vi "DL-SMART-MS-Modify-05-25-7.0.vi"() -> ()   [LabVIEW 2013]
uses:
  <vilib>/Utility/file.llb/Read From Spreadsheet File (DBL).vi
  <userlib>/caLab/Private/CaLabEvent_PV-1D.vi
  <userlib>/caLab/Private/Put_DBL-1D_PV.vi
  <userlib>/caLab/Private/Put_I32_PV.vi
  cal_p.vi
  <userlib>/caLab/Private/Get_PV.vi
  <vilib>/Utility/file.llb/Write To Spreadsheet File (DBL).vi
  <vilib>/vision/driver/NI_Vision_Acquisition_Software.lvlib
  <resource>/objmgr/imaqdx.rc
  <vilib>/Analysis/NI_AALPro.lvlib
panel:
  out "idn status":string
  out "MS":cluster{dbl[], "filtered data":dbl[]}(graph)
  out "std sample":T1(array[cluster])
  in  "Set Laser":bool
  out "Image":T2(plugin-control)
  out "selected id":i32
  out "selected row":i32
  out "currentNO":string
  out "commet":string
  out "sampleID":string
  in  "Shots/Point":i32=100
  in  "chamber in":bool caption="TakeMS"
  in  "chamber out":bool caption="TakeMS"
  in  "Laser parameter":T4
  in  "ADC parameter":T5
  in  "ShutDownSystem":bool
  in  "ADC reference":refnum<vi>
  in  "SetLaserEnergy":dbl(slide) min=0.0 max=50.0 scale=0.0..10.0
  in  "LaserHV":u8=50 min=1 max=100
  in  "频率/Hz":u8=30
  out "Pul.HV-Real":dbl
  out "Identify Spcetrum":cluster{"ID1:X":dbl[], "ID1:Y":dbl[]}[](graph)
  in  "测试记录":i32(listbox)=6
  in  "Identification Results (单靶鉴定结果)":i32(listbox)=2
  in  "HVEnable":bool
  out "GateClose":bool
  out "LaserOK":bool
  out "HV-OK":bool
  out "Vacuum-OK":bool
  in  "Tab Control":T6(tab)
  in  "helix-Zeta-Step":dbl=100.0
  in  "helix-b":dbl=0.2
  in  "AcquireMS-Methods":u8(ring) items=["SinglePoint", "Multipoints", "MultiTar"]
  in  "Thresh":dbl=-0.005 format="%#_13g"
  in  "right rank":i32=2
  in  "left rank":i32=2
  in  "deBaseline":bool
  in  "MCPHV-Set":dbl=1400.0 min=0.0 max=1600.0
  in  "LensHV-Set":dbl=8000.0 min=0.0 max=10000.0
  in  "Tar.HV-Set":dbl=18010.0 min=0.0 max=20000.0
  in  "Pul.HV-Set":dbl=1400.0 min=0.0 max=2000.0
  in  "PulseDelay":dbl
  in  "ADCFreq":dbl
  in  "CH1_Coupling":u64(ring)=2 items=["Volt DC"=1, "Volt AC"=2, "Ampere DC"=4, "Ampere AC"=8, "Ohm"=16]
  in  "Channel 1_Range":dbl(ring)=4.0 items=["80 V"=80.0, "40 V"=40.0, "20 V"=20.0, "8 V"=8.0, "4 V"=4.0, "2 V"=2.0, "800 mV"=0.8, "400 mV"=0.4, "200 mV"=0.2]
  in  "Anal. Setting File":string="High Mass"
  in  "SettingFileSave":bool caption="TakeMS"
  in  "SettingFileAppl":bool caption="TakeMS"
  in  "SettingDel":bool caption="TakeMS"
  in  "RunADC":bool caption="TakeMS"
  out "ADCstatus":bool
  in  "Vac_Prot.":bool
  in  "Turbo_Fore":bool
  in  "Main_Samp":bool
  in  "Samp_Atmos":bool
  in  "Fore_Samp":bool
  in  "StartPump":bool
  in  "SopPump":bool
  out "TurboSpeed":dbl(knob) scale=0.0..100.0
  out "PumpKW":dbl
  out "PumpAmps":dbl
  out "PumpTemp":u16
  out "PumpVolts":dbl
  in  "laser OFF":bool
  in  "laser ON":bool
  out "cluster":T7
  in  "laser Deactive":bool
  out "A1-position-Y":dbl=45.0 caption="Y" min=0.0 max=55.0
  out "A1-position-X":dbl=53.4 caption="X" min=0.0 max=55.0
  in  "GO":bool
  in  "Y":dbl min=0.0 max=55.0
  in  "X":dbl min=0.0 max=55.0
  in  "A1-Position":bool caption="X-"
  in  "Plat_To_Zero":bool caption="TakeMS"
  in  "Plat_Cal":bool caption="TakeMS"
  out "Y当前":dbl
  out "X当前":dbl
  out "移动":bool
  out "Y满":bool
  out "Y标":bool
  out "X满":bool
  out "Y0":bool
  out "X0":bool
  out "靶位In/Out":bool
  out "仓门":bool
  out "Y过热":bool
  out "X过热":bool
  out "通讯":bool
  in  "Operation Record":i32(listbox)
  in  "OptionRecordLoad 2":bool caption="TakeMS"
  in  "OptionRecordClear":bool caption="TakeMS"
  out "c:":dbl
  out "b:":dbl
  out "a:":dbl
  in  "cancel cal":bool
  in  "cal save":bool
  in  "peak cal":bool
  in  "peak detect":bool
  in  "标准样品":u16(ring) items=["肺炎克雷伯菌", "铜绿假单胞菌"]
  in  "定标参数":i32(listbox)
  out "Tar.HV-Real":dbl
  out "LensHV-Real":dbl
  out "MCPHV-Real":dbl
  out "Lvaccum":dbl=0.83 format="%#_2e"
  out "Hvaccum":dbl=3.4e-05 format="%#_2e"
  in  "H12":bool
  in  "G12":bool
  in  "F12":bool
  in  "E12":bool
  in  "D12":bool
  in  "C12":bool
  in  "B12":bool
  in  "A12":bool
  in  "H11":bool
  in  "G11":bool
  in  "F11":bool
  in  "E11":bool
  in  "D11":bool
  in  "C11":bool
  in  "B11":bool
  in  "A11":bool
  in  "H10":bool
  in  "G10":bool
  in  "F10":bool
  in  "E10":bool
  in  "D10":bool
  in  "C10":bool
  in  "B10":bool
  in  "A10":bool
  in  "H9":bool
  in  "G9":bool
  in  "F9":bool
  in  "E9":bool
  in  "D9":bool
  in  "C9":bool
  in  "B9":bool
  in  "A9":bool
  in  "H8":bool
  in  "G8":bool
  in  "F8":bool
  in  "E8":bool
  in  "D8":bool
  in  "C8":bool
  in  "B8":bool
  in  "A8":bool
  in  "H7":bool
  in  "G7":bool
  in  "F7":bool
  in  "E7":bool
  in  "D7":bool
  in  "C7":bool
  in  "B7":bool
  in  "A7":bool
  in  "H6":bool
  in  "G6":bool
  in  "F6":bool
  in  "E6":bool
  in  "D6":bool
  in  "C6":bool
  in  "B6":bool
  in  "A6":bool
  in  "H5":bool
  in  "G5":bool
  in  "F5":bool
  in  "E5":bool
  in  "D5":bool
  in  "C5":bool
  in  "B5":bool
  in  "A5":bool
  in  "H4":bool
  in  "G4":bool
  in  "F4":bool
  in  "E4":bool
  in  "D4":bool
  in  "C4":bool
  in  "B4":bool
  in  "A4":bool
  in  "H3":bool
  in  "G3":bool
  in  "F3":bool
  in  "E3":bool
  in  "D3":bool
  in  "C3":bool
  in  "B3":bool
  in  "A3":bool
  in  "H2":bool
  in  "G2":bool
  in  "F2":bool
  in  "E2":bool
  in  "D2":bool
  in  "C2":bool
  in  "B2":bool
  in  "A2":bool
  in  "H1":bool
  in  "G1":bool
  in  "F1":bool
  in  "E1":bool
  in  "D1":bool
  in  "C1":bool
  in  "B1":bool
  in  "A1":bool
  in  "Clear":bool caption="TakeMS"
  in  "Add":bool caption="TakeMS"
  in  "TakeMS-Stop":bool caption="TakeMS"
  in  "TakeMS-Run":bool caption="TakeMS"
  # "Laser (激光)"
  # "Acq.(采谱)"
  # "Vacuum(真空)"
  # "Pa"
  # "High"
  # "1"
  # "2"
  # "3"
  # "4"
  # "5"
  # "6"
  # "7"
  # "8"
  # "9"
  # "10"
  # "11"
  # "12"
  # "A"
  # "Low"
  # "Pa"
  # "B"
  # "H.V.(高压)"
  # "C"
  # "D"
  # "MCP"
  # "V"
  # "E"
  # "Tar."
  # "V"
  # "F"
  # "Pul."
  # "V"
  # "G"
  # "Lens"
  # "V"
  # "H"
  # "Vauum (真空)"
  # "H.V. (高压)"
  # "Laser (激光)"
  # "Gate (仓门)"
  # "mm"
  # "Radian"
  # "H.V. (高压参数)"
  # "ADC(采集卡设置)"
  # "ADCFreq(采样)"
  # "MCP (探测器)"
  # "V"
  # "Hz"
  # "Tar. (靶)"
  # "V"
  # "Setting File(设置文件)"
  # "Coupling"
  # "Pulse (脉冲)"
  # "V"
  # "IntRange"
  # "V"
  # "Lens (透镜)"
  # "Delay (延时)"
  # "ns"
  # "Sole. Valves"
  # "Turbo Pump"
  # "自锁保护"
  # "机械/分子"
  # "主仓/样仓"
  # "样仓/大气"
  # "机械/样仓"
  # "激光器状态"
  # "mm"
  # "mm"
  # "mm"
  # "mm"
  # "mm"
  # "mm"
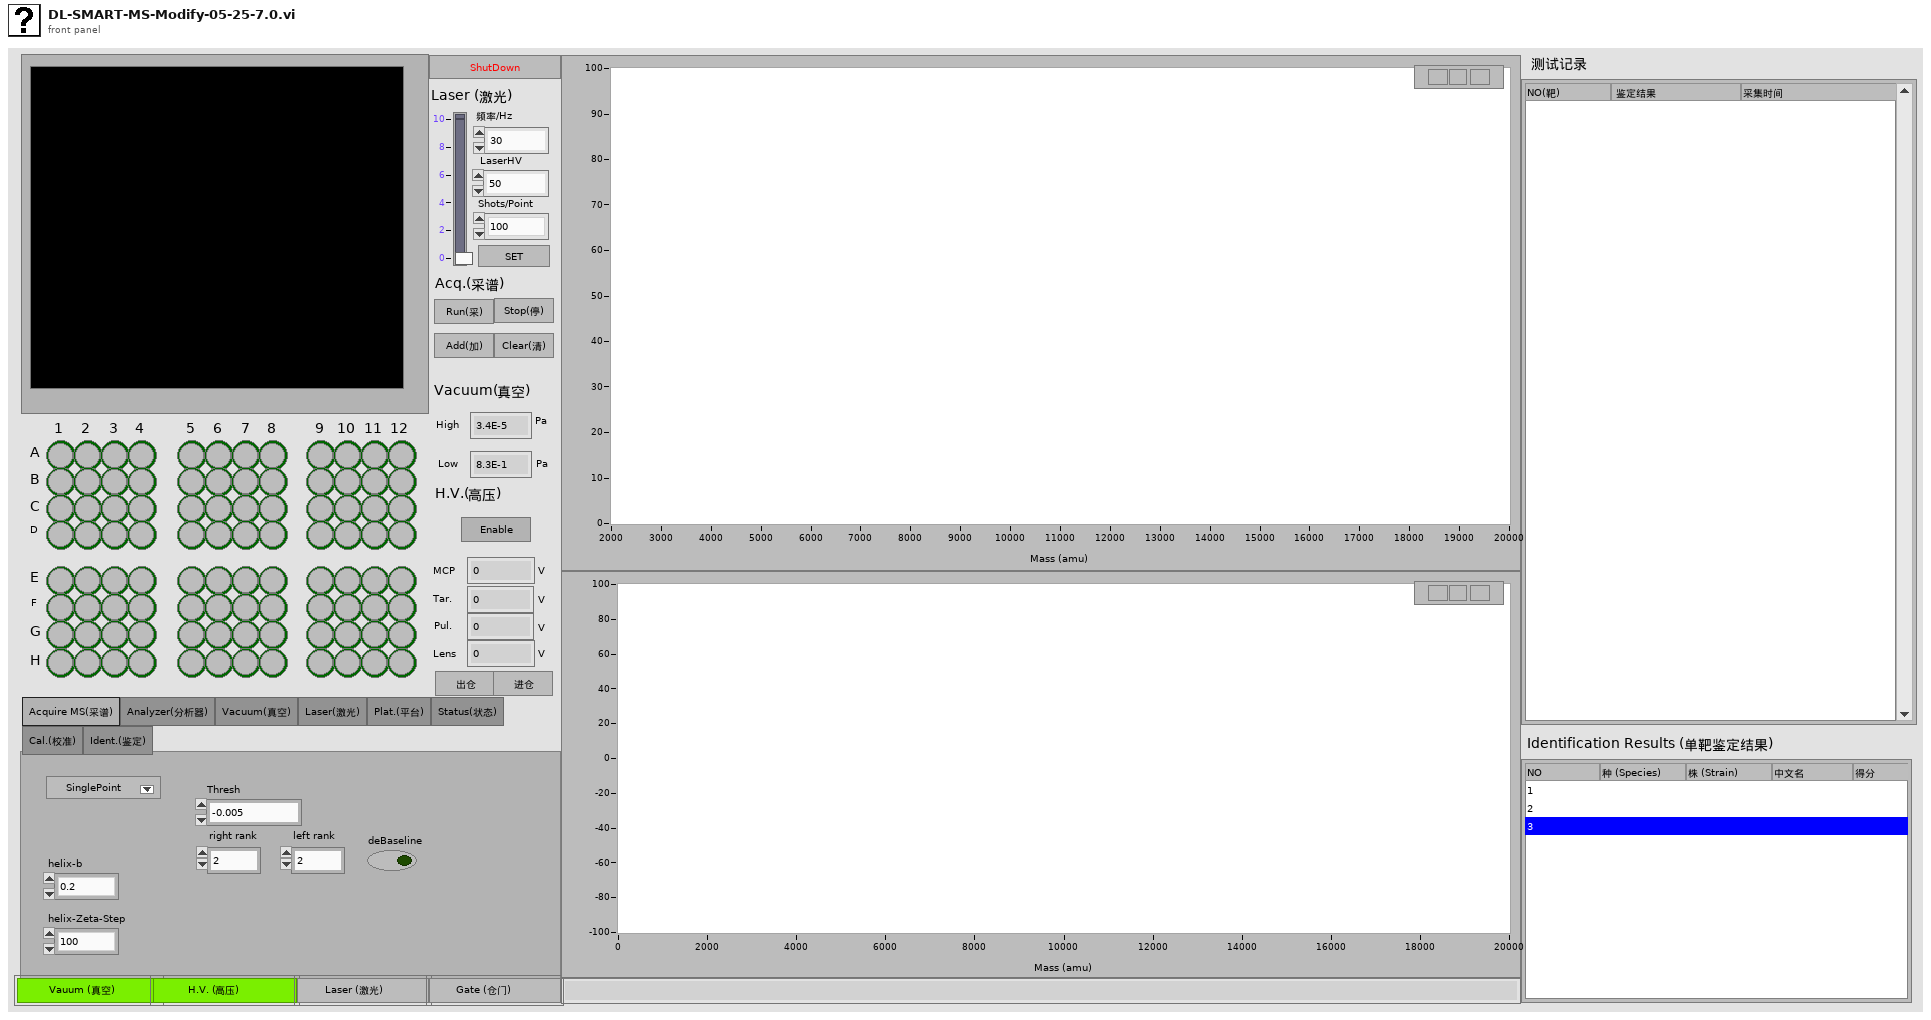
[diagram p1: front panel]
types:
  T1 = cluster{"name":string, "mz":dbl[], "time":dbl[]}[]
  T2 = typedef "IMAQ Image.ctl" = refnum<image>
  T3 = typedef "Semaphore RefNum" = refnum<k1>
  T4 = cluster{"VISA resource name":refnum<visa-resource-name>, "standby":bool, "semaphore in":T3, "SetLaserEnergy":dbl}
  T5 = cluster{"TpDeviceHandle_t":u32, "Record Length/Samples":u64, "ShotsPerPoint":u16}
  T6 = enum32{"Acquire MS(采谱)", "Analyzer(分析器)", "Vacuum(真空)", "Laser(激光)", "Plat.(平台)", "Status(状态)", "Cal.(校准)", "Ident.(鉴定)"}
  T7 = cluster{"链接":bool, "待机":bool, "发射":bool, "[3]":bool, "内存":bool, "测能":bool, "温警":bool, "静态":bool, "操作":bool}
  T8 = cluster{"tag1":string, "tag2":string, "x":dbl[], "y":dbl[], "ID1:X":dbl[], "ID1:Y":dbl[], "ID1:REF:X":dbl[], "ID1:REF:Y":dbl[], "ID2:X":dbl[], "ID2:Y":dbl[], "ID2:REF:X":dbl[], "ID2:REF:Y":dbl[], "ID3:X":dbl[], "ID3:Y":dbl[], "ID3:REF:X":dbl[], "ID3:REF:Y":dbl[], "ID1:TAG1":string, "ID1:TAG2":string, "ID2:TAG1":string, "ID2:TAG2":string, "ID3:TAG1":string, "ID3:TAG2":string, "ID1:NAME":string, "ID2:NAME":string, "ID3:NAME":string, "ID1:SCORE":string, "ID2:SCORE":string, "ID3:SCORE":string, "NO":string}[]
  T9 = cluster{"laser semaphore":T3, "pump semaphore":T3}
  T10 = enum8{"Enabled", "Disabled", "Disabled and Grayed Out"}
  T11 = cluster{"tag1":string, "tag2":string, "x":dbl[], "y":dbl[], "ID1:X":dbl[], "ID1:Y":dbl[], "ID1:REF:X":dbl[], "ID1:REF:Y":dbl[], "ID2:X":dbl[], "ID2:Y":dbl[], "ID2:REF:X":dbl[], "ID2:REF:Y":dbl[], "ID3:X":dbl[], "ID3:Y":dbl[], "ID3:REF:X":dbl[], "ID3:REF:Y":dbl[], "ID1:TAG1":string, "ID1:TAG2":string, "ID2:TAG1":string, "ID2:TAG2":string, "ID3:TAG1":string, "ID3:TAG2":string, "ID1:NAME":string, "ID2:NAME":string, "ID3:NAME":string, "ID1:SCORE":string, "ID2:SCORE":string, "ID3:SCORE":string, "NO":string}
  T12 = cluster{"monitor":refnum<user-event>, "motor status":refnum<user-event>, "motor":refnum<user-event>, "notifier out":refnum<notifier>, "queue out":refnum<queue>, "AI":T3, "DI":T3, "CX":T3, "CY":T3}
  T13 = cluster{"AI Task":refnum<k21>, "AO Task":refnum<k21>, "DO Task":refnum<k21>, "DI Task":refnum<k21>, "PWM x":refnum<k21>, "PWM y":refnum<k21>, "counter x":refnum<k21>, "counter y":refnum<k21>}
  T14 = cluster{"tasks":cluster{"AI Task":refnum<k21>, "AO Task":refnum<k21>, "DO Task":refnum<k21>, "DI Task":refnum<k21>, "PWM x":refnum<k21>, "PWM y":refnum<k21>, "counter x":refnum<k21>, "counter y":refnum<k21>}, "interface":cluster{"monitor":refnum<user-event>, "motor status":refnum<user-event>, "motor":refnum<user-event>, "notifier out":refnum<notifier>, "queue out":refnum<queue>, "AI":T3, "DI":T3, "CX":T3, "CY":T3}, "error out":errorcluster}
  T15 = cluster{"ConfiguredPumpCom":refnum<visa-resource-name>, "ConfiguredLaserCom":refnum<visa-resource-name>}
  T16 = typedef "LVPoint32TypeDef.ctl" = cluster{"Horizontal":i32, "Vertical":i32}
  T17 = typedef "LVRowAndColumnTypeDef.ctl" = cluster{"Row":i32, "Column":i32}
  T18 = cluster{"Type":u32, "Version":u32, "Flags":u32, "SerialNumberHigh":u32, "SerialNumberLow":u32, "BusType":u32, "InterfaceName":string, "VendorName":string, "ModelName":string, "CameraFileName":string, "CameraAttributeURL":string}[]
  T19 = cluster{"Type":u32, "Version":u32, "Flags":u32, "SerialNumberHigh":u32, "SerialNumberLow":u32, "BusType":u32, "InterfaceName":string, "VendorName":string, "ModelName":string, "CameraFileName":string, "CameraAttributeURL":string}
  T20 = typedef "IMAQdx.ctl" = refnum<k21>
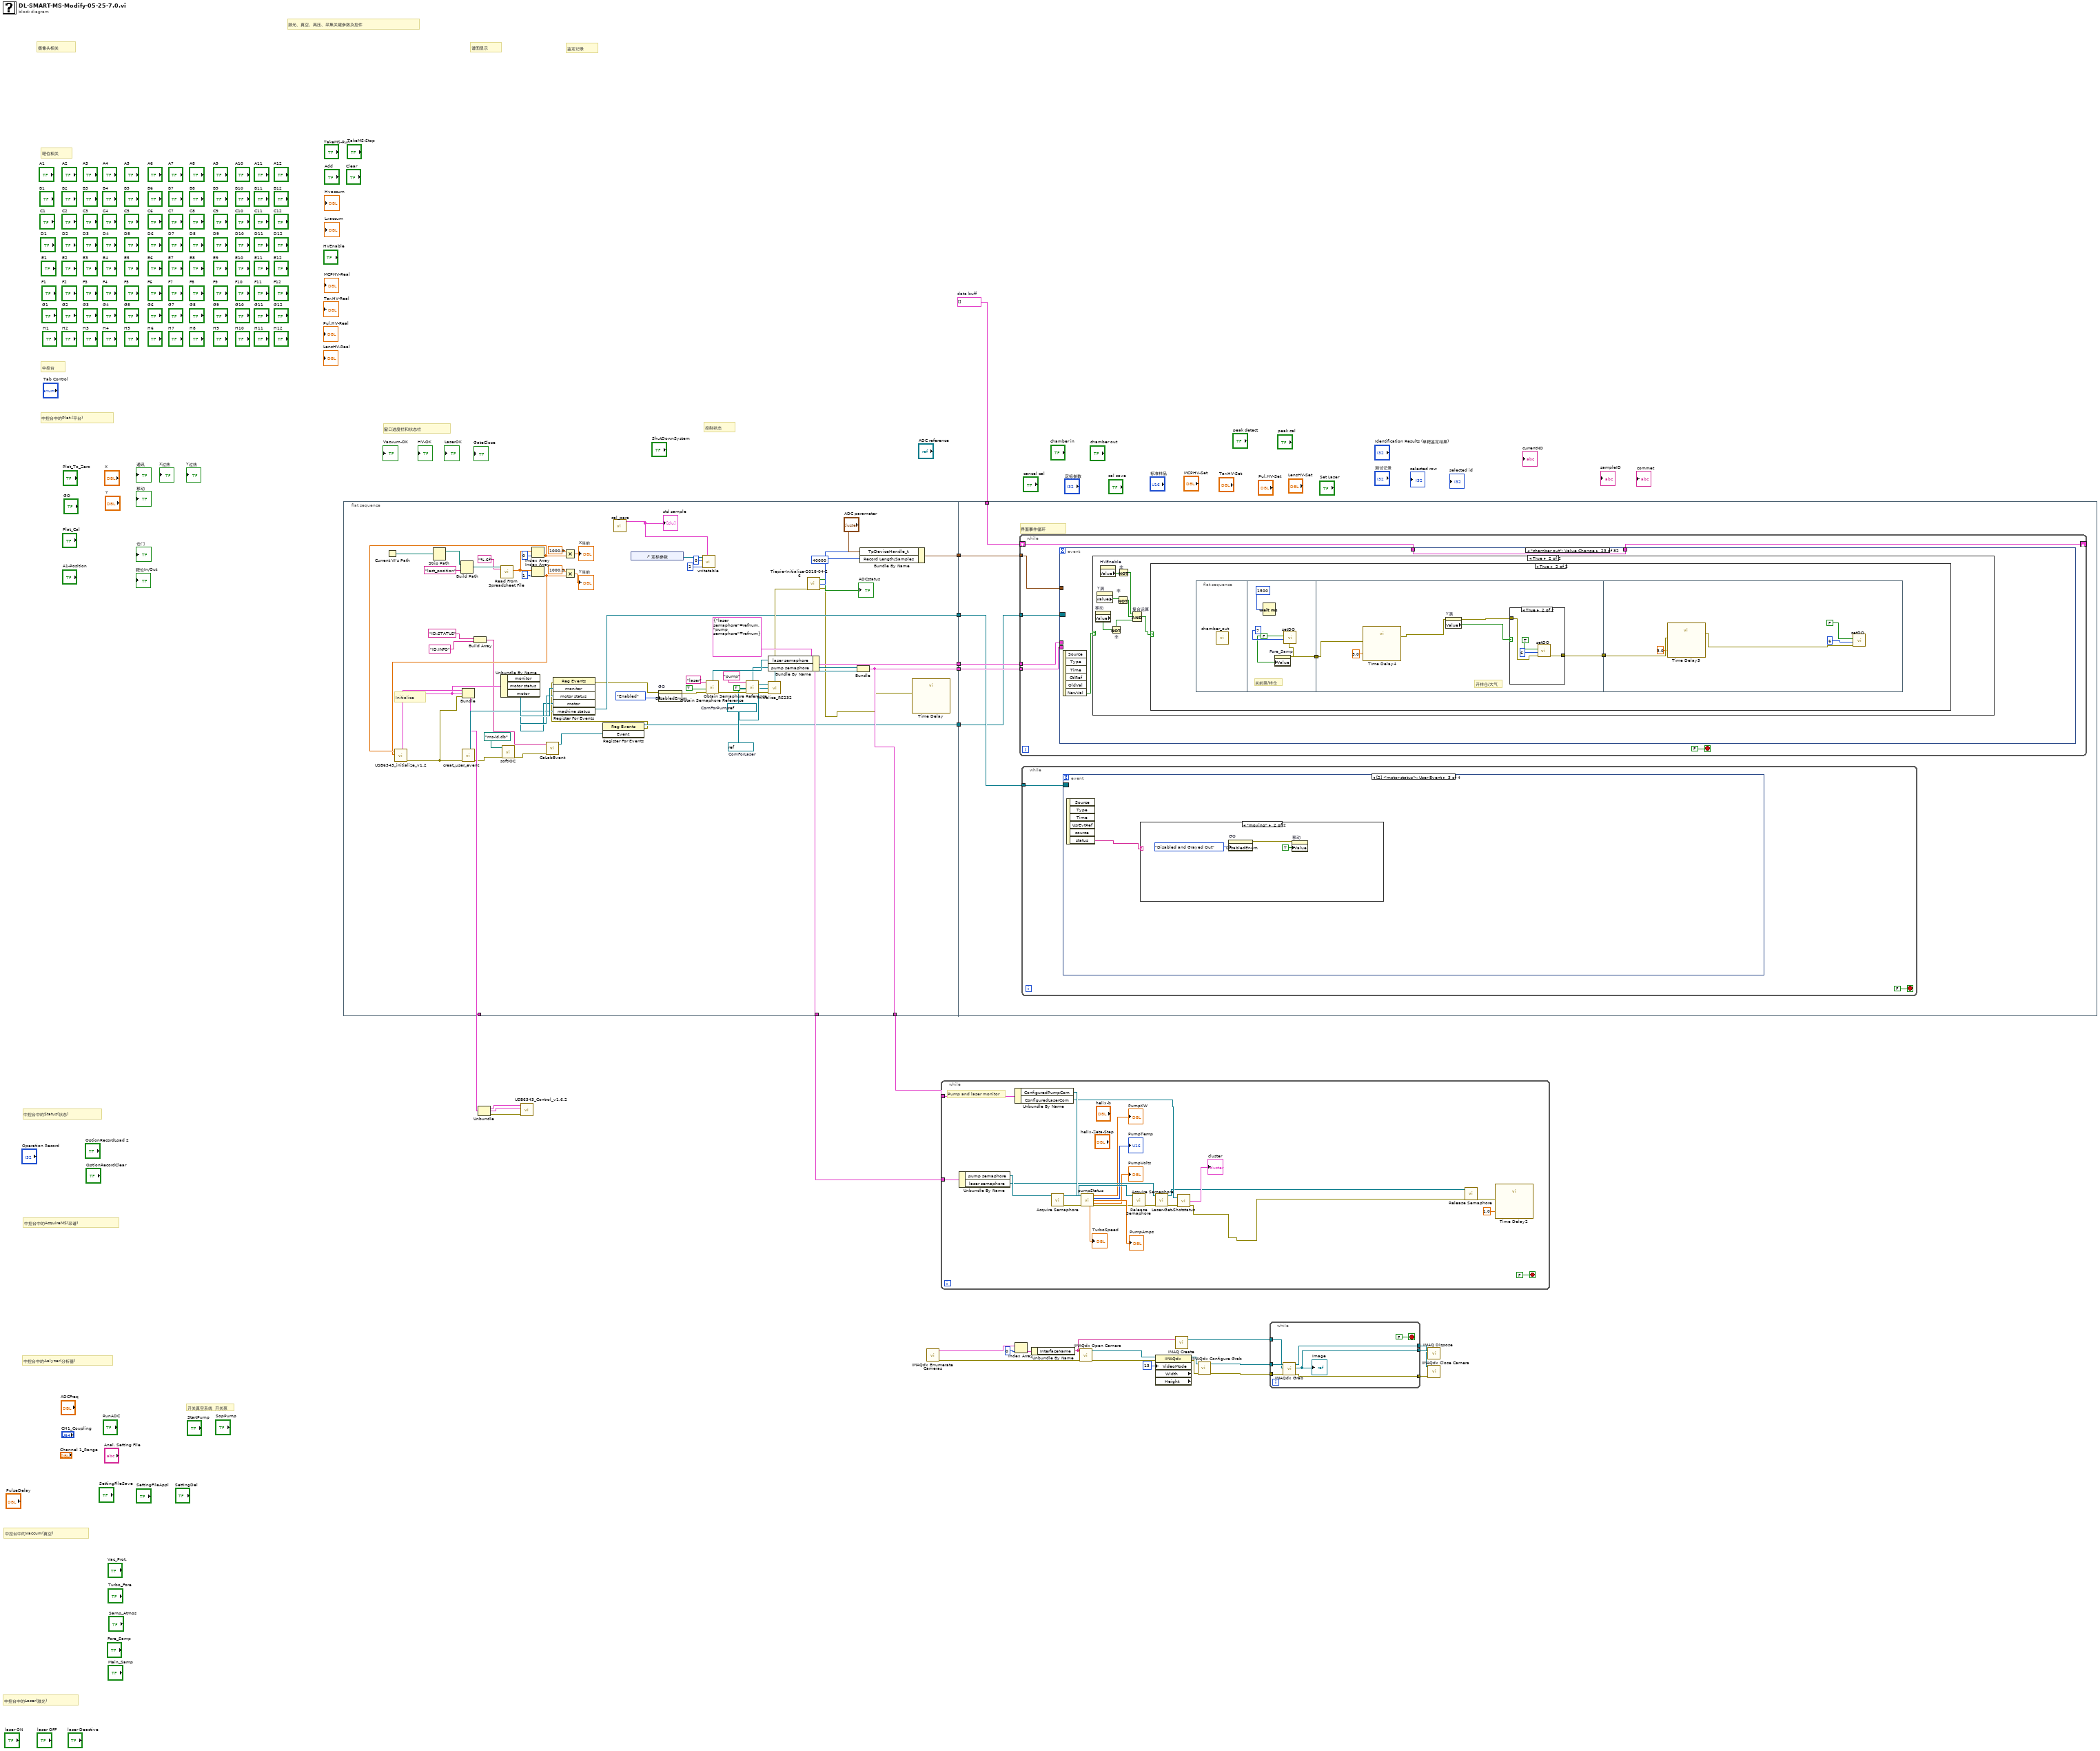
[diagram p0: block diagram]
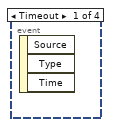
[diagram p2: hidden frame]
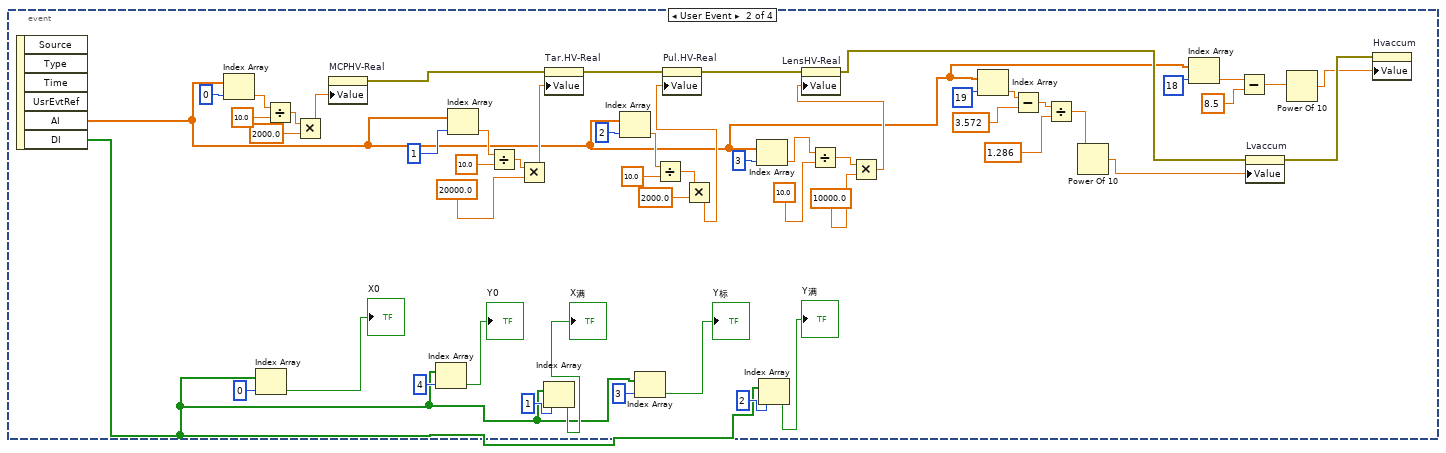
[diagram p3: hidden frame]
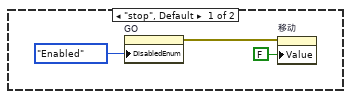
[diagram p4: hidden frame]
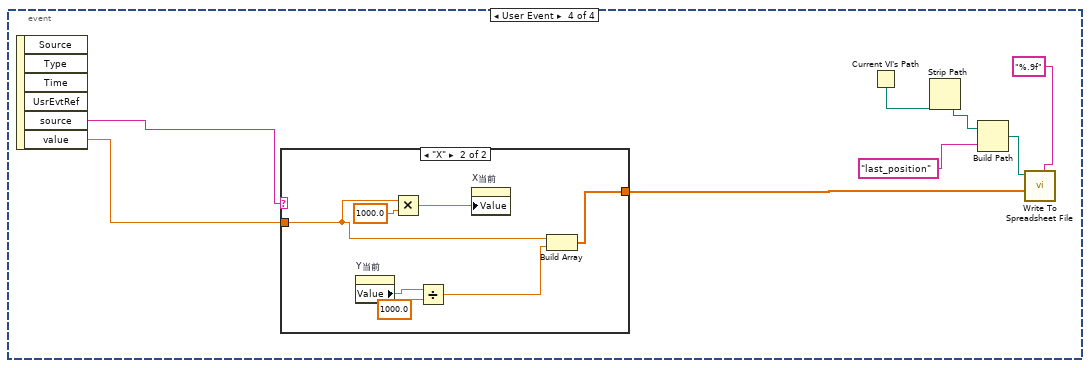
[diagram p5: hidden frame]
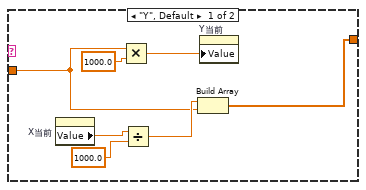
[diagram p6: hidden frame]
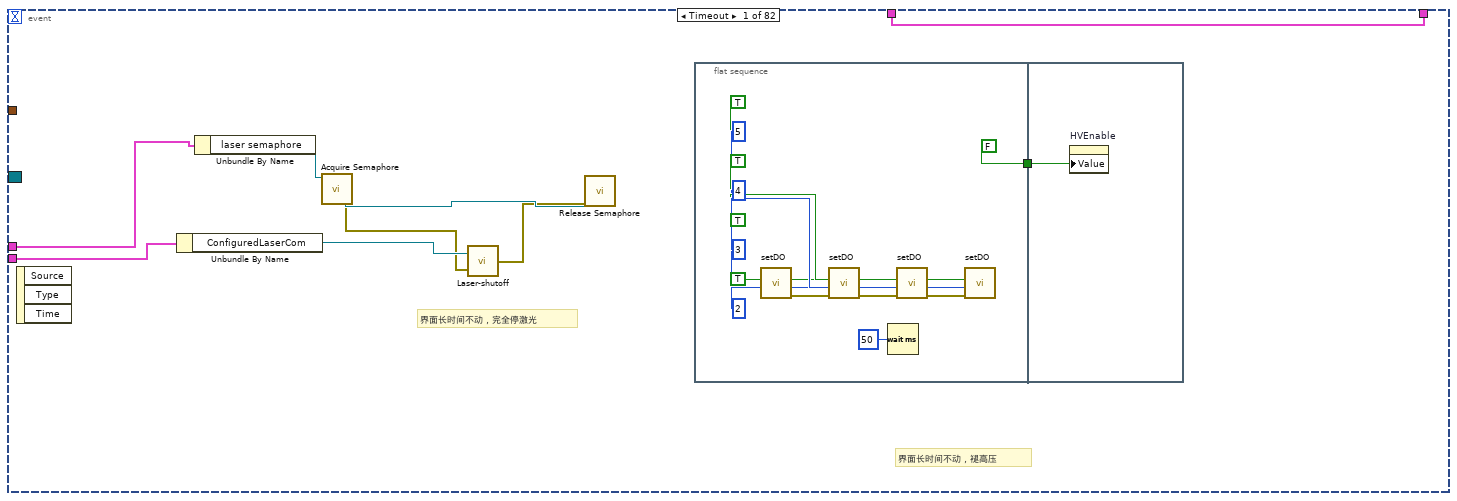
[diagram p7: hidden frame]
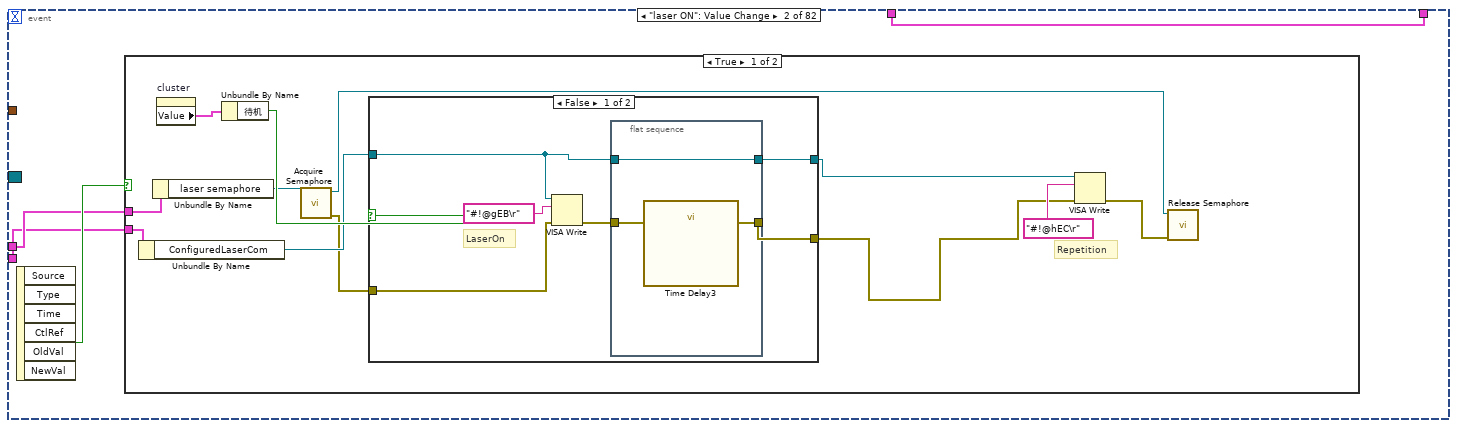
[diagram p8: hidden frame]
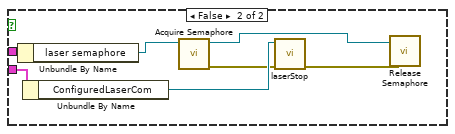
[diagram p10: hidden frame]
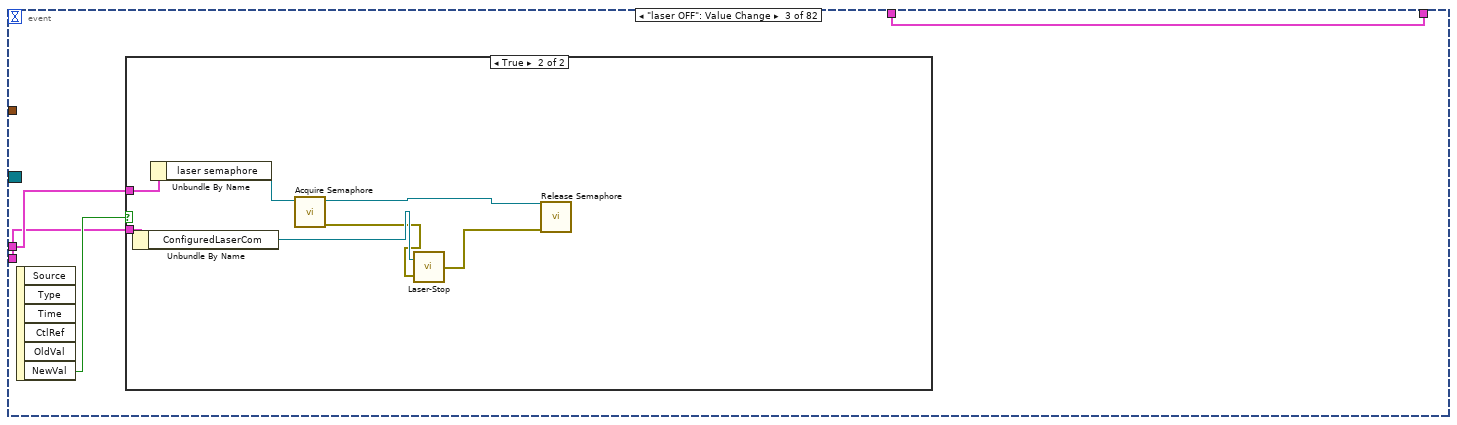
[diagram p11: hidden frame]
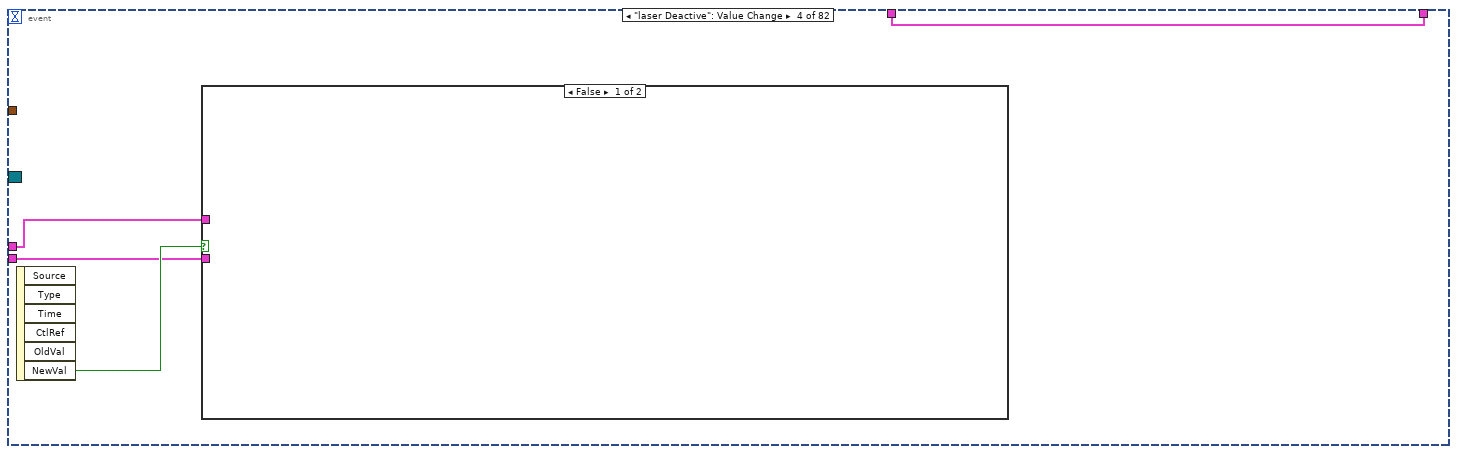
[diagram p13: hidden frame]
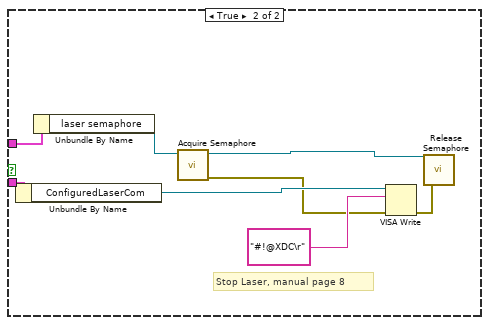
[diagram p14: hidden frame]
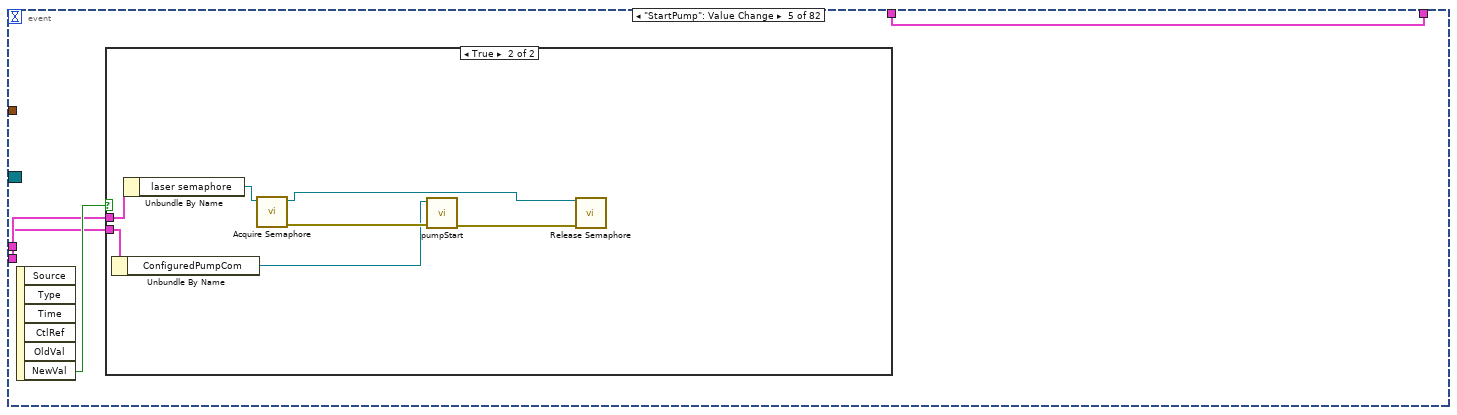
[diagram p15: hidden frame]
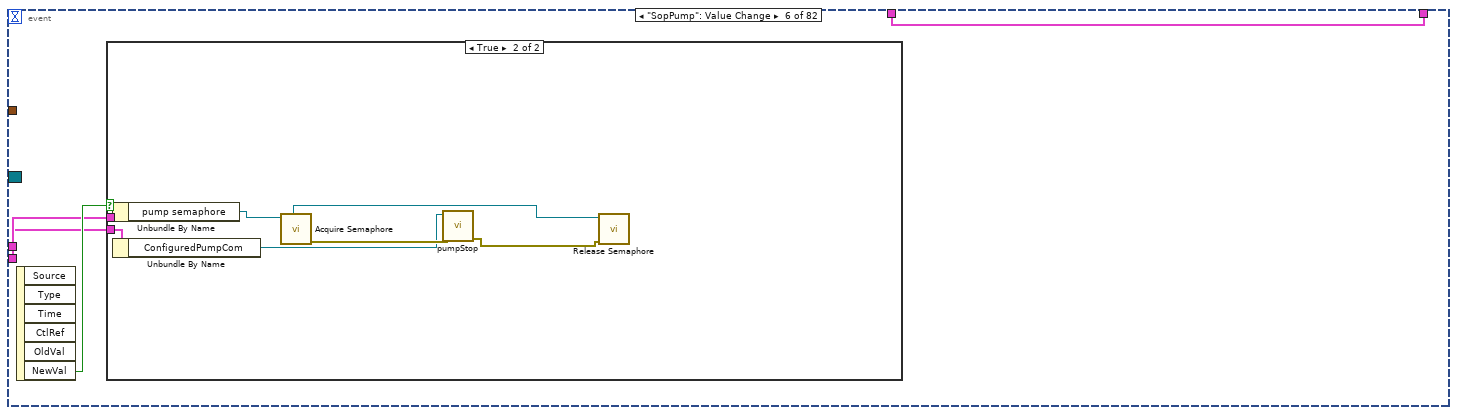
[diagram p17: hidden frame]
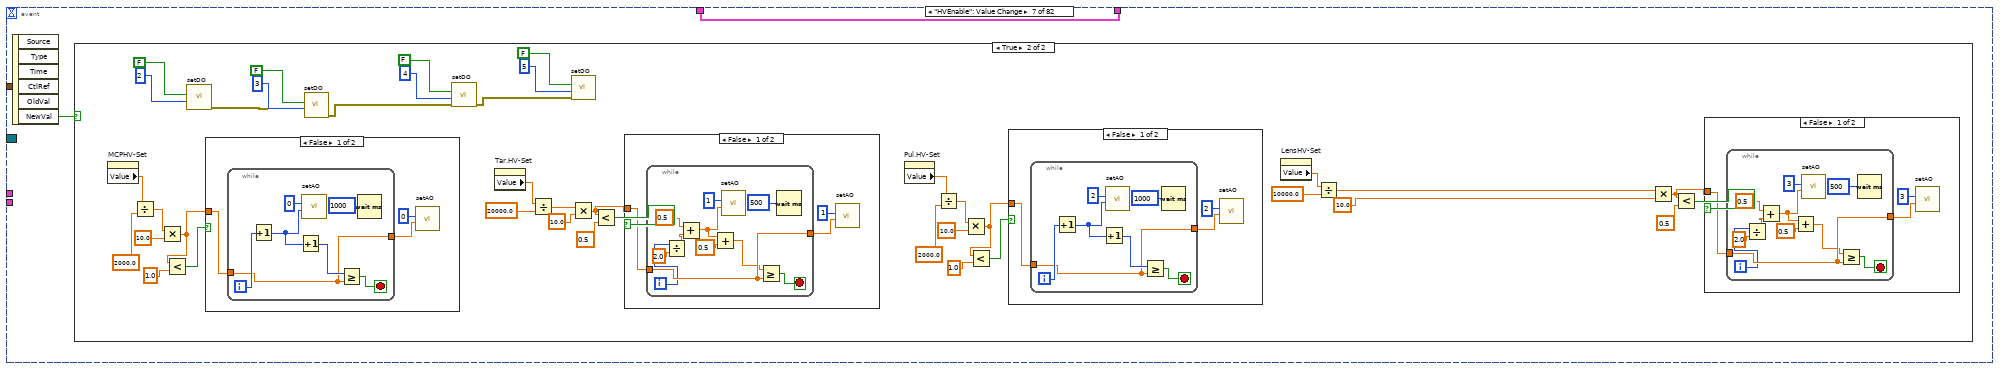
[diagram p19: hidden frame]
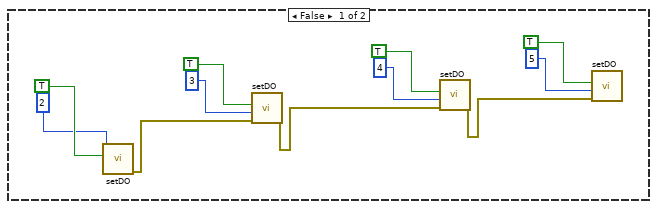
[diagram p20: hidden frame]
diagram:
  w21 = T8 []  # data buff
  # "Pump and laser monitor"
  # "开关真空系统  开关泵"
  # "控制状态"
  # "鉴定记录"
  # "谱图显示"
  # "激光、真空、高压、采集关键参数及控件"
  # "窗口进度栏和状态栏"
  # "中控台中的Laser(激光)"
  # "中控台中的Vaccum(真空)"
  # "中控台中的Aalyzer(分析器)"
  # "中控台中的AcquireMS(采谱)"
  # "中控台中的Status(状态)"
  # "中控台中的Plat.(平台)"
  # "中控台"
  # "靶位相关"
  # "摄像头相关"
  n1 = flat-sequence {
    tunnel: [w43] -> w28
    tunnel: [w68] -> w27
    tunnel: [w68] -> w25
    tunnel: [w67] -> w26
    tunnel: [w67] -> w24
    tunnel: [w71] -> w23
    tunnel: [w60] -> w22
    tunnel: [w30] -> w1
    tunnel: w28 -> [w91]
    tunnel: w27 -> [w95]
    tunnel: w26 -> [w94]
    tunnel: w22 -> [w93]
    tunnel: w21 -> [w92]
    tunnel: w1 -> [w90]
    frame #0 {
      w65 = refnum<visa-resource-name> "COM9"  # ComForLaser
      w66 = refnum<visa-resource-name> "COM10"  # ComForPump
      # "Initialize"
      n2 = Current VI's Path() -> (path=w58:path)
      n3 = Strip Path(path=w58) -> (stripped path=w57:path)  [unwired: 1 out]
      n4 = Build Path(base path=w57, name or relative path="last_position") -> (appended path=w55:path)
      n5 = Build Array("ID:STATUS", "ID:INFO") -> (w32:string[])
      n6 = call-poly <vilib>:"Read From Spreadsheet File.vi"("format (%.3f)"="%.6f", "file path (dialog if empty)"=w55) -> ("first row"=w53:dbl[])  [unwired: 5 in, 4 out]
      n7 = Index Array(array=w53, index=0) -> (element=w50:dbl)
      n8 = Index Array(array=w53, index=1) -> (element=w47:dbl)
      n9 = call "USB6343_initialize_v1.2.vi"("Y initial position"=w47, "X initial position"=w50) -> ("error out"=w72:errorcluster, "interface"=w73:T12, "tasks"=w74:T13)  [unwired: 7 in]
      n10 = Bundle("tasks"=w74, "interface"=w73, "error out"=w72) -> (w71:T14)  [unwired: 1 in]
      n11 = call "creat_user_event.vi"("error in (no error)"=w72) -> ("error out"=w40:errorcluster, "machine status"=w82:refnum<user-event>)  [unwired: 9 in]
      n12 = Unbundle By Name(w73) -> ("monitor"=w89:refnum<user-event>, "motor status"=w88:refnum<user-event>, "motor"=w87:refnum<user-event>)
      n13 = call "softIOC.vi"("error in (no error)"=w40, "路径"=path "ms-id.db") -> ("error out"=w41:errorcluster)  [unwired: 8 in, 1 out]
      n14 = call-poly <userlib>:"CaLabEvent.vi"("error in (no error)"=w41, "PV Names"=w32) -> ("Event"=w31:refnum<user-event>)  [unwired: 7 in, 2 out]
      n15 = Multiply(x=1000.0, y=w50) -> (x*y=→"X当前":dbl)
      n16 = Multiply(x=1000.0, y=w47) -> (x*y=→"Y当前":dbl)
      n17 = register-events(w31) -> (reference out=w30:refnum<event-registration>, error out=w29:errorcluster)  [unwired: 2 in]
      n18 = register-events(error in=w29, w89, w88, w87, w82) -> (reference out=w43:refnum<event-registration>, error out=w39:errorcluster)  [unwired: 1 in]
      n19 = call "cal_para.vi"() -> ("std sample"=w36:T1)  [unwired: 11 in]
      "std sample" <- w36
      n20 = control-ref of="定标参数"() -> (w38:refnum<vi>)
      n21 = property on="GO" class="Bool (strict)"(error in=w39, "DisabledEnum"=T10."Enabled" ("Disabled")) -> (error out=w83:errorcluster)  [unwired: 1 in, 1 out]
      n22 = call "writetable.vi"("std sample"=w36, "col"=2, "type"=0, "reference"=w38) -> ()  [unwired: 8 in]
      n23 = call <vilib>:"Obtain Semaphore Reference.vi"("error in (no error)"=w83, "create if not found (T)"=TRUE, "name (unnamed)"="laser") -> ("error out"=w78:errorcluster, "semaphore"=w75:T3)  [unwired: 2 in, 1 out]
      n24 = call <vilib>:"Obtain Semaphore Reference.vi"("error in (no error)"=w78, "create if not found (T)"=TRUE, "name (unnamed)"="pump") -> ("error out"=w77:errorcluster, "semaphore"=w69:T3)  [unwired: 2 in, 1 out]
      n25 = Bundle By Name(cluster=T9 {"laser semaphore"=refnum, "pump semaphore"=refnum}, "laser semaphore"=w75, "pump semaphore"=w69) -> (w68:T9)
      n26 = call "Initialize_RS232.vi"("error in (no error)"=w77, "ComForLaser"=w65, "ComForPump"=w66) -> ("error out"=w64:errorcluster, "ConfiguredLaserCom"=w80:refnum<visa-resource-name>, "ConfiguredPumpCom"=w81:refnum<visa-resource-name>)
      n27 = call "Tiepie-Initialize-2018-04-26.vi"("error in (no error)"=w64) -> ("error out"=w42:errorcluster, "TpDeviceHandle_t"=w62:u32, "Card-OK"=→"ADCstatus":bool)  [unwired: 3 in]
      n28 = Bundle("ConfiguredPumpCom"=w81, "ConfiguredLaserCom"=w80) -> (w67:T15)  [unwired: 1 in]
      n29 = Bundle By Name(cluster="ADC parameter", "TpDeviceHandle_t"=w62, "Record Length/Samples"=u64 40000) -> (w60:T5)
      n30 = call "Time Delay"("error in (no error)"=w42) -> ()  [unwired: 10 in, 1 out]
    }
    frame #1 {
      # "界面事件循环"
      n31 = while {
        tunnel: w90 -> [w186]
        tunnel: w94 -> [w185]
        tunnel: w95 -> [w184]
        tunnel: w93 -> [w182]
        shift-right: [w180] -> _
        shift-left: w92 -> [w181]
        stop <- FALSE stop-if-true
        n32 = event shown="[22] \"chamber out\": Value Change" {
          selector: w186 -> [_ _ _ _ _ _ _ _ _ _ _ _ _ _ _ _ _ _ _ _ _ _ _ _ _ _ _ _ _ _ _ _ _ _ _ _ _ _ _ _ _ _ _ _ _ _ _ _ _ _ _ _ _ _ _ _ _ _ _ _ _ _ _ _ _ _ _ _ _ _ _ _ _ _ _ _ _ _ _ _ _ _]
          dyn-events: _ -> [_ _ _ _ _ _ _ _ _ _ _ _ _ _ _ _ _ _ _ _ _ _ _ _ _ _ _ _ _ _ _ _ _ _ _ _ _ _ _ _ _ _ _ _ _ _ _ _ _ _ _ _ _ _ _ _ _ _ _ _ _ _ _ _ _ _ _ _ _ _ _ _ _ _ _ _ _ _ _ _ _ _]
          timeout: _ -> [_ _ _ _ _ _ _ _ _ _ _ _ _ _ _ _ _ _ _ _ _ _ _ _ _ _ _ _ _ _ _ _ _ _ _ _ _ _ _ _ _ _ _ _ _ _ _ _ _ _ _ _ _ _ _ _ _ _ _ _ _ _ _ _ _ _ _ _ _ _ _ _ _ _ _ _ _ _ _ _ _ _]
          tunnel: w185 -> [w189 w211 w244 w255 w267 w278 _ _ _ _ _ _ _ _ w473 w524 _ _ _ _ _ _ _ _ _ _ _ _ _ _ _ _ _ _ _ _ _ _ _ _ _ _ _ _ _ _ _ _ _ _ _ _ _ _ _ _ _ _ _ _ _ _ _ _ _ _ _ _ _ _ _ _ _ _ _ _ _ _ _ _ _ w1761]
          tunnel: w184 -> [w190 w212 w245 w254 w268 w279 _ _ _ _ _ _ _ _ w474 w525 _ _ _ _ _ _ _ _ _ _ _ _ _ _ _ _ _ _ _ _ _ _ _ _ _ _ _ _ _ _ _ _ _ _ _ _ _ _ _ _ _ _ _ _ _ _ _ _ _ _ _ _ _ _ _ _ _ _ _ _ _ _ _ _ _ _]
          tunnel: w182 -> [_ _ _ _ _ _ _ _ _ _ _ _ _ _ w475 _ _ _ _ _ _ _ _ _ _ _ _ _ _ _ _ _ _ _ _ _ _ _ _ _ _ _ _ _ _ _ _ _ _ _ _ _ _ _ _ _ _ _ _ _ _ _ _ _ _ _ _ _ _ _ _ _ _ _ _ _ _ _ _ _ _ _]
          tunnel: w181 -> [w187 w210 w243 w257 w266 w277 w288 w396 w411 w426 w433 w440 w447 w456 w472 w527 w539 w569 w604 w643 w645 w652 w687 w722 w724 w763 w768 w784 w802 w819 w836 w853 w870 w889 w914 w931 w948 w965 w982 w999 w1018 w1037 w1056 w1075 w1094 w1112 w1130 w1148 w1166 w1184 w1202 w1220 w1238 w1256 w1274 w1292 w1310 w1328 w1346 w1364 w1382 w1400 w1418 w1436 w1454 w1472 w1490 w1508 w1526 w1544 w1566 w1584 w1602 w1620 w1638 w1656 w1674 w1692 w1710 w1728 w1746 w1760]
          tunnel: [w187 w210 w243 w257 w266 w277 w288 w396 w411 w426 w433 w440 w447 w456 w471 w527 w538 w569 w604 w643 w645 w652 w687 w722 w724 w763 w768 w784 w802 w819 w836 w853 w870 w888 w914 w931 w948 w965 w982 w999 w1018 w1037 w1056 w1075 w1094 w1112 w1130 w1148 w1166 w1184 w1202 w1220 w1238 w1256 w1274 w1292 w1310 w1328 w1346 w1364 w1382 w1400 w1418 w1436 w1454 w1472 w1490 w1508 w1526 w1544 w1566 w1584 w1602 w1620 w1638 w1656 w1674 w1692 w1710 w1728 w1746 w1760] -> w180
          event Timeout {
            # "界面长时间不动，褪高压"
            # "界面长时间不动，完全停激光"
            n33 = event-data() -> ()  [unwired: 1 in, 3 out]
            n34 = Unbundle By Name(w189) -> ("ConfiguredLaserCom"=w193:refnum<visa-resource-name>)
            n35 = Unbundle By Name(w190) -> ("laser semaphore"=w195:T3)
            n36 = call <vilib>:"Acquire Semaphore.vi"("semaphore"=w195) -> ("error out"=w192:errorcluster, "semaphore out"=w194:T3)  [unwired: 4 in, 1 out]
            n37 = call "Laser-shutoff.vi"("error in (no error)"=w192, "VISA resource name"=w193) -> ("error out"=w191:errorcluster)
            n38 = call <vilib>:"Release Semaphore.vi"("error in (no error)"=w191, "semaphore"=w194) -> ()  [unwired: 4 in, 2 out]
            n39 = flat-sequence {
              tunnel: [FALSE ("HVEnable")] -> w188
              tunnel: w188 -> [w209]
              frame #0 {
                n40 = call "setDO.vi"("channel"=2, "on/off"=TRUE) -> ("错误输出"=w206:errorcluster)  [unwired: 9 in]
                n41 = call "setDO.vi"("错误输入（无错误）"=w206, "channel"=3, "on/off"=TRUE) -> ("错误输出"=w207:errorcluster)  [unwired: 8 in]
                n42 = Wait (ms)(milliseconds to wait=u32 50) -> ()  [unwired: 1 out]
                n43 = call "setDO.vi"("错误输入（无错误）"=w207, "channel"=4, "on/off"=TRUE) -> ("错误输出"=w208:errorcluster)  [unwired: 8 in]
                n44 = call "setDO.vi"("错误输入（无错误）"=w208, "channel"=5, "on/off"=TRUE) -> ()  [unwired: 8 in, 1 out]
              }
              frame #1 {
                n45 = property on="HVEnable" class="Bool (strict)"("Value"=w209) -> ()  [unwired: 2 in, 2 out]
              }
            }
          }
          event "laser ON": Value Change {
            n46 = event-data() -> ("NewVal"=w213:bool)  [unwired: 1 in, 5 out]
            n47 = case shown="True" w213 {
              tunnel: w212 -> [w225 w242]
              tunnel: w211 -> [w224 w240]
              frame True {
                # "Repetition"
                n48 = Unbundle By Name(w224) -> ("ConfiguredLaserCom"=w221:refnum<visa-resource-name>)
                n49 = Unbundle By Name(w225) -> ("laser semaphore"=w216:T3)
                n50 = property on="cluster" class="Clust (strict)"() -> ("Value"=w223:T7)  [unwired: 2 in, 2 out]
                n51 = Unbundle By Name(w223) -> ("待机"=w222:bool)
                n52 = call <vilib>:"Acquire Semaphore.vi"("semaphore"=w216) -> ("error out"=w214:errorcluster, "semaphore out"=w215:T3)  [unwired: 4 in, 1 out]
                n53 = case shown="False" w222 {
                  tunnel: w221 -> [w230 w235]
                  tunnel: [w229 w235] -> w218
                  tunnel: [w227 w234] -> w217
                  tunnel: w214 -> [w226 w234]
                  frame False {
                    # "LaserOn"
                    n54 = VISA Write(VISA resource name=w230, write buffer="#!@gEB\r", error in (no error)=w226) -> (error out=w228:errorcluster)  [unwired: 2 out]
                    n55 = flat-sequence {
                      tunnel: w228 -> [w233]
                      tunnel: [w233] -> w227
                      tunnel: w230 -> [w232]
                      tunnel: [w232] -> w229
                      frame #0 {
                        n56 = call "Time Delay3"() -> ()  [unwired: 11 in, 1 out]
                      }
                    }
                  }
                  frame True {
                  }
                }
                n57 = VISA Write(VISA resource name=w218, write buffer="#!@hEC\r", error in (no error)=w217) -> (error out=w219:errorcluster)  [unwired: 2 out]
                n58 = call <vilib>:"Release Semaphore.vi"("error in (no error)"=w219, "semaphore"=w215) -> ()  [unwired: 4 in, 2 out]
              }
              frame False {
                n59 = Unbundle By Name(w242) -> ("laser semaphore"=w241:T3)
                n60 = Unbundle By Name(w240) -> ("ConfiguredLaserCom"=w239:refnum<visa-resource-name>)
                n61 = call <vilib>:"Acquire Semaphore.vi"("semaphore"=w241) -> ("error out"=w238:errorcluster, "semaphore out"=w236:T3)  [unwired: 4 in, 1 out]
                n62 = call "laserStop.vi"("error in (no error)"=w238, "VISA resource name"=w239) -> ("error out"=w237:errorcluster)  [unwired: 9 in]
                n63 = call <vilib>:"Release Semaphore.vi"("error in (no error)"=w237, "semaphore"=w236) -> ()  [unwired: 4 in, 2 out]
              }
            }
          }
          event "laser OFF": Value Change {
            n64 = event-data() -> ("NewVal"=w246:bool)  [unwired: 1 in, 5 out]
            n65 = case shown="True" w246 {
              tunnel: w245 -> [_ w253]
              tunnel: w244 -> [_ w251]
              frame False {
              }
              frame True {
                n66 = Unbundle By Name(w251) -> ("ConfiguredLaserCom"=w249:refnum<visa-resource-name>)
                n67 = Unbundle By Name(w253) -> ("laser semaphore"=w252:T3)
                n68 = call <vilib>:"Acquire Semaphore.vi"("semaphore"=w252) -> ("error out"=w248:errorcluster, "semaphore out"=w250:T3)  [unwired: 4 in, 1 out]
                n69 = call "Laser-Stop.vi"("error in (no error)"=w248, "VISA resource name"=w249) -> ("error out"=w247:errorcluster)
                n70 = call <vilib>:"Release Semaphore.vi"("error in (no error)"=w247, "semaphore"=w250) -> ()  [unwired: 4 in, 2 out]
              }
            }
          }
          event "laser Deactive": Value Change {
            n71 = event-data() -> ("NewVal"=w256:bool)  [unwired: 1 in, 5 out]
            n72 = case shown="False" w256 {
              tunnel: w254 -> [_ w265]
              tunnel: w255 -> [_ w263]
              frame False {
              }
              frame True {
                # "Stop Laser, manual page 8"
                n73 = Unbundle By Name(w263) -> ("ConfiguredLaserCom"=w260:refnum<visa-resource-name>)
                n74 = Unbundle By Name(w265) -> ("laser semaphore"=w264:T3)
                n75 = call <vilib>:"Acquire Semaphore.vi"("semaphore"=w264) -> ("error out"=w259:errorcluster, "semaphore out"=w262:T3)  [unwired: 4 in, 1 out]
                n76 = VISA Write(VISA resource name=w260, write buffer="#!@XDC\r", error in (no error)=w259) -> (error out=w258:errorcluster)  [unwired: 2 out]
                n77 = call <vilib>:"Release Semaphore.vi"("error in (no error)"=w258, "semaphore"=w262) -> ()  [unwired: 4 in, 2 out]
              }
            }
          }
          event "StartPump": Value Change {
            n78 = event-data() -> ("NewVal"=w269:bool)  [unwired: 1 in, 5 out]
            n79 = case shown="True" w269 {
              tunnel: w268 -> [_ w274]
              tunnel: w267 -> [_ w273]
              frame False {
              }
              frame True {
                n80 = Unbundle By Name(w273) -> ("ConfiguredPumpCom"=w272:refnum<visa-resource-name>)
                n81 = Unbundle By Name(w274) -> ("laser semaphore"=w271:T3)
                n82 = call <vilib>:"Acquire Semaphore.vi"("semaphore"=w271) -> ("error out"=w276:errorcluster, "semaphore out"=w270:T3)  [unwired: 4 in, 1 out]
                n83 = call "pumpStart.vi"("error in (no error)"=w276, "VISA resource name"=w272) -> ("error out"=w275:errorcluster)  [unwired: 9 in]
                n84 = call <vilib>:"Release Semaphore.vi"("error in (no error)"=w275, "semaphore"=w270) -> ()  [unwired: 4 in, 2 out]
              }
            }
          }
          event "SopPump": Value Change {
            n85 = event-data() -> ("NewVal"=w280:bool)  [unwired: 1 in, 5 out]
            n86 = case shown="True" w280 {
              tunnel: w279 -> [_ w284]
              tunnel: w278 -> [_ w282]
              frame False {
              }
              frame True {
                n87 = Unbundle By Name(w284) -> ("pump semaphore"=w283:T3)
                n88 = Unbundle By Name(w282) -> ("ConfiguredPumpCom"=w281:refnum<visa-resource-name>)
                n89 = call <vilib>:"Acquire Semaphore.vi"("semaphore"=w283) -> ("error out"=w287:errorcluster, "semaphore out"=w285:T3)  [unwired: 4 in, 1 out]
                n90 = call "pumpStop.vi"("error in (no error)"=w287, "VISA resource name"=w281) -> ("error out"=w286:errorcluster)  [unwired: 9 in]
                n91 = call <vilib>:"Release Semaphore.vi"("error in (no error)"=w286, "semaphore"=w285) -> ()  [unwired: 4 in, 2 out]
              }
            }
          }
          event "HVEnable": Value Change {
            n92 = event-data() -> ("NewVal"=w289:bool)  [unwired: 1 in, 5 out]
            n93 = case shown="True" w289 {
              frame False {
                n94 = call "setDO.vi"("channel"=2, "on/off"=TRUE) -> ("错误输出"=w292:errorcluster)  [unwired: 9 in]
                n95 = call "setDO.vi"("错误输入（无错误）"=w292, "channel"=3, "on/off"=TRUE) -> ("错误输出"=w291:errorcluster)  [unwired: 8 in]
                n96 = call "setDO.vi"("错误输入（无错误）"=w291, "channel"=4, "on/off"=TRUE) -> ("错误输出"=w290:errorcluster)  [unwired: 8 in]
                n97 = call "setDO.vi"("错误输入（无错误）"=w290, "channel"=5, "on/off"=TRUE) -> ()  [unwired: 8 in, 1 out]
              }
              frame True {
                n98 = property on="MCPHV-Set" class="DigNum (strict)"() -> ("Value"=w325:dbl)  [unwired: 2 in, 2 out]
                n99 = Divide(x=w325, y=2000.0) -> (x/y=w327:dbl)
                n100 = Multiply(x=w327, y=10.0) -> (x*y=w318:dbl)
                n101 = Less?(x=w318, y=1.0) -> (x < y?=w319:bool)
                n102 = call "setDO.vi"("channel"=2, "on/off"=FALSE) -> ("错误输出"=w331:errorcluster)  [unwired: 9 in]
                n103 = case shown="False" w319 {
                  tunnel: w318 -> [w386 w394]
                  frame False {
                    n104 = while {
                      tunnel: w386 -> [w388]
                      tunnel: [w388] -> w384
                      i -> [w392]
                      stop <- w389 stop-if-true
                      n105 = Increment(x=w392) -> (x+1=w391:i32)
                      n106 = Increment(x=w391) -> (x+1=w390:i32)
                      n107 = call "setAO.vi"("value"=w391, "channel"=0) -> ()  [unwired: 9 in, 1 out]
                      n108 = Greater Or Equal?(x=w390, y=w388) -> (x >= y?=w389:bool)
                      n109 = Wait (ms)(milliseconds to wait=1000) -> ()  [unwired: 1 out]
                    }
                    n110 = call "setAO.vi"("value"=w384, "channel"=0) -> ()  [unwired: 9 in, 1 out]
                  }
                  frame True {
                    n111 = call "setAO.vi"("value"=w394, "channel"=0) -> ()  [unwired: 9 in, 1 out]
                  }
                }
                n112 = call "setDO.vi"("错误输入（无错误）"=w331, "channel"=3, "on/off"=FALSE) -> ("错误输出"=w330:errorcluster)  [unwired: 8 in]
                n113 = call "setDO.vi"("错误输入（无错误）"=w330, "channel"=4, "on/off"=FALSE) -> ("错误输出"=w329:errorcluster)  [unwired: 8 in]
                n114 = property on="Tar.HV-Set" class="DigNum (strict)"() -> ("Value"=w321:dbl)  [unwired: 2 in, 2 out]
                n115 = Divide(x=w321, y=20000.0) -> (x/y=w323:dbl)
                n116 = call "setDO.vi"("错误输入（无错误）"=w329, "channel"=5, "on/off"=FALSE) -> ()  [unwired: 8 in, 1 out]
                n117 = Multiply(x=w323, y=10.0) -> (x*y=w315:dbl)
                n118 = Less?(x=w315, y=0.5) -> (x < y?=w316:bool)
                n119 = case shown="False" w316 {
                  tunnel: w315 -> [w370 w382]
                  frame False {
                    n120 = while {
                      tunnel: w370 -> [w379]
                      tunnel: [w379] -> w368
                      i -> [w375]
                      stop <- w380 stop-if-true
                      n121 = Divide(x=w375, y=2.0) -> (x/y=w376:dbl)
                      n122 = Add(x=0.5, y=w376) -> (x+y=w373:dbl)
                      n123 = Add(x=w373, y=0.5) -> (x+y=w371:dbl)
                      n124 = call "setAO.vi"("value"=w373, "channel"=1) -> ()  [unwired: 9 in, 1 out]
                      n125 = Greater Or Equal?(x=w371, y=w379) -> (x >= y?=w380:bool)
                      n126 = Wait (ms)(milliseconds to wait=500) -> ()  [unwired: 1 out]
                    }
                    n127 = call "setAO.vi"("value"=w368, "channel"=1) -> ()  [unwired: 9 in, 1 out]
                  }
                  frame True {
                    n128 = call "setAO.vi"("value"=w382, "channel"=1) -> ()  [unwired: 9 in, 1 out]
                  }
                }
                n129 = property on="Pul.HV-Set" class="DigNum (strict)"() -> ("Value"=w314:dbl)  [unwired: 2 in, 2 out]
                n130 = Divide(x=w314, y=2000.0) -> (x/y=w309:dbl)
                n131 = Multiply(x=w309, y=10.0) -> (x*y=w313:dbl)
                n132 = Less?(x=w313, y=1.0) -> (x < y?=w312:bool)
                n133 = case shown="False" w312 {
                  tunnel: w313 -> [w358 w366]
                  frame False {
                    n134 = while {
                      tunnel: w358 -> [w360]
                      tunnel: [w360] -> w356
                      i -> [w364]
                      stop <- w361 stop-if-true
                      n135 = Increment(x=w364) -> (x+1=w363:i32)
                      n136 = Increment(x=w363) -> (x+1=w362:i32)
                      n137 = call "setAO.vi"("value"=w363, "channel"=2) -> ()  [unwired: 9 in, 1 out]
                      n138 = Greater Or Equal?(x=w362, y=w360) -> (x >= y?=w361:bool)
                      n139 = Wait (ms)(milliseconds to wait=1000) -> ()  [unwired: 1 out]
                    }
                    n140 = call "setAO.vi"("value"=w356, "channel"=2) -> ()  [unwired: 9 in, 1 out]
                  }
                  frame True {
                    n141 = call "setAO.vi"("value"=w366, "channel"=2) -> ()  [unwired: 9 in, 1 out]
                  }
                }
                n142 = property on="LensHV-Set" class="DigNum (strict)"() -> ("Value"=w307:dbl)  [unwired: 2 in, 2 out]
                n143 = Divide(x=w307, y=10000.0) -> (x/y=w302:dbl)
                n144 = Multiply(x=w302, y=10.0) -> (x*y=w306:dbl)
                n145 = Less?(x=w306, y=0.5) -> (x < y?=w305:bool)
                n146 = case shown="False" w305 {
                  tunnel: w306 -> [w342 w354]
                  frame False {
                    n147 = while {
                      tunnel: w342 -> [w351]
                      tunnel: [w351] -> w340
                      i -> [w347]
                      stop <- w352 stop-if-true
                      n148 = Divide(x=w347, y=2.0) -> (x/y=w348:dbl)
                      n149 = Add(x=0.5, y=w348) -> (x+y=w345:dbl)
                      n150 = Add(x=w345, y=0.5) -> (x+y=w343:dbl)
                      n151 = call "setAO.vi"("value"=w345, "channel"=3) -> ()  [unwired: 9 in, 1 out]
                      n152 = Greater Or Equal?(x=w343, y=w351) -> (x >= y?=w352:bool)
                      n153 = Wait (ms)(milliseconds to wait=500) -> ()  [unwired: 1 out]
                    }
                    n154 = call "setAO.vi"("value"=w340, "channel"=3) -> ()  [unwired: 9 in, 1 out]
                  }
                  frame True {
                    n155 = call "setAO.vi"("value"=w354, "channel"=3) -> ()  [unwired: 9 in, 1 out]
                  }
                }
              }
            }
          }
          event "Samp_Atmos": Value Change {
            n156 = event-data() -> ("OldVal"=w397:bool, "NewVal"=w401:bool)  [unwired: 1 in, 4 out]
            n157 = property on="Fore_Samp" class="Bool (strict)"() -> ("Value"=w400:bool)  [unwired: 2 in, 2 out]
            n158 = And(x=w401, y=w400) -> (x .and. y?=w399:bool)
            n159 = Not(x=w399) -> (.not. x?=w398:bool)
            n160 = case shown="True" w398 {
              tunnel: w401 -> [_ w404]
              tunnel: w397 -> [w403 _]
              frame False {
                n161 = property on="Samp_Atmos" class="Bool (strict)"("Value"=w403) -> (error out=w402:errorcluster)  [unwired: 2 in, 1 out]
                n162 = call "Display Message to User7"("error in (no error)"=w402) -> ()  [unwired: 9 in, 2 out]
              }
              frame True {
                n163 = case shown="False" w404 {
                  frame False {
                    n164 = call "setDO.vi"("channel"=6, "on/off"=FALSE) -> ()  [unwired: 9 in, 1 out]
                  }
                  frame True {
                    n165 = property on="Y满" class="Bool (strict)"() -> ("Value"=w408:bool)  [unwired: 2 in, 2 out]
                    n166 = Not(x=w408) -> (.not. x?=w407:bool)
                    n167 = case shown="False" w407 {
                      frame False {
                        n168 = call "setDO.vi"("channel"=6, "on/off"=TRUE) -> ()  [unwired: 9 in, 1 out]
                      }
                      frame True {
                        n169 = call "Display Message to User6"() -> ()  [unwired: 10 in, 2 out]
                      }
                    }
                  }
                }
              }
            }
          }
          event "Fore_Samp": Value Change {
            n170 = event-data() -> ("OldVal"=w412:bool, "NewVal"=w416:bool)  [unwired: 1 in, 4 out]
            n171 = property on="Samp_Atmos" class="Bool (strict)"() -> ("Value"=w415:bool)  [unwired: 2 in, 2 out]
            n172 = And(x=w416, y=w415) -> (x .and. y?=w414:bool)
            n173 = Not(x=w414) -> (.not. x?=w413:bool)
            n174 = case shown="True" w413 {
              tunnel: w416 -> [_ w419]
              tunnel: w412 -> [w418 _]
              frame False {
                n175 = property on="Fore_Samp" class="Bool (strict)"("Value"=w418) -> (error out=w417:errorcluster)  [unwired: 2 in, 1 out]
                n176 = call "Display Message to User8"("error in (no error)"=w417) -> ()  [unwired: 9 in, 2 out]
              }
              frame True {
                n177 = case shown="True" w419 {
                  frame False {
                    n178 = call "setDO.vi"("channel"=7, "on/off"=FALSE) -> ()  [unwired: 9 in, 1 out]
                  }
                  frame True {
                    n179 = property on="Y满" class="Bool (strict)"() -> ("Value"=w423:bool)  [unwired: 2 in, 2 out]
                    n180 = Not(x=w423) -> (.not. x?=w422:bool)
                    n181 = case shown="True" w422 {
                      frame False {
                        n182 = call "setDO.vi"("channel"=7, "on/off"=TRUE) -> ()  [unwired: 9 in, 1 out]
                      }
                      frame True {
                        n183 = call "Display Message to User"() -> ()  [unwired: 10 in, 2 out]
                      }
                    }
                  }
                }
              }
            }
          }
          event "MCPHV-Set": Value Change {
            n184 = event-data() -> ("NewVal"=w427:dbl)  [unwired: 1 in, 5 out]
            n185 = Divide(x=w427, y=2000.0) -> (x/y=w430:dbl)
            n186 = Multiply(x=w430, y=10.0) -> (x*y=w428:dbl)
            n187 = call "setAO.vi"("value"=w428, "channel"=0) -> ()  [unwired: 9 in, 1 out]
          }
          event "Tar.HV-Set": Value Change {
            n188 = event-data() -> ("NewVal"=w439:dbl)  [unwired: 1 in, 5 out]
            n189 = Divide(x=w439, y=20000.0) -> (x/y=w436:dbl)
            n190 = Multiply(x=w436, y=10.0) -> (x*y=w434:dbl)
            n191 = call "setAO.vi"("value"=w434, "channel"=1) -> ()  [unwired: 9 in, 1 out]
          }
          event "Pul.HV-Set": Value Change {
            n192 = event-data() -> ("NewVal"=w446:dbl)  [unwired: 1 in, 5 out]
            n193 = Divide(x=w446, y=2000.0) -> (x/y=w443:dbl)
            n194 = Multiply(x=w443, y=10.0) -> (x*y=w441:dbl)
            n195 = call "setAO.vi"("value"=w441, "channel"=2) -> ()  [unwired: 9 in, 1 out]
          }
          event "LensHV-Set": Value Change {
            n196 = event-data() -> ("NewVal"=w453:dbl)  [unwired: 1 in, 5 out]
            n197 = Divide(x=w453, y=10000.0) -> (x/y=w450:dbl)
            n198 = Multiply(x=w450, y=10.0) -> (x*y=w449:dbl)
            n199 = call "setAO.vi"("value"=w449, "channel"=3) -> ()  [unwired: 9 in, 1 out]
          }
          event "Image": Mouse Down {
            n200 = event-data() -> ("Coords"=w454:T16)  [unwired: 1 in, 7 out]
            n201 = property on="移动" class="Bool (strict)"() -> ("Value"=w455:bool)  [unwired: 2 in, 2 out]
            n202 = case shown="False" w455 {
              tunnel: w454 -> [w466 _]
              frame False {
                w463 = -0.005 ("x")
                n203 = Unbundle(w466) -> ("Horizontal"=w465:i32, "Vertical"=w464:i32)
                n204 = property on="X当前" class="DigNum (strict)"() -> ("Value"=w462:dbl)  [unwired: 2 in, 2 out]
                n205 = property on="Y当前" class="DigNum (strict)"() -> ("Value"=w458:dbl)  [unwired: 2 in, 2 out]
                n206 = Subtract(x=w465, y=252.0) -> (x-y=w468:dbl)
                n207 = Subtract(x=w464, y=191.0) -> (x-y=w467:dbl)
                n208 = Multiply(x=w463, y=w468) -> (x*y=w461:dbl)
                n209 = Multiply(x=w463, y=w467) -> (x*y=w459:dbl)
                n210 = Add(x=w462, y=w461) -> (x+y=w460:dbl)
                n211 = Add(x=w459, y=w458) -> (x+y=w457:dbl)
                n212 = call "goto.vi"("Y(mm)"=w457, "X(mm)"=w460) -> ()  [unwired: 9 in, 1 out]
              }
              frame True {
              }
            }
          }
          event "TakeMS-Run": Value Change {
            n213 = event-data() -> ("NewVal"=w476:bool)  [unwired: 1 in, 5 out]
            n214 = case shown="True" w476 {
              tunnel: w475 -> [_ w492]
              tunnel: w474 -> [_ w489]
              tunnel: w473 -> [_ w488]
              tunnel: w472 -> [w477 w479]
              tunnel: [w477 w478] -> w471
              frame False {
              }
              frame True {
                n215 = Unbundle By Name(w488) -> ("ConfiguredLaserCom"=w485:refnum<visa-resource-name>)
                n216 = Unbundle By Name(w489) -> ("laser semaphore"=w483:T3)
                n217 = property on="cluster" class="Clust (strict)"() -> ("Value"=w487:T7)  [unwired: 2 in, 2 out]
                n218 = Bundle By Name(cluster=w492, "ShotsPerPoint"="Shots/Point") -> (w490:T5)
                n219 = Unbundle By Name(w487) -> ("待机"=w484:bool)
                n220 = property on="SetLaserEnergy" class="Slide (strict)"() -> ("Value"=w482:dbl)  [unwired: 2 in, 2 out]
                n221 = Bundle By Name(cluster="Laser parameter", "VISA resource name"=w485, "standby"=w484, "semaphore in"=w483, "SetLaserEnergy"=w482) -> (w481:T4)
                n222 = case shown="0, Default" "AcquireMS-Methods" {
                  tunnel: w490 -> [w512 _ _]
                  tunnel: w481 -> [w513 _ _]
                  tunnel: w479 -> [w511 w522 w523]
                  tunnel: [w502 w522 w523] -> w478
                  frame 0, Default {
                    n223 = Get Date/Time String() -> (date string=w509:string, time string=w508:string)  [unwired: 3 in]
                    n224 = Concatenate Strings(w509, " " ("字符串"), w508) -> (w503:string)
                    n225 = call "Tiepie-takeData-2018-06-01.vi"("left rank"="left rank", "right rank"="right rank", "deBaseline"="deBaseline", "Thresh"="Thresh", "Laser parameter"=w513, "ADC parameter"=w512) -> ("output cluster"=w494:cluster{dbl[], "filtered data":dbl[]})  [unwired: 1 in, 1 out]
                    "MS" <- w494
                    n226 = Unbundle(w494) -> (w495:dbl[], "filtered data"=w510:dbl[])
                    n227 = property on="currentNO" class="Str"() -> ("Value"=w505:string)  [unwired: 2 in, 2 out]
                    n228 = Bundle By Name(cluster=T11 {"tag1"="", "tag2"="", "x"=[], "y"=[], "ID1:X"=[], "ID1:Y"=[], "ID1:REF:X"=[], "ID1:REF:Y"=[], "ID2:X"=[], "ID2:Y"=[], "ID2:REF:X"=[], "ID2:REF:Y"=[], "ID3:X"=[], "ID3:Y"=[], "ID3:REF:X"=[], "ID3:REF:Y"=[], "ID1:TAG1"="", "ID1:TAG2"="", "ID2:TAG1"="", "ID2:TAG2"="", "ID3:TAG1"="", "ID3:TAG2"="", "ID1:NAME"="", "ID2:NAME"="", "ID3:NAME"="", "ID1:SCORE"="", "ID2:SCORE"="", "ID3:SCORE"="", "NO"=""}, "y"=w510, "x"=w495, "tag1"="未鉴定", "tag2"=w503, "NO"=w505) -> (w504:T11)
                    n229 = Build Array (concatenate)(w511, w504) -> (w502:T8)
                    n230 = for {
                      tunnel: w502 -> [w521] mode=indexing
                      shift-right: [w514] -> w500
                      shift-left: string[][] [] ("Item Names") -> [w516]
                      i -> [w517]
                      n231 = Unbundle By Name(w521) -> ("NO"=w520:string, "tag1"=w519:string, "tag2"=w518:string)
                      n232 = Build Array(w520, w519, w518) -> (w515:string[])
                      n233 = Insert Into Array "Insert Into Array"(array=w516, index (row)=w517, new element=w515) -> (w514:string[][])  [unwired: 1 in]
                    }
                    n234 = property on="测试记录" class="MCListbox (strict)"("ItemNames"=w500) -> ()  [unwired: 2 in, 2 out]
                  }
                  frame 1 {
                  }
                  frame 2 {
                  }
                }
              }
            }
          }
          event "Set Laser": Value Change {
            n235 = event-data() -> ("NewVal"=w526:bool)  [unwired: 1 in, 5 out]
            n236 = case shown="True" w526 {
              tunnel: w525 -> [_ w534]
              tunnel: w524 -> [_ w529]
              frame False {
              }
              frame True {
                n237 = Unbundle By Name(w529) -> ("ConfiguredLaserCom"=w528:refnum<visa-resource-name>)
                n238 = Unbundle By Name(w534) -> ("laser semaphore"=w533:T3)
                n239 = call <vilib>:"Acquire Semaphore.vi"("semaphore"=w533) -> ("error out"=w532:errorcluster, "semaphore out"=w530:T3)  [unwired: 4 in, 1 out]
                n240 = call "Laser-Set-Parmeter.vi"("error in (no error)"=w532, "LaserHV"="LaserHV", "LaserFreq"="频率/Hz", "SetLaserEnergy"="SetLaserEnergy", "VISA resource name"=w528) -> ("error out"=w531:errorcluster)  [unwired: 1 in, 1 out]
                n241 = call <vilib>:"Release Semaphore.vi"("error in (no error)"=w531, "semaphore"=w530) -> ()  [unwired: 4 in, 2 out]
              }
            }
          }
          event "测试记录": Shortcut Menu Selection (User) {
            n242 = event-data() -> ("ItemTag"=w540:string)  [unwired: 1 in, 7 out]
            n243 = case shown="\"鉴定\"" w540 {
              tunnel: w539 -> [w541 w548 w555 w560]
              tunnel: [w541 w548 w555 w556] -> w538
              frame "假", Default {
              }
              frame "鉴定" {
                n244 = property on="selected row" class="DigNum (strict)"() -> ("Value"=w544:i32)  [unwired: 2 in, 2 out]
                n245 = Index Array(array=w548, index=w544) -> (element=w554:T11)
                n246 = Unbundle By Name(w554) -> ("x"=w553:dbl[], "y"=w549:dbl[])
                n247 = call-poly <userlib>:"CaLabPut.vi"("Values"=w553, "PV Names"="MS:X") -> ("Error out"=w551:errorcluster)  [unwired: 6 in, 3 out]
                n248 = call-poly <userlib>:"CaLabPut.vi"("Error in (no error)"=w551, "Values"=w549, "PV Names"="MS:Y") -> ("Error out"=w547:errorcluster)  [unwired: 5 in, 3 out]
                n249 = call-poly <userlib>:"CaLabPut.vi"("Error in (no error)"=w547, "Value"=w544, "PV Name"="MS:NUM") -> ("Error out"=w546:errorcluster)  [unwired: 5 in, 3 out]
                n250 = call-poly <userlib>:"CaLabPut.vi"("Error in (no error)"=w546, "Value"=1, "PV Name"="MS:START") -> ()  [unwired: 5 in, 4 out]
              }
              frame "参数" {
              }
              frame "删除" {
                n251 = property on="selected row" class="DigNum (strict)"() -> ("Value"=w559:i32)  [unwired: 2 in, 2 out]
                n252 = Delete From Array "Delete From Array"(array=w560, index=w559) -> (array with subset deleted=w556:T8)  [unwired: 1 in, 1 out]
                n253 = for {
                  tunnel: w556 -> [w568] mode=indexing
                  shift-right: [w561] -> w557
                  shift-left: string[][] [] ("Item Names") -> [w563]
                  i -> [w564]
                  n254 = Unbundle By Name(w568) -> ("NO"=w567:string, "tag1"=w566:string, "tag2"=w565:string)
                  n255 = Build Array(w567, w566, w565) -> (w562:string[])
                  n256 = Insert Into Array "Insert Into Array"(array=w563, index (row)=w564, new element=w562) -> (w561:string[][])  [unwired: 1 in]
                }
                n257 = property on="测试记录" class="MCListbox (strict)"("ItemNames"=w557) -> ()  [unwired: 2 in, 2 out]
              }
            }
          }
          event "测试记录": Mouse Down {
            n258 = event-data() -> ("Coords"=w574:T16)  [unwired: 1 in, 7 out]
            n259 = invoke on="测试记录" class="MCListbox (严格)" method="Point To Row Column"("Point"=w574) -> ("CellPosition"=w573:T17)  [unwired: 6 in, 6 out]
            n260 = Unbundle By Name(w573) -> ("Row"=w570:i32)
            n261 = Array Size(array=w569) -> (size(s)=w572:i32)
            n262 = Greater Or Equal?(x=w572, y=w570) -> (x >= y?=w571:bool)
            n263 = case shown="True" w571 {
              tunnel: w570 -> [_ w601]
              tunnel: w569 -> [_ w602]
              frame False {
              }
              frame True {
                n264 = property on="selected row" class="DigNum (strict)"("Value"=w601) -> ()  [unwired: 2 in, 2 out]
                n265 = Index Array(array=w602, index=w601) -> (element=w600:T11)
                n266 = Unbundle By Name(w600) -> ("ID1:TAG1"=w583:string, "ID1:TAG2"=w597:string, "ID1:NAME"=w596:string, "ID1:SCORE"=w587:string, "ID2:TAG1"=w581:string, "ID2:TAG2"=w594:string, "ID2:NAME"=w593:string, "ID2:SCORE"=w586:string, "ID3:TAG1"=w579:string, "ID3:TAG2"=w578:string, "ID3:NAME"=w577:string, "ID3:SCORE"=w576:string)
                n267 = Build Array("1" ("element"), w583, w597, w596, w587) -> (w595:string[])
                n268 = Build Array("2" ("element"), w581, w594, w593, w586) -> (w590:string[])
                n269 = Build Array("3" ("element"), w579, w578, w577, w576) -> (w585:string[])
                n270 = Insert Into Array(array=string[][] [] ("项名"), index (row)=0 ("索引 (行)"), new element=w595) -> (w592:string[][])  [unwired: 1 in]
                n271 = Insert Into Array(array=w592, index (row)=1 ("索引 (行)"), new element=w590) -> (w589:string[][])  [unwired: 1 in]
                n272 = Insert Into Array(array=w589, index (row)=2 ("索引 (行)"), new element=w585) -> (w584:string[][])  [unwired: 1 in]
                n273 = property on="Identification Results (单靶鉴定结果)" class="MCListbox (strict)"("ItemNames"=w584) -> ()  [unwired: 2 in, 2 out]
              }
            }
          }
          event "Identification Results (单靶鉴定结果)": Mouse Down {
            n274 = event-data() -> ("Coords"=w608:T16)  [unwired: 1 in, 7 out]
            n275 = invoke on="Identification Results (单靶鉴定结果)" class="MCListbox (严格)" method="Point To Row Column"("Point"=w608) -> ("CellPosition"=w607:T17)  [unwired: 6 in, 6 out]
            n276 = Unbundle By Name(w607) -> ("Row"=w603:i32)
            n277 = Less Or Equal?(x=w603, y=2) -> (x <= y?=w605:bool)
            n278 = case shown="True" w605 {
              tunnel: w604 -> [_ w615]
              tunnel: w603 -> [_ w609]
              frame False {
              }
              frame True {
                n279 = property on="selected row" class="DigNum (strict)"() -> ("Value"=w614:i32)  [unwired: 2 in, 2 out]
                n280 = Index Array(array=w615, index=w614) -> (element=w613:T11)
                n281 = case shown="2" w609 {
                  tunnel: w613 -> [w621 w633 w642]
                  tunnel: [w620 w629 w638] -> w612
                  tunnel: [w619 w628 w637] -> w610
                  frame 0, Default {
                    n282 = Unbundle By Name(w621) -> ("x"=w623:dbl[], "y"=w622:dbl[], "ID1:REF:X"=w624:dbl[], "ID1:REF:Y"=w618:dbl[])
                    n283 = Multiply(x=w618, y=-1.0) -> (x*y=w616:dbl[])
                    n284 = Bundle("x"=w623, "y"=w622) -> (w620:cluster{"x":dbl[], "y":dbl[]})  [unwired: 1 in]
                    n285 = Bundle("ID1:REF:X"=w624, w616) -> (w619:cluster{"ID1:REF:X":dbl[], dbl[]})  [unwired: 1 in]
                  }
                  frame 1 {
                    n286 = Unbundle By Name(w633) -> ("x"=w631:dbl[], "y"=w630:dbl[], "ID2:REF:X"=w632:dbl[], "ID2:REF:Y"=w627:dbl[])
                    n287 = Multiply(x=w627, y=-1.0) -> (x*y=w625:dbl[])
                    n288 = Bundle("x"=w631, "y"=w630) -> (w629:cluster{"x":dbl[], "y":dbl[]})  [unwired: 1 in]
                    n289 = Bundle("ID2:REF:X"=w632, w625) -> (w628:cluster{"ID2:REF:X":dbl[], dbl[]})  [unwired: 1 in]
                  }
                  frame 2 {
                    n290 = Unbundle By Name(w642) -> ("x"=w640:dbl[], "y"=w639:dbl[], "ID3:REF:X"=w641:dbl[], "ID3:REF:Y"=w636:dbl[])
                    n291 = Multiply(x=w636, y=-1.0) -> (x*y=w634:dbl[])
                    n292 = Bundle("x"=w640, "y"=w639) -> (w638:cluster{"x":dbl[], "y":dbl[]})  [unwired: 1 in]
                    n293 = Bundle("ID3:REF:X"=w641, w634) -> (w637:cluster{"ID3:REF:X":dbl[], dbl[]})  [unwired: 1 in]
                  }
                }
                n294 = Build Array(w612, w610) -> (→"Identify Spcetrum":cluster{"ID3:REF:X":dbl[], "y":dbl[]}[])
              }
            }
          }
          event "Plat_To_Zero": Value Change {
            n295 = event-data() -> ("NewVal"=w644:bool)  [unwired: 1 in, 5 out]
            n296 = case shown="False" w644 {
              frame False {
              }
              frame True {
                (unwired) TRUE ("plat zeroed")
                n297 = call "plate_cal.vi"() -> ()  [unwired: 11 in, 1 out]
              }
            }
          }
          event "GO": Value Change {
            n298 = event-data() -> ("NewVal"=w647:bool)  [unwired: 1 in, 5 out]
            n299 = property on="移动" class="Bool (strict)"() -> ("Value"=w649:bool)  [unwired: 2 in, 2 out]
            n300 = Not(x=w649) -> (.not. x?=w648:bool)
            n301 = And(x=w648, y=w647) -> (x .and. y?=w646:bool)
            n302 = case shown="True" w646 {
              frame False {
              }
              frame True {
                n303 = property on="X" class="DigNum (strict)"() -> ("Value"=w651:dbl)  [unwired: 2 in, 2 out]
                n304 = property on="Y" class="DigNum (strict)"() -> ("Value"=w650:dbl)  [unwired: 2 in, 2 out]
                n305 = call "goto.vi"("Y(mm)"=w650, "X(mm)"=w651) -> ()  [unwired: 9 in, 1 out]
              }
            }
          }
          event "chamber in": Value Change {
            n306 = event-data() -> ("NewVal"=w654:bool)  [unwired: 1 in, 5 out]
            n307 = property on="HVEnable" class="Bool (strict)"() -> ("Value"=w659:bool)  [unwired: 2 in, 2 out]
            n308 = property on="Y满" class="Bool (strict)"() -> ("Value"=w655:bool)  [unwired: 2 in, 2 out]
            n309 = property on="移动" class="Bool (strict)"() -> ("Value"=w658:bool)  [unwired: 2 in, 2 out]
            n310 = Not(x=w659) -> (.not. x?=w656:bool)
            n311 = Not(x=w658) -> (.not. x?=w657:bool)
            n312 = Compound Arithmetic op=AND(w656, w655, w657, w654) -> (w653:bool)
            n313 = case shown="True" w653 {
              frame False {
              }
              frame True {
                n314 = flat-sequence {
                  tunnel: [w664] -> w660
                  tunnel: w660 -> [w674]
                  frame #0 {
                    n315 = call "样品标识与备注"() -> ("备注"=w661:string, "样品名称"=w662:string)  [unwired: 16 in, 2 out]
                    n316 = property on="sampleID" class="Str"("Value"=w662) -> ()  [unwired: 2 in, 2 out]
                    n317 = property on="commet" class="Str"("Value"=w661) -> ()  [unwired: 2 in, 2 out]
                  }
                  frame #1 {
                    w665 = FALSE ("on/off")
                    # "关样仓/大气"
                    n318 = Wait (ms)(milliseconds to wait=1500) -> ()  [unwired: 1 out]
                    n319 = call "setDO.vi"("channel"=6, "on/off"=w665) -> ("错误输出"=w663:errorcluster)  [unwired: 9 in]
                    n320 = property on="Samp_Atmos" class="Bool (strict)"(error in=w663, "Value"=w665) -> (error out=w664:errorcluster)  [unwired: 1 in, 1 out]
                  }
                  frame #2 {
                    # "开前泵/样仓"
                    n321 = call "setDO.vi"("错误输入（无错误）"=w674, "channel"=7, "on/off"=TRUE) -> ("错误输出"=w673:errorcluster)  [unwired: 8 in]
                    n322 = flat-sequence {
                      tunnel: w673 -> [w684]
                      tunnel: [w684] -> w669
                      frame #0 {
                        n323 = Wait (ms)(milliseconds to wait=10000) -> ()  [unwired: 1 out]
                      }
                    }
                    n324 = property on="Lvaccum" class="DigNum (strict)"(error in=w669) -> (error out=w668:errorcluster, "Value"=w672:dbl)  [unwired: 1 in, 1 out]
                    n325 = Less?(x=w672, y=10) -> (x < y?=w670:bool)
                    n326 = case shown="False" w670 {
                      tunnel: w668 -> [w678 w680]
                      frame False {
                        (unwired) 7
                        n327 = call "setDO.vi"("错误输入（无错误）"=w678, "on/off"=FALSE) -> ("错误输出"=w677:errorcluster)  [unwired: 9 in]
                        n328 = call "Display Message to User4"("error in (no error)"=w677) -> ()  [unwired: 9 in, 2 out]
                      }
                      frame True {
                        n329 = flat-sequence {
                          tunnel: w680 -> [w681]
                          frame #0 {
                            n330 = call "setDO.vi"("错误输入（无错误）"=w681, "channel"=7, "on/off"=FALSE) -> ()  [unwired: 8 in, 1 out]
                          }
                          frame #1 {
                            n331 = call "chamber_in.vi"() -> ()  [unwired: 12 in]
                          }
                        }
                      }
                    }
                  }
                }
              }
            }
          }
          event "chamber out": Value Change {
            n332 = event-data() -> ("NewVal"=w686:bool)  [unwired: 1 in, 5 out]
            n333 = case shown="True" w686 {
              frame False {
              }
              frame True {
                n334 = property on="移动" class="Bool (strict)"() -> ("Value"=w692:bool)  [unwired: 2 in, 2 out]
                n335 = property on="Y满" class="Bool (strict)"() -> ("Value"=w693:bool)  [unwired: 2 in, 2 out]
                n336 = property on="HVEnable" class="Bool (strict)"() -> ("Value"=w694:bool)  [unwired: 2 in, 2 out]
                n337 = Not "非"(x=w692) -> (.not. x?=w690:bool)
                n338 = Not "非"(x=w693) -> (.not. x?=w691:bool)
                n339 = Not "非"(x=w694) -> (.not. x?=w688:bool)
                n340 = Compound Arithmetic op=AND "复合运算"(w688, w691, w690) -> (w689:bool)
                n341 = case shown="True" w689 {
                  frame False {
                    n342 = call "Display Message to User3"() -> ()  [unwired: 10 in, 2 out]
                  }
                  frame True {
                    n343 = flat-sequence {
                      tunnel: [w698] -> w696
                      tunnel: w696 -> [w704]
                      tunnel: [w705] -> w695
                      tunnel: w695 -> [w716]
                      frame #0 {
                        n344 = call "chamber_out.vi"() -> ()  [unwired: 12 in]
                      }
                      frame #1 {
                        w699 = FALSE ("on/off")
                        # "关前泵/样仓"
                        n345 = Wait (ms)(milliseconds to wait=1500) -> ()  [unwired: 1 out]
                        n346 = call "setDO.vi"("channel"=7, "on/off"=w699) -> ("错误输出"=w697:errorcluster)  [unwired: 9 in]
                        n347 = property on="Fore_Samp" class="Bool (strict)"(error in=w697, "Value"=w699) -> (error out=w698:errorcluster)  [unwired: 1 in, 1 out]
                      }
                      frame #2 {
                        # "开样仓/大气"
                        n348 = call "Time Delay4"("error in (no error)"=w704, "Delay Time (s)"=3.0) -> ("error out"=w703:errorcluster)  [unwired: 9 in]
                        n349 = property on="Y满" class="Bool (strict)"(error in=w703) -> (error out=w706:errorcluster, "Value"=w707:bool)  [unwired: 1 in, 1 out]
                        n350 = case shown="True" w707 {
                          tunnel: w706 -> [w709 w711]
                          tunnel: [w708 w710] -> w705
                          frame False {
                            n351 = call "Display Message to User2"("error in (no error)"=w709) -> ("error out"=w708:errorcluster)  [unwired: 9 in, 1 out]
                          }
                          frame True {
                            n352 = call "setDO.vi"("错误输入（无错误）"=w711, "channel"=6, "on/off"=TRUE) -> ("错误输出"=w710:errorcluster)  [unwired: 8 in]
                          }
                        }
                      }
                      frame #3 {
                        n353 = call "Time Delay5"("error in (no error)"=w716, "Delay Time (s)"=3.0) -> ("error out"=w715:errorcluster)  [unwired: 9 in]
                        n354 = call "setDO.vi"("错误输入（无错误）"=w715, "channel"=6, "on/off"=FALSE) -> ()  [unwired: 8 in, 1 out]
                      }
                    }
                  }
                }
              }
            }
          }
          event "标准样品": Value Change {
            n355 = event-data() -> ("NewVal"=w720:u16)  [unwired: 1 in, 5 out]
            n356 = control-ref of="定标参数"() -> (w721:refnum<vi>)
            n357 = local read "std sample"() -> (w719:T1)
            n358 = call "writetable.vi"("std sample"=w719, "type"=w720, "reference"=w721) -> ()  [unwired: 9 in]
          }
          event "peak cal": Value Change {
            n359 = event-data() -> ("NewVal"=w723:bool)  [unwired: 1 in, 5 out]
            n360 = case shown="True" w723 {
              frame False {
              }
              frame True {
                n361 = property on="定标参数" class="MCListbox (strict)"() -> ("ItemNames"=w743:string[][])  [unwired: 2 in, 2 out]
                n362 = Index Array(array=w743, index (col)=1 ("disabled index (col)")) -> (element=w744:string[])  [unwired: 1 in]
                n363 = Index Array(array=w743, index (col)=3 ("disabled index (col)")) -> (element=w741:string[])  [unwired: 1 in]
                n364 = Fract/Exp String To Number(string=w744) -> (number=w733:dbl[])  [unwired: 3 in, 1 out]
                n365 = Fract/Exp String To Number(string=w741) -> (number=w735:dbl[])  [unwired: 3 in, 1 out]
                n366 = call <vilib>:"General Polynomial Fit.vi"("Y"=w733, "polynomial order"=2, "X"=w735) -> ("Polynomial Coefficients"=w737:dbl[])  [unwired: 9 in, 3 out]
                n367 = Index Array(array=w737, index=2) -> (element=w725:dbl)
                "a:" <- w725
                n368 = Index Array(array=w737, index=1) -> (element=w726:dbl)
                "b:" <- w726
                n369 = Index Array(array=w737, index=0) -> (element=w727:dbl)
                "c:" <- w727
                n370 = global write "cal_p.vi" "a"(w725) -> ()
                n371 = global write "cal_p.vi" "b"(w726) -> ()
                n372 = for {
                  tunnel: w735 -> [w758] mode=indexing
                  tunnel: [w762] -> w734 mode=indexing
                  tunnel: w727 -> [w759]
                  tunnel: w726 -> [w760]
                  tunnel: w725 -> [w761]
                  n373 = formula code="m=a*x*x+b*x+c;"("a"=w761, "b"=w760, "c"=w759, "x"=w758) -> ("m"=w762:dbl)
                }
                n374 = global write "cal_p.vi" "c"(w727) -> ()
                n375 = for {
                  tunnel: w734 -> [w756] mode=indexing
                  tunnel: w733 -> [w757] mode=indexing
                  tunnel: [w755] -> w728 mode=indexing
                  n376 = formula code="delta=100*(m-m0)/m0;"("m0"=w757, "m"=w756) -> ("delta"=w755:dbl)
                }
                n377 = control-ref of="定标参数"() -> (w732:refnum<vi>)
                n378 = property on="Property Node" class="MCListbox (strict)"(reference=w732) -> (reference out=w731:refnum<vi>, "ItemNames"=w730:string[][])  [unwired: 1 in, 1 out]
                n379 = for {
                  shift-right: [w751] -> w729
                  shift-left: w730 -> [w754]
                  tunnel: w728 -> [w752] mode=indexing
                  i -> [w753]
                  n380 = Number To Fractional String(number=w752, precision (6)=i16 2) -> (F-format string=w749:string)  [unwired: 2 in]
                  n381 = Concatenate Strings(w749, "%" ("string")) -> (w747:string)
                  n382 = Replace Array Subset(array=w754, new element=w747, index (row)=w753, index (col)=4 ("disabled index (col)")) -> (w751:string[][])
                }
                n383 = property on="Property Node" class="MCListbox (strict)"(reference=w731, "ItemNames"=w729) -> ()  [unwired: 1 in, 2 out]
              }
            }
          }
          event "A1-Position": Value Change {
            n384 = event-data() -> ("NewVal"=w764:bool)  [unwired: 1 in, 5 out]
            n385 = case shown="True" w764 {
              frame False {
              }
              frame True {
                n386 = property on="X当前" class="DigNum (strict)"() -> ("Value"=→"A1-position-X":dbl)  [unwired: 2 in, 2 out]
                n387 = property on="Y当前" class="DigNum (strict)"() -> ("Value"=→"A1-position-Y":dbl)  [unwired: 2 in, 2 out]
              }
            }
          }
          event "A1": Value Change {
            n388 = event-data() -> ("NewVal"=w770:bool)  [unwired: 1 in, 5 out]
            n389 = property on="移动" class="Bool (strict)"() -> ("Value"=w772:bool)  [unwired: 2 in, 2 out]
            n390 = Not(x=w772) -> (.not. x?=w771:bool)
            n391 = And(x=w771, y=w770) -> (x .and. y?=w769:bool)
            n392 = case shown="True" w769 {
              frame False {
              }
              frame True {
                n393 = property on="A1-position-X" class="DigNum (strict)"() -> (error out=w777:errorcluster, "Value"=w775:dbl)  [unwired: 2 in, 1 out]
                n394 = property on="A1-position-Y" class="DigNum (strict)"(error in=w777) -> (error out=w776:errorcluster, "Value"=w774:dbl)  [unwired: 1 in, 1 out]
                n395 = vi-ref "goto.vi"() -> (w781:refnum<vi>)
                n396 = property class="VI"(reference=w781, error in=w776) -> ("Name"=w780:string)  [unwired: 2 out]
                n397 = Open VI Reference(type specifier VI Refnum (for type only)=refnum<vi> refnum, vi path=w780, options=128) -> (vi reference=w778:refnum<vi>)  [unwired: 3 in, 1 out]
                n398 = call-by-ref "Start Asynchronous Call"(reference=w778, "Y(mm)"=w774, "X(mm)"=w775) -> ()  [unwired: 10 in, 3 out]
              }
            }
            n399 = property on="currentNO" class="Str"("Value"="A1") -> ()  [unwired: 2 in, 2 out]
          }
          event "A2": Value Change {
            n400 = event-data() -> ("NewVal"=w785:bool)  [unwired: 1 in, 5 out]
            n401 = property on="移动" class="Bool (strict)"() -> ("Value"=w788:bool)  [unwired: 2 in, 2 out]
            n402 = Not(x=w788) -> (.not. x?=w787:bool)
            n403 = And(x=w787, y=w785) -> (x .and. y?=w786:bool)
            n404 = case shown="True" w786 {
              frame False {
              }
              frame True {
                n405 = property on="A1-position-X" class="DigNum (strict)"() -> (error out=w792:errorcluster, "Value"=w799:dbl)  [unwired: 2 in, 1 out]
                n406 = property on="A1-position-Y" class="DigNum (strict)"(error in=w792) -> (error out=w791:errorcluster, "Value"=w789:dbl)  [unwired: 1 in, 1 out]
                n407 = Subtract(x=w799, y=4.5) -> (x-y=w790:dbl)
                n408 = vi-ref "goto.vi"() -> (w797:refnum<vi>)
                n409 = property class="VI"(reference=w797, error in=w791) -> ("Name"=w796:string)  [unwired: 2 out]
                n410 = Open VI Reference(type specifier VI Refnum (for type only)=refnum<vi> refnum, vi path=w796, options=128) -> (vi reference=w794:refnum<vi>)  [unwired: 3 in, 1 out]
                n411 = call-by-ref "Start Asynchronous Call"(reference=w794, "Y(mm)"=w789, "X(mm)"=w790) -> ()  [unwired: 10 in, 3 out]
              }
            }
            n412 = control-ref of="currentNO"() -> (w782:refnum<vi>)
            n413 = property on="属性节点" class="Str"(reference=w782, "Value"="A2") -> ()  [unwired: 1 in, 2 out]
          }
          event "A3": Value Change {
            n414 = event-data() -> ("NewVal"=w803:bool)  [unwired: 1 in, 5 out]
            n415 = property on="移动" class="Bool (strict)"() -> ("Value"=w806:bool)  [unwired: 2 in, 2 out]
            n416 = Not(x=w806) -> (.not. x?=w805:bool)
            n417 = And(x=w805, y=w803) -> (x .and. y?=w804:bool)
            n418 = case shown="True" w804 {
              frame False {
              }
              frame True {
                n419 = property on="A1-position-X" class="DigNum (strict)"() -> (error out=w810:errorcluster, "Value"=w817:dbl)  [unwired: 2 in, 1 out]
                n420 = property on="A1-position-Y" class="DigNum (strict)"(error in=w810) -> (error out=w809:errorcluster, "Value"=w807:dbl)  [unwired: 1 in, 1 out]
                n421 = Subtract(x=w817, y=9.0) -> (x-y=w808:dbl)
                n422 = vi-ref "goto.vi"() -> (w815:refnum<vi>)
                n423 = property class="VI"(reference=w815, error in=w809) -> ("Name"=w814:string)  [unwired: 2 out]
                n424 = Open VI Reference(type specifier VI Refnum (for type only)=refnum<vi> refnum, vi path=w814, options=128) -> (vi reference=w812:refnum<vi>)  [unwired: 3 in, 1 out]
                n425 = call-by-ref "Start Asynchronous Call"(reference=w812, "Y(mm)"=w807, "X(mm)"=w808) -> ()  [unwired: 10 in, 3 out]
              }
            }
            n426 = control-ref of="currentNO"() -> (w800:refnum<vi>)
            n427 = property on="属性节点" class="Str"(reference=w800, "Value"="A3") -> ()  [unwired: 1 in, 2 out]
          }
          event "A4": Value Change {
            n428 = event-data() -> ("NewVal"=w820:bool)  [unwired: 1 in, 5 out]
            n429 = property on="移动" class="Bool (strict)"() -> ("Value"=w823:bool)  [unwired: 2 in, 2 out]
            n430 = Not(x=w823) -> (.not. x?=w822:bool)
            n431 = And(x=w822, y=w820) -> (x .and. y?=w821:bool)
            n432 = case shown="True" w821 {
              frame False {
              }
              frame True {
                n433 = property on="A1-position-X" class="DigNum (strict)"() -> (error out=w827:errorcluster, "Value"=w834:dbl)  [unwired: 2 in, 1 out]
                n434 = property on="A1-position-Y" class="DigNum (strict)"(error in=w827) -> (error out=w826:errorcluster, "Value"=w824:dbl)  [unwired: 1 in, 1 out]
                n435 = Subtract(x=w834, y=13.5) -> (x-y=w825:dbl)
                n436 = vi-ref "goto.vi"() -> (w832:refnum<vi>)
                n437 = property class="VI"(reference=w832, error in=w826) -> ("Name"=w831:string)  [unwired: 2 out]
                n438 = Open VI Reference(type specifier VI Refnum (for type only)=refnum<vi> refnum, vi path=w831, options=128) -> (vi reference=w829:refnum<vi>)  [unwired: 3 in, 1 out]
                n439 = call-by-ref "Start Asynchronous Call"(reference=w829, "Y(mm)"=w824, "X(mm)"=w825) -> ()  [unwired: 10 in, 3 out]
              }
            }
            n440 = property on="currentNO" class="Str"("Value"="A4") -> ()  [unwired: 2 in, 2 out]
          }
          event "A5": Value Change {
            n441 = event-data() -> ("NewVal"=w837:bool)  [unwired: 1 in, 5 out]
            n442 = property on="移动" class="Bool (strict)"() -> ("Value"=w840:bool)  [unwired: 2 in, 2 out]
            n443 = Not(x=w840) -> (.not. x?=w839:bool)
            n444 = And(x=w839, y=w837) -> (x .and. y?=w838:bool)
            n445 = case shown="True" w838 {
              frame False {
              }
              frame True {
                n446 = property on="A1-position-X" class="DigNum (strict)"() -> (error out=w844:errorcluster, "Value"=w851:dbl)  [unwired: 2 in, 1 out]
                n447 = property on="A1-position-Y" class="DigNum (strict)"(error in=w844) -> (error out=w843:errorcluster, "Value"=w841:dbl)  [unwired: 1 in, 1 out]
                n448 = Subtract(x=w851, y=18) -> (x-y=w842:dbl)
                n449 = vi-ref "goto.vi"() -> (w849:refnum<vi>)
                n450 = property class="VI"(reference=w849, error in=w843) -> ("Name"=w848:string)  [unwired: 2 out]
                n451 = Open VI Reference(type specifier VI Refnum (for type only)=refnum<vi> refnum, vi path=w848, options=128) -> (vi reference=w846:refnum<vi>)  [unwired: 3 in, 1 out]
                n452 = call-by-ref "Start Asynchronous Call"(reference=w846, "Y(mm)"=w841, "X(mm)"=w842) -> ()  [unwired: 10 in, 3 out]
              }
            }
            n453 = property on="currentNO" class="Str"("Value"="A5") -> ()  [unwired: 2 in, 2 out]
          }
          event "A6": Value Change {
            n454 = event-data() -> ("NewVal"=w854:bool)  [unwired: 1 in, 5 out]
            n455 = property on="移动" class="Bool (strict)"() -> ("Value"=w857:bool)  [unwired: 2 in, 2 out]
            n456 = Not(x=w857) -> (.not. x?=w856:bool)
            n457 = And(x=w856, y=w854) -> (x .and. y?=w855:bool)
            n458 = case shown="True" w855 {
              frame False {
              }
              frame True {
                n459 = property on="A1-position-X" class="DigNum (strict)"() -> (error out=w861:errorcluster, "Value"=w868:dbl)  [unwired: 2 in, 1 out]
                n460 = property on="A1-position-Y" class="DigNum (strict)"(error in=w861) -> (error out=w860:errorcluster, "Value"=w858:dbl)  [unwired: 1 in, 1 out]
                n461 = Subtract(x=w868, y=22.5) -> (x-y=w859:dbl)
                n462 = vi-ref "goto.vi"() -> (w866:refnum<vi>)
                n463 = property class="VI"(reference=w866, error in=w860) -> ("Name"=w865:string)  [unwired: 2 out]
                n464 = Open VI Reference(type specifier VI Refnum (for type only)=refnum<vi> refnum, vi path=w865, options=128) -> (vi reference=w863:refnum<vi>)  [unwired: 3 in, 1 out]
                n465 = call-by-ref "Start Asynchronous Call"(reference=w863, "Y(mm)"=w858, "X(mm)"=w859) -> ()  [unwired: 10 in, 3 out]
              }
            }
            n466 = property on="currentNO" class="Str"("Value"="A6") -> ()  [unwired: 2 in, 2 out]
          }
          event "A7": Value Change {
            n467 = event-data() -> ("NewVal"=w871:bool)  [unwired: 1 in, 5 out]
            n468 = property on="移动" class="Bool (strict)"() -> ("Value"=w874:bool)  [unwired: 2 in, 2 out]
            n469 = Not(x=w874) -> (.not. x?=w873:bool)
            n470 = And(x=w873, y=w871) -> (x .and. y?=w872:bool)
            n471 = case shown="True" w872 {
              frame False {
              }
              frame True {
                n472 = property on="A1-position-X" class="DigNum (strict)"() -> (error out=w878:errorcluster, "Value"=w885:dbl)  [unwired: 2 in, 1 out]
                n473 = property on="A1-position-Y" class="DigNum (strict)"(error in=w878) -> (error out=w877:errorcluster, "Value"=w875:dbl)  [unwired: 1 in, 1 out]
                n474 = Subtract(x=w885, y=27) -> (x-y=w876:dbl)
                n475 = vi-ref "goto.vi"() -> (w883:refnum<vi>)
                n476 = property class="VI"(reference=w883, error in=w877) -> ("Name"=w882:string)  [unwired: 2 out]
                n477 = Open VI Reference(type specifier VI Refnum (for type only)=refnum<vi> refnum, vi path=w882, options=128) -> (vi reference=w880:refnum<vi>)  [unwired: 3 in, 1 out]
                n478 = call-by-ref "Start Asynchronous Call"(reference=w880, "Y(mm)"=w875, "X(mm)"=w876) -> ()  [unwired: 10 in, 3 out]
              }
            }
            n479 = property on="currentNO" class="Str"("Value"="A7") -> ()  [unwired: 2 in, 2 out]
          }
          event User Event {
            n480 = event-data() -> ("PV name"=w887:string, "value array (string)"=w886:string[])  [unwired: 1 in, 9 out]
            n481 = case shown="\"ID:STATUS\"" w887 {
              tunnel: w889 -> [w893 w899]
              tunnel: [w893 w902] -> w888
              tunnel: w886 -> [w892 _]
              frame "ID:INFO", Default {
                n482 = Index Array(array=w892, index=0) -> (element=→"idn status":string)
              }
              frame "ID:STATUS" {
                n483 = call "getIOCdata.vi"() -> ("输出簇"=w900:T11)  [unwired: 11 in]
                n484 = call-poly <userlib>:"CaLabGet.vi"("PV Name"="MS:NUM") -> ("1rst Value (number)"=w898:dbl)  [unwired: 8 in, 6 out]
                n485 = Index Array(array=w899, index=w898) -> (element=w897:T11)
                n486 = Unbundle By Name(w897) -> ("NO"=w896:string, "tag2"=w895:string)
                n487 = Bundle By Name(cluster=w900, "NO"=w896, "tag2"=w895) -> (w894:T11)
                n488 = Replace Array Subset "Replace Array Subset"(array=w899, new element=w894, index=w898) -> (w902:T8)
                n489 = for {
                  tunnel: w902 -> [w912] mode=indexing
                  shift-right: [w905] -> w901
                  shift-left: string[][] [] ("Item Names") -> [w907]
                  i -> [w908]
                  n490 = Unbundle By Name(w912) -> ("NO"=w911:string, "tag1"=w910:string, "tag2"=w909:string)
                  n491 = Build Array(w911, w910, w909) -> (w906:string[])
                  n492 = Insert Into Array "Insert Into Array"(array=w907, index (row)=w908, new element=w906) -> (w905:string[][])  [unwired: 1 in]
                }
                n493 = property on="测试记录" class="MCListbox (strict)"("ItemNames"=w901) -> ()  [unwired: 2 in, 2 out]
              }
            }
          }
          event "A8": Value Change {
            n494 = event-data() -> ("NewVal"=w915:bool)  [unwired: 1 in, 5 out]
            n495 = property on="移动" class="Bool (strict)"() -> ("Value"=w918:bool)  [unwired: 2 in, 2 out]
            n496 = Not(x=w918) -> (.not. x?=w917:bool)
            n497 = And(x=w917, y=w915) -> (x .and. y?=w916:bool)
            n498 = case shown="True" w916 {
              frame False {
              }
              frame True {
                n499 = property on="A1-position-X" class="DigNum (strict)"() -> (error out=w922:errorcluster, "Value"=w929:dbl)  [unwired: 2 in, 1 out]
                n500 = property on="A1-position-Y" class="DigNum (strict)"(error in=w922) -> (error out=w921:errorcluster, "Value"=w919:dbl)  [unwired: 1 in, 1 out]
                n501 = Subtract(x=w929, y=31.5) -> (x-y=w920:dbl)
                n502 = vi-ref "goto.vi"() -> (w927:refnum<vi>)
                n503 = property class="VI"(reference=w927, error in=w921) -> ("Name"=w926:string)  [unwired: 2 out]
                n504 = Open VI Reference(type specifier VI Refnum (for type only)=refnum<vi> refnum, vi path=w926, options=128) -> (vi reference=w924:refnum<vi>)  [unwired: 3 in, 1 out]
                n505 = call-by-ref "Start Asynchronous Call"(reference=w924, "Y(mm)"=w919, "X(mm)"=w920) -> ()  [unwired: 10 in, 3 out]
              }
            }
            n506 = property on="currentNO" class="Str"("Value"="A8") -> ()  [unwired: 2 in, 2 out]
          }
          event "A9": Value Change {
            n507 = event-data() -> ("NewVal"=w932:bool)  [unwired: 1 in, 5 out]
            n508 = property on="移动" class="Bool (strict)"() -> ("Value"=w935:bool)  [unwired: 2 in, 2 out]
            n509 = Not(x=w935) -> (.not. x?=w934:bool)
            n510 = And(x=w934, y=w932) -> (x .and. y?=w933:bool)
            n511 = case shown="True" w933 {
              frame False {
              }
              frame True {
                n512 = property on="A1-position-X" class="DigNum (strict)"() -> (error out=w939:errorcluster, "Value"=w946:dbl)  [unwired: 2 in, 1 out]
                n513 = property on="A1-position-Y" class="DigNum (strict)"(error in=w939) -> (error out=w938:errorcluster, "Value"=w936:dbl)  [unwired: 1 in, 1 out]
                n514 = Subtract(x=w946, y=36) -> (x-y=w937:dbl)
                n515 = vi-ref "goto.vi"() -> (w944:refnum<vi>)
                n516 = property class="VI"(reference=w944, error in=w938) -> ("Name"=w943:string)  [unwired: 2 out]
                n517 = Open VI Reference(type specifier VI Refnum (for type only)=refnum<vi> refnum, vi path=w943, options=128) -> (vi reference=w941:refnum<vi>)  [unwired: 3 in, 1 out]
                n518 = call-by-ref "Start Asynchronous Call"(reference=w941, "Y(mm)"=w936, "X(mm)"=w937) -> ()  [unwired: 10 in, 3 out]
              }
            }
            n519 = property on="currentNO" class="Str"("Value"="A9") -> ()  [unwired: 2 in, 2 out]
          }
          event "A10": Value Change {
            n520 = event-data() -> ("NewVal"=w949:bool)  [unwired: 1 in, 5 out]
            n521 = property on="移动" class="Bool (strict)"() -> ("Value"=w952:bool)  [unwired: 2 in, 2 out]
            n522 = Not(x=w952) -> (.not. x?=w951:bool)
            n523 = And(x=w951, y=w949) -> (x .and. y?=w950:bool)
            n524 = case shown="True" w950 {
              frame False {
              }
              frame True {
                n525 = property on="A1-position-X" class="DigNum (strict)"() -> (error out=w956:errorcluster, "Value"=w963:dbl)  [unwired: 2 in, 1 out]
                n526 = property on="A1-position-Y" class="DigNum (strict)"(error in=w956) -> (error out=w955:errorcluster, "Value"=w953:dbl)  [unwired: 1 in, 1 out]
                n527 = Subtract(x=w963, y=40.5) -> (x-y=w954:dbl)
                n528 = vi-ref "goto.vi"() -> (w961:refnum<vi>)
                n529 = property class="VI"(reference=w961, error in=w955) -> ("Name"=w960:string)  [unwired: 2 out]
                n530 = Open VI Reference(type specifier VI Refnum (for type only)=refnum<vi> refnum, vi path=w960, options=128) -> (vi reference=w958:refnum<vi>)  [unwired: 3 in, 1 out]
                n531 = call-by-ref "Start Asynchronous Call"(reference=w958, "Y(mm)"=w953, "X(mm)"=w954) -> ()  [unwired: 10 in, 3 out]
              }
            }
            n532 = property on="currentNO" class="Str"("Value"="A10") -> ()  [unwired: 2 in, 2 out]
          }
          event "A11": Value Change {
            n533 = event-data() -> ("NewVal"=w966:bool)  [unwired: 1 in, 5 out]
            n534 = property on="移动" class="Bool (strict)"() -> ("Value"=w969:bool)  [unwired: 2 in, 2 out]
            n535 = Not(x=w969) -> (.not. x?=w968:bool)
            n536 = And(x=w968, y=w966) -> (x .and. y?=w967:bool)
            n537 = case shown="True" w967 {
              frame False {
              }
              frame True {
                n538 = property on="A1-position-X" class="DigNum (strict)"() -> (error out=w973:errorcluster, "Value"=w980:dbl)  [unwired: 2 in, 1 out]
                n539 = property on="A1-position-Y" class="DigNum (strict)"(error in=w973) -> (error out=w972:errorcluster, "Value"=w970:dbl)  [unwired: 1 in, 1 out]
                n540 = Subtract(x=w980, y=45) -> (x-y=w971:dbl)
                n541 = vi-ref "goto.vi"() -> (w978:refnum<vi>)
                n542 = property class="VI"(reference=w978, error in=w972) -> ("Name"=w977:string)  [unwired: 2 out]
                n543 = Open VI Reference(type specifier VI Refnum (for type only)=refnum<vi> refnum, vi path=w977, options=128) -> (vi reference=w975:refnum<vi>)  [unwired: 3 in, 1 out]
                n544 = call-by-ref "Start Asynchronous Call"(reference=w975, "Y(mm)"=w970, "X(mm)"=w971) -> ()  [unwired: 10 in, 3 out]
              }
            }
            n545 = property on="currentNO" class="Str"("Value"="A11") -> ()  [unwired: 2 in, 2 out]
          }
          event "A12": Value Change {
            n546 = event-data() -> ("NewVal"=w983:bool)  [unwired: 1 in, 5 out]
            n547 = property on="移动" class="Bool (strict)"() -> ("Value"=w986:bool)  [unwired: 2 in, 2 out]
            n548 = Not(x=w986) -> (.not. x?=w985:bool)
            n549 = And(x=w985, y=w983) -> (x .and. y?=w984:bool)
            n550 = case shown="True" w984 {
              frame False {
              }
              frame True {
                n551 = property on="A1-position-X" class="DigNum (strict)"() -> (error out=w990:errorcluster, "Value"=w997:dbl)  [unwired: 2 in, 1 out]
                n552 = property on="A1-position-Y" class="DigNum (strict)"(error in=w990) -> (error out=w989:errorcluster, "Value"=w987:dbl)  [unwired: 1 in, 1 out]
                n553 = Subtract(x=w997, y=49.5) -> (x-y=w988:dbl)
                n554 = vi-ref "goto.vi"() -> (w995:refnum<vi>)
                n555 = property class="VI"(reference=w995, error in=w989) -> ("Name"=w994:string)  [unwired: 2 out]
                n556 = Open VI Reference(type specifier VI Refnum (for type only)=refnum<vi> refnum, vi path=w994, options=128) -> (vi reference=w992:refnum<vi>)  [unwired: 3 in, 1 out]
                n557 = call-by-ref "Start Asynchronous Call"(reference=w992, "Y(mm)"=w987, "X(mm)"=w988) -> ()  [unwired: 10 in, 3 out]
              }
            }
            n558 = property on="currentNO" class="Str"("Value"="A12") -> ()  [unwired: 2 in, 2 out]
          }
          event "B1": Value Change {
            n559 = event-data() -> ("NewVal"=w1000:bool)  [unwired: 1 in, 5 out]
            n560 = property on="移动" class="Bool (strict)"() -> ("Value"=w1003:bool)  [unwired: 2 in, 2 out]
            n561 = Not(x=w1003) -> (.not. x?=w1002:bool)
            n562 = And(x=w1002, y=w1000) -> (x .and. y?=w1001:bool)
            n563 = case shown="True" w1001 {
              frame False {
              }
              frame True {
                n564 = property on="A1-position-X" class="DigNum (strict)"() -> (error out=w1009:errorcluster, "Value"=w1016:dbl)  [unwired: 2 in, 1 out]
                n565 = property on="A1-position-Y" class="DigNum (strict)"(error in=w1009) -> (error out=w1008:errorcluster, "Value"=w1005:dbl)  [unwired: 1 in, 1 out]
                n566 = Subtract(x=w1005, y=4.5) -> (x-y=w1004:dbl)
                n567 = Subtract(x=w1016, y=0) -> (x-y=w1007:dbl)
                n568 = vi-ref "goto.vi"() -> (w1014:refnum<vi>)
                n569 = property class="VI"(reference=w1014, error in=w1008) -> ("Name"=w1013:string)  [unwired: 2 out]
                n570 = Open VI Reference(type specifier VI Refnum (for type only)=refnum<vi> refnum, vi path=w1013, options=128) -> (vi reference=w1011:refnum<vi>)  [unwired: 3 in, 1 out]
                n571 = call-by-ref "Start Asynchronous Call"(reference=w1011, "Y(mm)"=w1004, "X(mm)"=w1007) -> ()  [unwired: 10 in, 3 out]
              }
            }
            n572 = property on="currentNO" class="Str"("Value"="B1") -> ()  [unwired: 2 in, 2 out]
          }
          event "B2": Value Change {
            n573 = event-data() -> ("NewVal"=w1019:bool)  [unwired: 1 in, 5 out]
            n574 = property on="移动" class="Bool (strict)"() -> ("Value"=w1022:bool)  [unwired: 2 in, 2 out]
            n575 = Not(x=w1022) -> (.not. x?=w1021:bool)
            n576 = And(x=w1021, y=w1019) -> (x .and. y?=w1020:bool)
            n577 = case shown="True" w1020 {
              frame False {
              }
              frame True {
                n578 = property on="A1-position-X" class="DigNum (strict)"() -> (error out=w1028:errorcluster, "Value"=w1035:dbl)  [unwired: 2 in, 1 out]
                n579 = property on="A1-position-Y" class="DigNum (strict)"(error in=w1028) -> (error out=w1027:errorcluster, "Value"=w1024:dbl)  [unwired: 1 in, 1 out]
                n580 = Subtract(x=w1024, y=4.5) -> (x-y=w1023:dbl)
                n581 = Subtract(x=w1035, y=4.5) -> (x-y=w1026:dbl)
                n582 = vi-ref "goto.vi"() -> (w1033:refnum<vi>)
                n583 = property class="VI"(reference=w1033, error in=w1027) -> ("Name"=w1032:string)  [unwired: 2 out]
                n584 = Open VI Reference(type specifier VI Refnum (for type only)=refnum<vi> refnum, vi path=w1032, options=128) -> (vi reference=w1030:refnum<vi>)  [unwired: 3 in, 1 out]
                n585 = call-by-ref "Start Asynchronous Call"(reference=w1030, "Y(mm)"=w1023, "X(mm)"=w1026) -> ()  [unwired: 10 in, 3 out]
              }
            }
            n586 = property on="currentNO" class="Str"("Value"="B2") -> ()  [unwired: 2 in, 2 out]
          }
          event "B3": Value Change {
            n587 = event-data() -> ("NewVal"=w1038:bool)  [unwired: 1 in, 5 out]
            n588 = property on="移动" class="Bool (strict)"() -> ("Value"=w1041:bool)  [unwired: 2 in, 2 out]
            n589 = Not(x=w1041) -> (.not. x?=w1040:bool)
            n590 = And(x=w1040, y=w1038) -> (x .and. y?=w1039:bool)
            n591 = case shown="True" w1039 {
              frame False {
              }
              frame True {
                n592 = property on="A1-position-X" class="DigNum (strict)"() -> (error out=w1047:errorcluster, "Value"=w1054:dbl)  [unwired: 2 in, 1 out]
                n593 = property on="A1-position-Y" class="DigNum (strict)"(error in=w1047) -> (error out=w1046:errorcluster, "Value"=w1043:dbl)  [unwired: 1 in, 1 out]
                n594 = Subtract(x=w1043, y=4.5) -> (x-y=w1042:dbl)
                n595 = Subtract(x=w1054, y=9) -> (x-y=w1045:dbl)
                n596 = vi-ref "goto.vi"() -> (w1052:refnum<vi>)
                n597 = property class="VI"(reference=w1052, error in=w1046) -> ("Name"=w1051:string)  [unwired: 2 out]
                n598 = Open VI Reference(type specifier VI Refnum (for type only)=refnum<vi> refnum, vi path=w1051, options=128) -> (vi reference=w1049:refnum<vi>)  [unwired: 3 in, 1 out]
                n599 = call-by-ref "Start Asynchronous Call"(reference=w1049, "Y(mm)"=w1042, "X(mm)"=w1045) -> ()  [unwired: 10 in, 3 out]
              }
            }
            n600 = property on="currentNO" class="Str"("Value"="B3") -> ()  [unwired: 2 in, 2 out]
          }
          event "B4": Value Change {
            n601 = event-data() -> ("NewVal"=w1057:bool)  [unwired: 1 in, 5 out]
            n602 = property on="移动" class="Bool (strict)"() -> ("Value"=w1060:bool)  [unwired: 2 in, 2 out]
            n603 = Not(x=w1060) -> (.not. x?=w1059:bool)
            n604 = And(x=w1059, y=w1057) -> (x .and. y?=w1058:bool)
            n605 = case shown="True" w1058 {
              frame False {
              }
              frame True {
                n606 = property on="A1-position-X" class="DigNum (strict)"() -> (error out=w1066:errorcluster, "Value"=w1073:dbl)  [unwired: 2 in, 1 out]
                n607 = property on="A1-position-Y" class="DigNum (strict)"(error in=w1066) -> (error out=w1065:errorcluster, "Value"=w1062:dbl)  [unwired: 1 in, 1 out]
                n608 = Subtract(x=w1062, y=4.5) -> (x-y=w1061:dbl)
                n609 = Subtract(x=w1073, y=13.5) -> (x-y=w1064:dbl)
                n610 = vi-ref "goto.vi"() -> (w1071:refnum<vi>)
                n611 = property class="VI"(reference=w1071, error in=w1065) -> ("Name"=w1070:string)  [unwired: 2 out]
                n612 = Open VI Reference(type specifier VI Refnum (for type only)=refnum<vi> refnum, vi path=w1070, options=128) -> (vi reference=w1068:refnum<vi>)  [unwired: 3 in, 1 out]
                n613 = call-by-ref "Start Asynchronous Call"(reference=w1068, "Y(mm)"=w1061, "X(mm)"=w1064) -> ()  [unwired: 10 in, 3 out]
              }
            }
            n614 = property on="currentNO" class="Str"("Value"="B4") -> ()  [unwired: 2 in, 2 out]
          }
          event "B5": Value Change {
            n615 = event-data() -> ("NewVal"=w1076:bool)  [unwired: 1 in, 5 out]
            n616 = property on="移动" class="Bool (strict)"() -> ("Value"=w1079:bool)  [unwired: 2 in, 2 out]
            n617 = Not(x=w1079) -> (.not. x?=w1078:bool)
            n618 = And(x=w1078, y=w1076) -> (x .and. y?=w1077:bool)
            n619 = case shown="True" w1077 {
              frame False {
              }
              frame True {
                n620 = property on="A1-position-X" class="DigNum (strict)"() -> (error out=w1085:errorcluster, "Value"=w1092:dbl)  [unwired: 2 in, 1 out]
                n621 = property on="A1-position-Y" class="DigNum (strict)"(error in=w1085) -> (error out=w1084:errorcluster, "Value"=w1081:dbl)  [unwired: 1 in, 1 out]
                n622 = Subtract(x=w1081, y=4.5) -> (x-y=w1080:dbl)
                n623 = Subtract(x=w1092, y=18) -> (x-y=w1083:dbl)
                n624 = vi-ref "goto.vi"() -> (w1090:refnum<vi>)
                n625 = property class="VI"(reference=w1090, error in=w1084) -> ("Name"=w1089:string)  [unwired: 2 out]
                n626 = Open VI Reference(type specifier VI Refnum (for type only)=refnum<vi> refnum, vi path=w1089, options=128) -> (vi reference=w1087:refnum<vi>)  [unwired: 3 in, 1 out]
                n627 = call-by-ref "Start Asynchronous Call"(reference=w1087, "Y(mm)"=w1080, "X(mm)"=w1083) -> ()  [unwired: 10 in, 3 out]
              }
            }
            n628 = property on="currentNO" class="Str"("Value"="B5") -> ()  [unwired: 2 in, 2 out]
          }
          event "B6": Value Change {
            n629 = event-data() -> ("NewVal"=w1095:bool)  [unwired: 1 in, 5 out]
            n630 = property on="移动" class="Bool (strict)"() -> ("Value"=w1098:bool)  [unwired: 2 in, 2 out]
            n631 = Not(x=w1098) -> (.not. x?=w1097:bool)
            n632 = And(x=w1097, y=w1095) -> (x .and. y?=w1096:bool)
            n633 = case shown="True" w1096 {
              frame False {
              }
              frame True {
                n634 = property on="A1-position-X" class="DigNum (strict)"() -> (error out=w1104:errorcluster, "Value"=w1111:dbl)  [unwired: 2 in, 1 out]
                n635 = property on="A1-position-Y" class="DigNum (strict)"(error in=w1104) -> (error out=w1103:errorcluster, "Value"=w1100:dbl)  [unwired: 1 in, 1 out]
                n636 = Subtract(x=w1100, y=4.5) -> (x-y=w1099:dbl)
                n637 = Subtract(x=w1111, y=22.5) -> (x-y=w1102:dbl)
                n638 = vi-ref "goto.vi"() -> (w1109:refnum<vi>)
                n639 = property class="VI"(reference=w1109, error in=w1103) -> ("Name"=w1108:string)  [unwired: 2 out]
                n640 = Open VI Reference(type specifier VI Refnum (for type only)=refnum<vi> refnum, vi path=w1108, options=128) -> (vi reference=w1106:refnum<vi>)  [unwired: 3 in, 1 out]
                n641 = call-by-ref "Start Asynchronous Call"(reference=w1106, "Y(mm)"=w1099, "X(mm)"=w1102) -> ()  [unwired: 10 in, 3 out]
              }
            }
            n642 = property on="currentNO" class="Str"("Value"="B6") -> ()  [unwired: 2 in, 2 out]
          }
          event "B7": Value Change {
            n643 = event-data() -> ("NewVal"=w1113:bool)  [unwired: 1 in, 5 out]
            n644 = property on="移动" class="Bool (strict)"() -> ("Value"=w1116:bool)  [unwired: 2 in, 2 out]
            n645 = Not(x=w1116) -> (.not. x?=w1115:bool)
            n646 = And(x=w1115, y=w1113) -> (x .and. y?=w1114:bool)
            n647 = case shown="True" w1114 {
              frame False {
              }
              frame True {
                n648 = property on="A1-position-X" class="DigNum (strict)"() -> (error out=w1122:errorcluster, "Value"=w1129:dbl)  [unwired: 2 in, 1 out]
                n649 = property on="A1-position-Y" class="DigNum (strict)"(error in=w1122) -> (error out=w1121:errorcluster, "Value"=w1118:dbl)  [unwired: 1 in, 1 out]
                n650 = Subtract(x=w1118, y=4.5) -> (x-y=w1117:dbl)
                n651 = Subtract(x=w1129, y=27) -> (x-y=w1120:dbl)
                n652 = vi-ref "goto.vi"() -> (w1127:refnum<vi>)
                n653 = property class="VI"(reference=w1127, error in=w1121) -> ("Name"=w1126:string)  [unwired: 2 out]
                n654 = Open VI Reference(type specifier VI Refnum (for type only)=refnum<vi> refnum, vi path=w1126, options=128) -> (vi reference=w1124:refnum<vi>)  [unwired: 3 in, 1 out]
                n655 = call-by-ref "Start Asynchronous Call"(reference=w1124, "Y(mm)"=w1117, "X(mm)"=w1120) -> ()  [unwired: 10 in, 3 out]
              }
            }
          }
          event "B8": Value Change {
            n656 = event-data() -> ("NewVal"=w1131:bool)  [unwired: 1 in, 5 out]
            n657 = property on="移动" class="Bool (strict)"() -> ("Value"=w1134:bool)  [unwired: 2 in, 2 out]
            n658 = Not(x=w1134) -> (.not. x?=w1133:bool)
            n659 = And(x=w1133, y=w1131) -> (x .and. y?=w1132:bool)
            n660 = case shown="True" w1132 {
              frame False {
              }
              frame True {
                n661 = property on="A1-position-X" class="DigNum (strict)"() -> (error out=w1140:errorcluster, "Value"=w1147:dbl)  [unwired: 2 in, 1 out]
                n662 = property on="A1-position-Y" class="DigNum (strict)"(error in=w1140) -> (error out=w1139:errorcluster, "Value"=w1136:dbl)  [unwired: 1 in, 1 out]
                n663 = Subtract(x=w1136, y=4.5) -> (x-y=w1135:dbl)
                n664 = Subtract(x=w1147, y=31.5) -> (x-y=w1138:dbl)
                n665 = vi-ref "goto.vi"() -> (w1145:refnum<vi>)
                n666 = property class="VI"(reference=w1145, error in=w1139) -> ("Name"=w1144:string)  [unwired: 2 out]
                n667 = Open VI Reference(type specifier VI Refnum (for type only)=refnum<vi> refnum, vi path=w1144, options=128) -> (vi reference=w1142:refnum<vi>)  [unwired: 3 in, 1 out]
                n668 = call-by-ref "Start Asynchronous Call"(reference=w1142, "Y(mm)"=w1135, "X(mm)"=w1138) -> ()  [unwired: 10 in, 3 out]
              }
            }
          }
          event "B9": Value Change {
            n669 = event-data() -> ("NewVal"=w1149:bool)  [unwired: 1 in, 5 out]
            n670 = property on="移动" class="Bool (strict)"() -> ("Value"=w1152:bool)  [unwired: 2 in, 2 out]
            n671 = Not(x=w1152) -> (.not. x?=w1151:bool)
            n672 = And(x=w1151, y=w1149) -> (x .and. y?=w1150:bool)
            n673 = case shown="True" w1150 {
              frame False {
              }
              frame True {
                n674 = property on="A1-position-X" class="DigNum (strict)"() -> (error out=w1158:errorcluster, "Value"=w1165:dbl)  [unwired: 2 in, 1 out]
                n675 = property on="A1-position-Y" class="DigNum (strict)"(error in=w1158) -> (error out=w1157:errorcluster, "Value"=w1154:dbl)  [unwired: 1 in, 1 out]
                n676 = Subtract(x=w1154, y=4.5) -> (x-y=w1153:dbl)
                n677 = Subtract(x=w1165, y=36) -> (x-y=w1156:dbl)
                n678 = vi-ref "goto.vi"() -> (w1163:refnum<vi>)
                n679 = property class="VI"(reference=w1163, error in=w1157) -> ("Name"=w1162:string)  [unwired: 2 out]
                n680 = Open VI Reference(type specifier VI Refnum (for type only)=refnum<vi> refnum, vi path=w1162, options=128) -> (vi reference=w1160:refnum<vi>)  [unwired: 3 in, 1 out]
                n681 = call-by-ref "Start Asynchronous Call"(reference=w1160, "Y(mm)"=w1153, "X(mm)"=w1156) -> ()  [unwired: 10 in, 3 out]
              }
            }
          }
          event "B10": Value Change {
            n682 = event-data() -> ("NewVal"=w1167:bool)  [unwired: 1 in, 5 out]
            n683 = property on="移动" class="Bool (strict)"() -> ("Value"=w1170:bool)  [unwired: 2 in, 2 out]
            n684 = Not(x=w1170) -> (.not. x?=w1169:bool)
            n685 = And(x=w1169, y=w1167) -> (x .and. y?=w1168:bool)
            n686 = case shown="True" w1168 {
              frame False {
              }
              frame True {
                n687 = property on="A1-position-X" class="DigNum (strict)"() -> (error out=w1176:errorcluster, "Value"=w1183:dbl)  [unwired: 2 in, 1 out]
                n688 = property on="A1-position-Y" class="DigNum (strict)"(error in=w1176) -> (error out=w1175:errorcluster, "Value"=w1172:dbl)  [unwired: 1 in, 1 out]
                n689 = Subtract(x=w1172, y=4.5) -> (x-y=w1171:dbl)
                n690 = Subtract(x=w1183, y=40.5) -> (x-y=w1174:dbl)
                n691 = vi-ref "goto.vi"() -> (w1181:refnum<vi>)
                n692 = property class="VI"(reference=w1181, error in=w1175) -> ("Name"=w1180:string)  [unwired: 2 out]
                n693 = Open VI Reference(type specifier VI Refnum (for type only)=refnum<vi> refnum, vi path=w1180, options=128) -> (vi reference=w1178:refnum<vi>)  [unwired: 3 in, 1 out]
                n694 = call-by-ref "Start Asynchronous Call"(reference=w1178, "Y(mm)"=w1171, "X(mm)"=w1174) -> ()  [unwired: 10 in, 3 out]
              }
            }
          }
          event "B11": Value Change {
            n695 = event-data() -> ("NewVal"=w1185:bool)  [unwired: 1 in, 5 out]
            n696 = property on="移动" class="Bool (strict)"() -> ("Value"=w1188:bool)  [unwired: 2 in, 2 out]
            n697 = Not(x=w1188) -> (.not. x?=w1187:bool)
            n698 = And(x=w1187, y=w1185) -> (x .and. y?=w1186:bool)
            n699 = case shown="True" w1186 {
              frame False {
              }
              frame True {
                n700 = property on="A1-position-X" class="DigNum (strict)"() -> (error out=w1194:errorcluster, "Value"=w1201:dbl)  [unwired: 2 in, 1 out]
                n701 = property on="A1-position-Y" class="DigNum (strict)"(error in=w1194) -> (error out=w1193:errorcluster, "Value"=w1190:dbl)  [unwired: 1 in, 1 out]
                n702 = Subtract(x=w1190, y=4.5) -> (x-y=w1189:dbl)
                n703 = Subtract(x=w1201, y=45) -> (x-y=w1192:dbl)
                n704 = vi-ref "goto.vi"() -> (w1199:refnum<vi>)
                n705 = property class="VI"(reference=w1199, error in=w1193) -> ("Name"=w1198:string)  [unwired: 2 out]
                n706 = Open VI Reference(type specifier VI Refnum (for type only)=refnum<vi> refnum, vi path=w1198, options=128) -> (vi reference=w1196:refnum<vi>)  [unwired: 3 in, 1 out]
                n707 = call-by-ref "Start Asynchronous Call"(reference=w1196, "Y(mm)"=w1189, "X(mm)"=w1192) -> ()  [unwired: 10 in, 3 out]
              }
            }
          }
          event "B12": Value Change {
            n708 = event-data() -> ("NewVal"=w1203:bool)  [unwired: 1 in, 5 out]
            n709 = property on="移动" class="Bool (strict)"() -> ("Value"=w1206:bool)  [unwired: 2 in, 2 out]
            n710 = Not(x=w1206) -> (.not. x?=w1205:bool)
            n711 = And(x=w1205, y=w1203) -> (x .and. y?=w1204:bool)
            n712 = case shown="True" w1204 {
              frame False {
              }
              frame True {
                n713 = property on="A1-position-X" class="DigNum (strict)"() -> (error out=w1212:errorcluster, "Value"=w1219:dbl)  [unwired: 2 in, 1 out]
                n714 = property on="A1-position-Y" class="DigNum (strict)"(error in=w1212) -> (error out=w1211:errorcluster, "Value"=w1208:dbl)  [unwired: 1 in, 1 out]
                n715 = Subtract(x=w1208, y=4.5) -> (x-y=w1207:dbl)
                n716 = Subtract(x=w1219, y=49.5) -> (x-y=w1210:dbl)
                n717 = vi-ref "goto.vi"() -> (w1217:refnum<vi>)
                n718 = property class="VI"(reference=w1217, error in=w1211) -> ("Name"=w1216:string)  [unwired: 2 out]
                n719 = Open VI Reference(type specifier VI Refnum (for type only)=refnum<vi> refnum, vi path=w1216, options=128) -> (vi reference=w1214:refnum<vi>)  [unwired: 3 in, 1 out]
                n720 = call-by-ref "Start Asynchronous Call"(reference=w1214, "Y(mm)"=w1207, "X(mm)"=w1210) -> ()  [unwired: 10 in, 3 out]
              }
            }
          }
          event "C1": Value Change {
            n721 = event-data() -> ("NewVal"=w1221:bool)  [unwired: 1 in, 5 out]
            n722 = property on="移动" class="Bool (strict)"() -> ("Value"=w1224:bool)  [unwired: 2 in, 2 out]
            n723 = Not(x=w1224) -> (.not. x?=w1223:bool)
            n724 = And(x=w1223, y=w1221) -> (x .and. y?=w1222:bool)
            n725 = case shown="True" w1222 {
              frame False {
              }
              frame True {
                n726 = property on="A1-position-X" class="DigNum (strict)"() -> (error out=w1230:errorcluster, "Value"=w1237:dbl)  [unwired: 2 in, 1 out]
                n727 = property on="A1-position-Y" class="DigNum (strict)"(error in=w1230) -> (error out=w1229:errorcluster, "Value"=w1226:dbl)  [unwired: 1 in, 1 out]
                n728 = Subtract(x=w1226, y=9) -> (x-y=w1225:dbl)
                n729 = Subtract(x=w1237, y=0) -> (x-y=w1228:dbl)
                n730 = vi-ref "goto.vi"() -> (w1235:refnum<vi>)
                n731 = property class="VI"(reference=w1235, error in=w1229) -> ("Name"=w1234:string)  [unwired: 2 out]
                n732 = Open VI Reference(type specifier VI Refnum (for type only)=refnum<vi> refnum, vi path=w1234, options=128) -> (vi reference=w1232:refnum<vi>)  [unwired: 3 in, 1 out]
                n733 = call-by-ref "Start Asynchronous Call"(reference=w1232, "Y(mm)"=w1225, "X(mm)"=w1228) -> ()  [unwired: 10 in, 3 out]
              }
            }
          }
          event "C2": Value Change {
            n734 = event-data() -> ("NewVal"=w1239:bool)  [unwired: 1 in, 5 out]
            n735 = property on="移动" class="Bool (strict)"() -> ("Value"=w1242:bool)  [unwired: 2 in, 2 out]
            n736 = Not(x=w1242) -> (.not. x?=w1241:bool)
            n737 = And(x=w1241, y=w1239) -> (x .and. y?=w1240:bool)
            n738 = case shown="True" w1240 {
              frame False {
              }
              frame True {
                n739 = property on="A1-position-X" class="DigNum (strict)"() -> (error out=w1248:errorcluster, "Value"=w1255:dbl)  [unwired: 2 in, 1 out]
                n740 = property on="A1-position-Y" class="DigNum (strict)"(error in=w1248) -> (error out=w1247:errorcluster, "Value"=w1244:dbl)  [unwired: 1 in, 1 out]
                n741 = Subtract(x=w1244, y=9) -> (x-y=w1243:dbl)
                n742 = Subtract(x=w1255, y=4.5) -> (x-y=w1246:dbl)
                n743 = vi-ref "goto.vi"() -> (w1253:refnum<vi>)
                n744 = property class="VI"(reference=w1253, error in=w1247) -> ("Name"=w1252:string)  [unwired: 2 out]
                n745 = Open VI Reference(type specifier VI Refnum (for type only)=refnum<vi> refnum, vi path=w1252, options=128) -> (vi reference=w1250:refnum<vi>)  [unwired: 3 in, 1 out]
                n746 = call-by-ref "Start Asynchronous Call"(reference=w1250, "Y(mm)"=w1243, "X(mm)"=w1246) -> ()  [unwired: 10 in, 3 out]
              }
            }
          }
          event "C3": Value Change {
            n747 = event-data() -> ("NewVal"=w1257:bool)  [unwired: 1 in, 5 out]
            n748 = property on="移动" class="Bool (strict)"() -> ("Value"=w1260:bool)  [unwired: 2 in, 2 out]
            n749 = Not(x=w1260) -> (.not. x?=w1259:bool)
            n750 = And(x=w1259, y=w1257) -> (x .and. y?=w1258:bool)
            n751 = case shown="True" w1258 {
              frame False {
              }
              frame True {
                n752 = property on="A1-position-X" class="DigNum (strict)"() -> (error out=w1266:errorcluster, "Value"=w1273:dbl)  [unwired: 2 in, 1 out]
                n753 = property on="A1-position-Y" class="DigNum (strict)"(error in=w1266) -> (error out=w1265:errorcluster, "Value"=w1262:dbl)  [unwired: 1 in, 1 out]
                n754 = Subtract(x=w1262, y=9) -> (x-y=w1261:dbl)
                n755 = Subtract(x=w1273, y=9) -> (x-y=w1264:dbl)
                n756 = vi-ref "goto.vi"() -> (w1271:refnum<vi>)
                n757 = property class="VI"(reference=w1271, error in=w1265) -> ("Name"=w1270:string)  [unwired: 2 out]
                n758 = Open VI Reference(type specifier VI Refnum (for type only)=refnum<vi> refnum, vi path=w1270, options=128) -> (vi reference=w1268:refnum<vi>)  [unwired: 3 in, 1 out]
                n759 = call-by-ref "Start Asynchronous Call"(reference=w1268, "Y(mm)"=w1261, "X(mm)"=w1264) -> ()  [unwired: 10 in, 3 out]
              }
            }
          }
          event "C4": Value Change {
            n760 = event-data() -> ("NewVal"=w1275:bool)  [unwired: 1 in, 5 out]
            n761 = property on="移动" class="Bool (strict)"() -> ("Value"=w1278:bool)  [unwired: 2 in, 2 out]
            n762 = Not(x=w1278) -> (.not. x?=w1277:bool)
            n763 = And(x=w1277, y=w1275) -> (x .and. y?=w1276:bool)
            n764 = case shown="True" w1276 {
              frame False {
              }
              frame True {
                n765 = property on="A1-position-X" class="DigNum (strict)"() -> (error out=w1284:errorcluster, "Value"=w1291:dbl)  [unwired: 2 in, 1 out]
                n766 = property on="A1-position-Y" class="DigNum (strict)"(error in=w1284) -> (error out=w1283:errorcluster, "Value"=w1280:dbl)  [unwired: 1 in, 1 out]
                n767 = Subtract(x=w1280, y=9) -> (x-y=w1279:dbl)
                n768 = Subtract(x=w1291, y=13.5) -> (x-y=w1282:dbl)
                n769 = vi-ref "goto.vi"() -> (w1289:refnum<vi>)
                n770 = property class="VI"(reference=w1289, error in=w1283) -> ("Name"=w1288:string)  [unwired: 2 out]
                n771 = Open VI Reference(type specifier VI Refnum (for type only)=refnum<vi> refnum, vi path=w1288, options=128) -> (vi reference=w1286:refnum<vi>)  [unwired: 3 in, 1 out]
                n772 = call-by-ref "Start Asynchronous Call"(reference=w1286, "Y(mm)"=w1279, "X(mm)"=w1282) -> ()  [unwired: 10 in, 3 out]
              }
            }
          }
          event "C5": Value Change {
            n773 = event-data() -> ("NewVal"=w1293:bool)  [unwired: 1 in, 5 out]
            n774 = property on="移动" class="Bool (strict)"() -> ("Value"=w1296:bool)  [unwired: 2 in, 2 out]
            n775 = Not(x=w1296) -> (.not. x?=w1295:bool)
            n776 = And(x=w1295, y=w1293) -> (x .and. y?=w1294:bool)
            n777 = case shown="True" w1294 {
              frame False {
              }
              frame True {
                n778 = property on="A1-position-X" class="DigNum (strict)"() -> (error out=w1302:errorcluster, "Value"=w1309:dbl)  [unwired: 2 in, 1 out]
                n779 = property on="A1-position-Y" class="DigNum (strict)"(error in=w1302) -> (error out=w1301:errorcluster, "Value"=w1298:dbl)  [unwired: 1 in, 1 out]
                n780 = Subtract(x=w1298, y=9) -> (x-y=w1297:dbl)
                n781 = Subtract(x=w1309, y=18) -> (x-y=w1300:dbl)
                n782 = vi-ref "goto.vi"() -> (w1307:refnum<vi>)
                n783 = property class="VI"(reference=w1307, error in=w1301) -> ("Name"=w1306:string)  [unwired: 2 out]
                n784 = Open VI Reference(type specifier VI Refnum (for type only)=refnum<vi> refnum, vi path=w1306, options=128) -> (vi reference=w1304:refnum<vi>)  [unwired: 3 in, 1 out]
                n785 = call-by-ref "Start Asynchronous Call"(reference=w1304, "Y(mm)"=w1297, "X(mm)"=w1300) -> ()  [unwired: 10 in, 3 out]
              }
            }
          }
          event "C6": Value Change {
            n786 = event-data() -> ("NewVal"=w1311:bool)  [unwired: 1 in, 5 out]
            n787 = property on="移动" class="Bool (strict)"() -> ("Value"=w1314:bool)  [unwired: 2 in, 2 out]
            n788 = Not(x=w1314) -> (.not. x?=w1313:bool)
            n789 = And(x=w1313, y=w1311) -> (x .and. y?=w1312:bool)
            n790 = case shown="True" w1312 {
              frame False {
              }
              frame True {
                n791 = property on="A1-position-X" class="DigNum (strict)"() -> (error out=w1320:errorcluster, "Value"=w1327:dbl)  [unwired: 2 in, 1 out]
                n792 = property on="A1-position-Y" class="DigNum (strict)"(error in=w1320) -> (error out=w1319:errorcluster, "Value"=w1316:dbl)  [unwired: 1 in, 1 out]
                n793 = Subtract(x=w1316, y=9) -> (x-y=w1315:dbl)
                n794 = Subtract(x=w1327, y=22.5) -> (x-y=w1318:dbl)
                n795 = vi-ref "goto.vi"() -> (w1325:refnum<vi>)
                n796 = property class="VI"(reference=w1325, error in=w1319) -> ("Name"=w1324:string)  [unwired: 2 out]
                n797 = Open VI Reference(type specifier VI Refnum (for type only)=refnum<vi> refnum, vi path=w1324, options=128) -> (vi reference=w1322:refnum<vi>)  [unwired: 3 in, 1 out]
                n798 = call-by-ref "Start Asynchronous Call"(reference=w1322, "Y(mm)"=w1315, "X(mm)"=w1318) -> ()  [unwired: 10 in, 3 out]
              }
            }
          }
          event "C7": Value Change {
            n799 = event-data() -> ("NewVal"=w1329:bool)  [unwired: 1 in, 5 out]
            n800 = property on="移动" class="Bool (strict)"() -> ("Value"=w1332:bool)  [unwired: 2 in, 2 out]
            n801 = Not(x=w1332) -> (.not. x?=w1331:bool)
            n802 = And(x=w1331, y=w1329) -> (x .and. y?=w1330:bool)
            n803 = case shown="True" w1330 {
              frame False {
              }
              frame True {
                n804 = property on="A1-position-X" class="DigNum (strict)"() -> (error out=w1338:errorcluster, "Value"=w1345:dbl)  [unwired: 2 in, 1 out]
                n805 = property on="A1-position-Y" class="DigNum (strict)"(error in=w1338) -> (error out=w1337:errorcluster, "Value"=w1334:dbl)  [unwired: 1 in, 1 out]
                n806 = Subtract(x=w1334, y=9) -> (x-y=w1333:dbl)
                n807 = Subtract(x=w1345, y=27) -> (x-y=w1336:dbl)
                n808 = vi-ref "goto.vi"() -> (w1343:refnum<vi>)
                n809 = property class="VI"(reference=w1343, error in=w1337) -> ("Name"=w1342:string)  [unwired: 2 out]
                n810 = Open VI Reference(type specifier VI Refnum (for type only)=refnum<vi> refnum, vi path=w1342, options=128) -> (vi reference=w1340:refnum<vi>)  [unwired: 3 in, 1 out]
                n811 = call-by-ref "Start Asynchronous Call"(reference=w1340, "Y(mm)"=w1333, "X(mm)"=w1336) -> ()  [unwired: 10 in, 3 out]
              }
            }
          }
          event "C8": Value Change {
            n812 = event-data() -> ("NewVal"=w1347:bool)  [unwired: 1 in, 5 out]
            n813 = property on="移动" class="Bool (strict)"() -> ("Value"=w1350:bool)  [unwired: 2 in, 2 out]
            n814 = Not(x=w1350) -> (.not. x?=w1349:bool)
            n815 = And(x=w1349, y=w1347) -> (x .and. y?=w1348:bool)
            n816 = case shown="True" w1348 {
              frame False {
              }
              frame True {
                n817 = property on="A1-position-X" class="DigNum (strict)"() -> (error out=w1356:errorcluster, "Value"=w1363:dbl)  [unwired: 2 in, 1 out]
                n818 = property on="A1-position-Y" class="DigNum (strict)"(error in=w1356) -> (error out=w1355:errorcluster, "Value"=w1352:dbl)  [unwired: 1 in, 1 out]
                n819 = Subtract(x=w1352, y=9) -> (x-y=w1351:dbl)
                n820 = Subtract(x=w1363, y=31.5) -> (x-y=w1354:dbl)
                n821 = vi-ref "goto.vi"() -> (w1361:refnum<vi>)
                n822 = property class="VI"(reference=w1361, error in=w1355) -> ("Name"=w1360:string)  [unwired: 2 out]
                n823 = Open VI Reference(type specifier VI Refnum (for type only)=refnum<vi> refnum, vi path=w1360, options=128) -> (vi reference=w1358:refnum<vi>)  [unwired: 3 in, 1 out]
                n824 = call-by-ref "Start Asynchronous Call"(reference=w1358, "Y(mm)"=w1351, "X(mm)"=w1354) -> ()  [unwired: 10 in, 3 out]
              }
            }
          }
          event "C9": Value Change {
            n825 = event-data() -> ("NewVal"=w1365:bool)  [unwired: 1 in, 5 out]
            n826 = property on="移动" class="Bool (strict)"() -> ("Value"=w1368:bool)  [unwired: 2 in, 2 out]
            n827 = Not(x=w1368) -> (.not. x?=w1367:bool)
            n828 = And(x=w1367, y=w1365) -> (x .and. y?=w1366:bool)
            n829 = case shown="True" w1366 {
              frame False {
              }
              frame True {
                n830 = property on="A1-position-X" class="DigNum (strict)"() -> (error out=w1374:errorcluster, "Value"=w1381:dbl)  [unwired: 2 in, 1 out]
                n831 = property on="A1-position-Y" class="DigNum (strict)"(error in=w1374) -> (error out=w1373:errorcluster, "Value"=w1370:dbl)  [unwired: 1 in, 1 out]
                n832 = Subtract(x=w1370, y=9) -> (x-y=w1369:dbl)
                n833 = Subtract(x=w1381, y=36) -> (x-y=w1372:dbl)
                n834 = vi-ref "goto.vi"() -> (w1379:refnum<vi>)
                n835 = property class="VI"(reference=w1379, error in=w1373) -> ("Name"=w1378:string)  [unwired: 2 out]
                n836 = Open VI Reference(type specifier VI Refnum (for type only)=refnum<vi> refnum, vi path=w1378, options=128) -> (vi reference=w1376:refnum<vi>)  [unwired: 3 in, 1 out]
                n837 = call-by-ref "Start Asynchronous Call"(reference=w1376, "Y(mm)"=w1369, "X(mm)"=w1372) -> ()  [unwired: 10 in, 3 out]
              }
            }
          }
          event "C10": Value Change {
            n838 = event-data() -> ("NewVal"=w1383:bool)  [unwired: 1 in, 5 out]
            n839 = property on="移动" class="Bool (strict)"() -> ("Value"=w1386:bool)  [unwired: 2 in, 2 out]
            n840 = Not(x=w1386) -> (.not. x?=w1385:bool)
            n841 = And(x=w1385, y=w1383) -> (x .and. y?=w1384:bool)
            n842 = case shown="True" w1384 {
              frame False {
              }
              frame True {
                n843 = property on="A1-position-X" class="DigNum (strict)"() -> (error out=w1392:errorcluster, "Value"=w1399:dbl)  [unwired: 2 in, 1 out]
                n844 = property on="A1-position-Y" class="DigNum (strict)"(error in=w1392) -> (error out=w1391:errorcluster, "Value"=w1388:dbl)  [unwired: 1 in, 1 out]
                n845 = Subtract(x=w1388, y=9) -> (x-y=w1387:dbl)
                n846 = Subtract(x=w1399, y=40.5) -> (x-y=w1390:dbl)
                n847 = vi-ref "goto.vi"() -> (w1397:refnum<vi>)
                n848 = property class="VI"(reference=w1397, error in=w1391) -> ("Name"=w1396:string)  [unwired: 2 out]
                n849 = Open VI Reference(type specifier VI Refnum (for type only)=refnum<vi> refnum, vi path=w1396, options=128) -> (vi reference=w1394:refnum<vi>)  [unwired: 3 in, 1 out]
                n850 = call-by-ref "Start Asynchronous Call"(reference=w1394, "Y(mm)"=w1387, "X(mm)"=w1390) -> ()  [unwired: 10 in, 3 out]
              }
            }
          }
          event "C11": Value Change {
            n851 = event-data() -> ("NewVal"=w1401:bool)  [unwired: 1 in, 5 out]
            n852 = property on="移动" class="Bool (strict)"() -> ("Value"=w1404:bool)  [unwired: 2 in, 2 out]
            n853 = Not(x=w1404) -> (.not. x?=w1403:bool)
            n854 = And(x=w1403, y=w1401) -> (x .and. y?=w1402:bool)
            n855 = case shown="True" w1402 {
              frame False {
              }
              frame True {
                n856 = property on="A1-position-X" class="DigNum (strict)"() -> (error out=w1410:errorcluster, "Value"=w1417:dbl)  [unwired: 2 in, 1 out]
                n857 = property on="A1-position-Y" class="DigNum (strict)"(error in=w1410) -> (error out=w1409:errorcluster, "Value"=w1406:dbl)  [unwired: 1 in, 1 out]
                n858 = Subtract(x=w1406, y=9) -> (x-y=w1405:dbl)
                n859 = Subtract(x=w1417, y=45) -> (x-y=w1408:dbl)
                n860 = vi-ref "goto.vi"() -> (w1415:refnum<vi>)
                n861 = property class="VI"(reference=w1415, error in=w1409) -> ("Name"=w1414:string)  [unwired: 2 out]
                n862 = Open VI Reference(type specifier VI Refnum (for type only)=refnum<vi> refnum, vi path=w1414, options=128) -> (vi reference=w1412:refnum<vi>)  [unwired: 3 in, 1 out]
                n863 = call-by-ref "Start Asynchronous Call"(reference=w1412, "Y(mm)"=w1405, "X(mm)"=w1408) -> ()  [unwired: 10 in, 3 out]
              }
            }
          }
          event "C12": Value Change {
            n864 = event-data() -> ("NewVal"=w1419:bool)  [unwired: 1 in, 5 out]
            n865 = property on="移动" class="Bool (strict)"() -> ("Value"=w1422:bool)  [unwired: 2 in, 2 out]
            n866 = Not(x=w1422) -> (.not. x?=w1421:bool)
            n867 = And(x=w1421, y=w1419) -> (x .and. y?=w1420:bool)
            n868 = case shown="True" w1420 {
              frame False {
              }
              frame True {
                n869 = property on="A1-position-X" class="DigNum (strict)"() -> (error out=w1428:errorcluster, "Value"=w1435:dbl)  [unwired: 2 in, 1 out]
                n870 = property on="A1-position-Y" class="DigNum (strict)"(error in=w1428) -> (error out=w1427:errorcluster, "Value"=w1424:dbl)  [unwired: 1 in, 1 out]
                n871 = Subtract(x=w1424, y=9) -> (x-y=w1423:dbl)
                n872 = Subtract(x=w1435, y=49.5) -> (x-y=w1426:dbl)
                n873 = vi-ref "goto.vi"() -> (w1433:refnum<vi>)
                n874 = property class="VI"(reference=w1433, error in=w1427) -> ("Name"=w1432:string)  [unwired: 2 out]
                n875 = Open VI Reference(type specifier VI Refnum (for type only)=refnum<vi> refnum, vi path=w1432, options=128) -> (vi reference=w1430:refnum<vi>)  [unwired: 3 in, 1 out]
                n876 = call-by-ref "Start Asynchronous Call"(reference=w1430, "Y(mm)"=w1423, "X(mm)"=w1426) -> ()  [unwired: 10 in, 3 out]
              }
            }
          }
          event "D1": Value Change {
            n877 = event-data() -> ("NewVal"=w1437:bool)  [unwired: 1 in, 5 out]
            n878 = property on="移动" class="Bool (strict)"() -> ("Value"=w1440:bool)  [unwired: 2 in, 2 out]
            n879 = Not(x=w1440) -> (.not. x?=w1439:bool)
            n880 = And(x=w1439, y=w1437) -> (x .and. y?=w1438:bool)
            n881 = case shown="True" w1438 {
              frame False {
              }
              frame True {
                n882 = property on="A1-position-X" class="DigNum (strict)"() -> (error out=w1446:errorcluster, "Value"=w1453:dbl)  [unwired: 2 in, 1 out]
                n883 = property on="A1-position-Y" class="DigNum (strict)"(error in=w1446) -> (error out=w1445:errorcluster, "Value"=w1442:dbl)  [unwired: 1 in, 1 out]
                n884 = Subtract(x=w1442, y=13.5) -> (x-y=w1441:dbl)
                n885 = Subtract(x=w1453, y=0) -> (x-y=w1444:dbl)
                n886 = vi-ref "goto.vi"() -> (w1451:refnum<vi>)
                n887 = property class="VI"(reference=w1451, error in=w1445) -> ("Name"=w1450:string)  [unwired: 2 out]
                n888 = Open VI Reference(type specifier VI Refnum (for type only)=refnum<vi> refnum, vi path=w1450, options=128) -> (vi reference=w1448:refnum<vi>)  [unwired: 3 in, 1 out]
                n889 = call-by-ref "Start Asynchronous Call"(reference=w1448, "Y(mm)"=w1441, "X(mm)"=w1444) -> ()  [unwired: 10 in, 3 out]
              }
            }
          }
          event "D2": Value Change {
            n890 = event-data() -> ("NewVal"=w1455:bool)  [unwired: 1 in, 5 out]
            n891 = property on="移动" class="Bool (strict)"() -> ("Value"=w1458:bool)  [unwired: 2 in, 2 out]
            n892 = Not(x=w1458) -> (.not. x?=w1457:bool)
            n893 = And(x=w1457, y=w1455) -> (x .and. y?=w1456:bool)
            n894 = case shown="True" w1456 {
              frame False {
              }
              frame True {
                n895 = property on="A1-position-X" class="DigNum (strict)"() -> (error out=w1464:errorcluster, "Value"=w1471:dbl)  [unwired: 2 in, 1 out]
                n896 = property on="A1-position-Y" class="DigNum (strict)"(error in=w1464) -> (error out=w1463:errorcluster, "Value"=w1460:dbl)  [unwired: 1 in, 1 out]
                n897 = Subtract(x=w1460, y=13.5) -> (x-y=w1459:dbl)
                n898 = Subtract(x=w1471, y=4.5) -> (x-y=w1462:dbl)
                n899 = vi-ref "goto.vi"() -> (w1469:refnum<vi>)
                n900 = property class="VI"(reference=w1469, error in=w1463) -> ("Name"=w1468:string)  [unwired: 2 out]
                n901 = Open VI Reference(type specifier VI Refnum (for type only)=refnum<vi> refnum, vi path=w1468, options=128) -> (vi reference=w1466:refnum<vi>)  [unwired: 3 in, 1 out]
                n902 = call-by-ref "Start Asynchronous Call"(reference=w1466, "Y(mm)"=w1459, "X(mm)"=w1462) -> ()  [unwired: 10 in, 3 out]
              }
            }
          }
          event "D3": Value Change {
            n903 = event-data() -> ("NewVal"=w1473:bool)  [unwired: 1 in, 5 out]
            n904 = property on="移动" class="Bool (strict)"() -> ("Value"=w1476:bool)  [unwired: 2 in, 2 out]
            n905 = Not(x=w1476) -> (.not. x?=w1475:bool)
            n906 = And(x=w1475, y=w1473) -> (x .and. y?=w1474:bool)
            n907 = case shown="True" w1474 {
              frame False {
              }
              frame True {
                n908 = property on="A1-position-X" class="DigNum (strict)"() -> (error out=w1482:errorcluster, "Value"=w1489:dbl)  [unwired: 2 in, 1 out]
                n909 = property on="A1-position-Y" class="DigNum (strict)"(error in=w1482) -> (error out=w1481:errorcluster, "Value"=w1478:dbl)  [unwired: 1 in, 1 out]
                n910 = Subtract(x=w1478, y=13.5) -> (x-y=w1477:dbl)
                n911 = Subtract(x=w1489, y=9) -> (x-y=w1480:dbl)
                n912 = vi-ref "goto.vi"() -> (w1487:refnum<vi>)
                n913 = property class="VI"(reference=w1487, error in=w1481) -> ("Name"=w1486:string)  [unwired: 2 out]
                n914 = Open VI Reference(type specifier VI Refnum (for type only)=refnum<vi> refnum, vi path=w1486, options=128) -> (vi reference=w1484:refnum<vi>)  [unwired: 3 in, 1 out]
                n915 = call-by-ref "Start Asynchronous Call"(reference=w1484, "Y(mm)"=w1477, "X(mm)"=w1480) -> ()  [unwired: 10 in, 3 out]
              }
            }
          }
          event "D4": Value Change {
            n916 = event-data() -> ("NewVal"=w1491:bool)  [unwired: 1 in, 5 out]
            n917 = property on="移动" class="Bool (strict)"() -> ("Value"=w1494:bool)  [unwired: 2 in, 2 out]
            n918 = Not(x=w1494) -> (.not. x?=w1493:bool)
            n919 = And(x=w1493, y=w1491) -> (x .and. y?=w1492:bool)
            n920 = case shown="True" w1492 {
              frame False {
              }
              frame True {
                n921 = property on="A1-position-X" class="DigNum (strict)"() -> (error out=w1500:errorcluster, "Value"=w1507:dbl)  [unwired: 2 in, 1 out]
                n922 = property on="A1-position-Y" class="DigNum (strict)"(error in=w1500) -> (error out=w1499:errorcluster, "Value"=w1496:dbl)  [unwired: 1 in, 1 out]
                n923 = Subtract(x=w1496, y=13.5) -> (x-y=w1495:dbl)
                n924 = Subtract(x=w1507, y=13.5) -> (x-y=w1498:dbl)
                n925 = vi-ref "goto.vi"() -> (w1505:refnum<vi>)
                n926 = property class="VI"(reference=w1505, error in=w1499) -> ("Name"=w1504:string)  [unwired: 2 out]
                n927 = Open VI Reference(type specifier VI Refnum (for type only)=refnum<vi> refnum, vi path=w1504, options=128) -> (vi reference=w1502:refnum<vi>)  [unwired: 3 in, 1 out]
                n928 = call-by-ref "Start Asynchronous Call"(reference=w1502, "Y(mm)"=w1495, "X(mm)"=w1498) -> ()  [unwired: 10 in, 3 out]
              }
            }
          }
          event "D5": Value Change {
            n929 = event-data() -> ("NewVal"=w1509:bool)  [unwired: 1 in, 5 out]
            n930 = property on="移动" class="Bool (strict)"() -> ("Value"=w1512:bool)  [unwired: 2 in, 2 out]
            n931 = Not(x=w1512) -> (.not. x?=w1511:bool)
            n932 = And(x=w1511, y=w1509) -> (x .and. y?=w1510:bool)
            n933 = case shown="True" w1510 {
              frame False {
              }
              frame True {
                n934 = property on="A1-position-X" class="DigNum (strict)"() -> (error out=w1518:errorcluster, "Value"=w1525:dbl)  [unwired: 2 in, 1 out]
                n935 = property on="A1-position-Y" class="DigNum (strict)"(error in=w1518) -> (error out=w1517:errorcluster, "Value"=w1514:dbl)  [unwired: 1 in, 1 out]
                n936 = Subtract(x=w1514, y=13.5) -> (x-y=w1513:dbl)
                n937 = Subtract(x=w1525, y=18) -> (x-y=w1516:dbl)
                n938 = vi-ref "goto.vi"() -> (w1523:refnum<vi>)
                n939 = property class="VI"(reference=w1523, error in=w1517) -> ("Name"=w1522:string)  [unwired: 2 out]
                n940 = Open VI Reference(type specifier VI Refnum (for type only)=refnum<vi> refnum, vi path=w1522, options=128) -> (vi reference=w1520:refnum<vi>)  [unwired: 3 in, 1 out]
                n941 = call-by-ref "Start Asynchronous Call"(reference=w1520, "Y(mm)"=w1513, "X(mm)"=w1516) -> ()  [unwired: 10 in, 3 out]
              }
            }
          }
          event "D6": Value Change {
            n942 = event-data() -> ("NewVal"=w1527:bool)  [unwired: 1 in, 5 out]
            n943 = property on="移动" class="Bool (strict)"() -> ("Value"=w1530:bool)  [unwired: 2 in, 2 out]
            n944 = Not(x=w1530) -> (.not. x?=w1529:bool)
            n945 = And(x=w1529, y=w1527) -> (x .and. y?=w1528:bool)
            n946 = case shown="True" w1528 {
              frame False {
              }
              frame True {
                n947 = property on="A1-position-X" class="DigNum (strict)"() -> (error out=w1536:errorcluster, "Value"=w1543:dbl)  [unwired: 2 in, 1 out]
                n948 = property on="A1-position-Y" class="DigNum (strict)"(error in=w1536) -> (error out=w1535:errorcluster, "Value"=w1532:dbl)  [unwired: 1 in, 1 out]
                n949 = Subtract(x=w1532, y=13.5) -> (x-y=w1531:dbl)
                n950 = Subtract(x=w1543, y=22.5) -> (x-y=w1534:dbl)
                n951 = vi-ref "goto.vi"() -> (w1541:refnum<vi>)
                n952 = property class="VI"(reference=w1541, error in=w1535) -> ("Name"=w1540:string)  [unwired: 2 out]
                n953 = Open VI Reference(type specifier VI Refnum (for type only)=refnum<vi> refnum, vi path=w1540, options=128) -> (vi reference=w1538:refnum<vi>)  [unwired: 3 in, 1 out]
                n954 = call-by-ref "Start Asynchronous Call"(reference=w1538, "Y(mm)"=w1531, "X(mm)"=w1534) -> ()  [unwired: 10 in, 3 out]
              }
            }
          }
          event "D7": Value Change {
            n955 = event-data() -> ("NewVal"=w1545:bool)  [unwired: 1 in, 5 out]
            n956 = property on="移动" class="Bool (strict)"() -> ("Value"=w1548:bool)  [unwired: 2 in, 2 out]
            n957 = Not(x=w1548) -> (.not. x?=w1547:bool)
            n958 = And(x=w1547, y=w1545) -> (x .and. y?=w1546:bool)
            n959 = case shown="True" w1546 {
              frame False {
              }
              frame True {
                n960 = property on="A1-position-X" class="DigNum (strict)"() -> (error out=w1554:errorcluster, "Value"=w1561:dbl)  [unwired: 2 in, 1 out]
                n961 = property on="A1-position-Y" class="DigNum (strict)"(error in=w1554) -> (error out=w1553:errorcluster, "Value"=w1550:dbl)  [unwired: 1 in, 1 out]
                n962 = Subtract(x=w1550, y=13.5) -> (x-y=w1549:dbl)
                n963 = Subtract(x=w1561, y=27) -> (x-y=w1552:dbl)
                n964 = vi-ref "goto.vi"() -> (w1559:refnum<vi>)
                n965 = property class="VI"(reference=w1559, error in=w1553) -> ("Name"=w1558:string)  [unwired: 2 out]
                n966 = Open VI Reference(type specifier VI Refnum (for type only)=refnum<vi> refnum, vi path=w1558, options=128) -> (vi reference=w1556:refnum<vi>)  [unwired: 3 in, 1 out]
                n967 = call-by-ref "Start Asynchronous Call"(reference=w1556, "Y(mm)"=w1549, "X(mm)"=w1552) -> ()  [unwired: 10 in, 3 out]
              }
            }
          }
          event "D8": Value Change {
            n968 = event-data() -> ("NewVal"=w1562:bool)  [unwired: 1 in, 5 out]
            n969 = property on="移动" class="Bool (strict)"() -> ("Value"=w1565:bool)  [unwired: 2 in, 2 out]
            n970 = Not(x=w1565) -> (.not. x?=w1564:bool)
            n971 = And(x=w1564, y=w1562) -> (x .and. y?=w1563:bool)
            n972 = case shown="True" w1563 {
              frame False {
              }
              frame True {
                n973 = property on="A1-position-X" class="DigNum (strict)"() -> (error out=w1572:errorcluster, "Value"=w1579:dbl)  [unwired: 2 in, 1 out]
                n974 = property on="A1-position-Y" class="DigNum (strict)"(error in=w1572) -> (error out=w1571:errorcluster, "Value"=w1568:dbl)  [unwired: 1 in, 1 out]
                n975 = Subtract(x=w1568, y=13.5) -> (x-y=w1567:dbl)
                n976 = Subtract(x=w1579, y=31.5) -> (x-y=w1570:dbl)
                n977 = vi-ref "goto.vi"() -> (w1577:refnum<vi>)
                n978 = property class="VI"(reference=w1577, error in=w1571) -> ("Name"=w1576:string)  [unwired: 2 out]
                n979 = Open VI Reference(type specifier VI Refnum (for type only)=refnum<vi> refnum, vi path=w1576, options=128) -> (vi reference=w1574:refnum<vi>)  [unwired: 3 in, 1 out]
                n980 = call-by-ref "Start Asynchronous Call"(reference=w1574, "Y(mm)"=w1567, "X(mm)"=w1570) -> ()  [unwired: 10 in, 3 out]
              }
            }
          }
          event "D9": Value Change {
            n981 = event-data() -> ("NewVal"=w1580:bool)  [unwired: 1 in, 5 out]
            n982 = property on="移动" class="Bool (strict)"() -> ("Value"=w1583:bool)  [unwired: 2 in, 2 out]
            n983 = Not(x=w1583) -> (.not. x?=w1582:bool)
            n984 = And(x=w1582, y=w1580) -> (x .and. y?=w1581:bool)
            n985 = case shown="True" w1581 {
              frame False {
              }
              frame True {
                n986 = property on="A1-position-X" class="DigNum (strict)"() -> (error out=w1590:errorcluster, "Value"=w1597:dbl)  [unwired: 2 in, 1 out]
                n987 = property on="A1-position-Y" class="DigNum (strict)"(error in=w1590) -> (error out=w1589:errorcluster, "Value"=w1586:dbl)  [unwired: 1 in, 1 out]
                n988 = Subtract(x=w1586, y=13.5) -> (x-y=w1585:dbl)
                n989 = Subtract(x=w1597, y=36) -> (x-y=w1588:dbl)
                n990 = vi-ref "goto.vi"() -> (w1595:refnum<vi>)
                n991 = property class="VI"(reference=w1595, error in=w1589) -> ("Name"=w1594:string)  [unwired: 2 out]
                n992 = Open VI Reference(type specifier VI Refnum (for type only)=refnum<vi> refnum, vi path=w1594, options=128) -> (vi reference=w1592:refnum<vi>)  [unwired: 3 in, 1 out]
                n993 = call-by-ref "Start Asynchronous Call"(reference=w1592, "Y(mm)"=w1585, "X(mm)"=w1588) -> ()  [unwired: 10 in, 3 out]
              }
            }
          }
          event "D10": Value Change {
            n994 = event-data() -> ("NewVal"=w1598:bool)  [unwired: 1 in, 5 out]
            n995 = property on="移动" class="Bool (strict)"() -> ("Value"=w1601:bool)  [unwired: 2 in, 2 out]
            n996 = Not(x=w1601) -> (.not. x?=w1600:bool)
            n997 = And(x=w1600, y=w1598) -> (x .and. y?=w1599:bool)
            n998 = case shown="True" w1599 {
              frame False {
              }
              frame True {
                n999 = property on="A1-position-X" class="DigNum (strict)"() -> (error out=w1608:errorcluster, "Value"=w1615:dbl)  [unwired: 2 in, 1 out]
                n1000 = property on="A1-position-Y" class="DigNum (strict)"(error in=w1608) -> (error out=w1607:errorcluster, "Value"=w1604:dbl)  [unwired: 1 in, 1 out]
                n1001 = Subtract(x=w1604, y=13.5) -> (x-y=w1603:dbl)
                n1002 = Subtract(x=w1615, y=40.5) -> (x-y=w1606:dbl)
                n1003 = vi-ref "goto.vi"() -> (w1613:refnum<vi>)
                n1004 = property class="VI"(reference=w1613, error in=w1607) -> ("Name"=w1612:string)  [unwired: 2 out]
                n1005 = Open VI Reference(type specifier VI Refnum (for type only)=refnum<vi> refnum, vi path=w1612, options=128) -> (vi reference=w1610:refnum<vi>)  [unwired: 3 in, 1 out]
                n1006 = call-by-ref "Start Asynchronous Call"(reference=w1610, "Y(mm)"=w1603, "X(mm)"=w1606) -> ()  [unwired: 10 in, 3 out]
              }
            }
          }
          event "D11": Value Change {
            n1007 = event-data() -> ("NewVal"=w1616:bool)  [unwired: 1 in, 5 out]
            n1008 = property on="移动" class="Bool (strict)"() -> ("Value"=w1619:bool)  [unwired: 2 in, 2 out]
            n1009 = Not(x=w1619) -> (.not. x?=w1618:bool)
            n1010 = And(x=w1618, y=w1616) -> (x .and. y?=w1617:bool)
            n1011 = case shown="True" w1617 {
              frame False {
              }
              frame True {
                n1012 = property on="A1-position-X" class="DigNum (strict)"() -> (error out=w1626:errorcluster, "Value"=w1633:dbl)  [unwired: 2 in, 1 out]
                n1013 = property on="A1-position-Y" class="DigNum (strict)"(error in=w1626) -> (error out=w1625:errorcluster, "Value"=w1622:dbl)  [unwired: 1 in, 1 out]
                n1014 = Subtract(x=w1622, y=13.5) -> (x-y=w1621:dbl)
                n1015 = Subtract(x=w1633, y=45) -> (x-y=w1624:dbl)
                n1016 = vi-ref "goto.vi"() -> (w1631:refnum<vi>)
                n1017 = property class="VI"(reference=w1631, error in=w1625) -> ("Name"=w1630:string)  [unwired: 2 out]
                n1018 = Open VI Reference(type specifier VI Refnum (for type only)=refnum<vi> refnum, vi path=w1630, options=128) -> (vi reference=w1628:refnum<vi>)  [unwired: 3 in, 1 out]
                n1019 = call-by-ref "Start Asynchronous Call"(reference=w1628, "Y(mm)"=w1621, "X(mm)"=w1624) -> ()  [unwired: 10 in, 3 out]
              }
            }
          }
          event "D12": Value Change {
            n1020 = event-data() -> ("NewVal"=w1634:bool)  [unwired: 1 in, 5 out]
            n1021 = property on="移动" class="Bool (strict)"() -> ("Value"=w1637:bool)  [unwired: 2 in, 2 out]
            n1022 = Not(x=w1637) -> (.not. x?=w1636:bool)
            n1023 = And(x=w1636, y=w1634) -> (x .and. y?=w1635:bool)
            n1024 = case shown="True" w1635 {
              frame False {
              }
              frame True {
                n1025 = property on="A1-position-X" class="DigNum (strict)"() -> (error out=w1644:errorcluster, "Value"=w1651:dbl)  [unwired: 2 in, 1 out]
                n1026 = property on="A1-position-Y" class="DigNum (strict)"(error in=w1644) -> (error out=w1643:errorcluster, "Value"=w1640:dbl)  [unwired: 1 in, 1 out]
                n1027 = Subtract(x=w1640, y=13.5) -> (x-y=w1639:dbl)
                n1028 = Subtract(x=w1651, y=49.5) -> (x-y=w1642:dbl)
                n1029 = vi-ref "goto.vi"() -> (w1649:refnum<vi>)
                n1030 = property class="VI"(reference=w1649, error in=w1643) -> ("Name"=w1648:string)  [unwired: 2 out]
                n1031 = Open VI Reference(type specifier VI Refnum (for type only)=refnum<vi> refnum, vi path=w1648, options=128) -> (vi reference=w1646:refnum<vi>)  [unwired: 3 in, 1 out]
                n1032 = call-by-ref "Start Asynchronous Call"(reference=w1646, "Y(mm)"=w1639, "X(mm)"=w1642) -> ()  [unwired: 10 in, 3 out]
              }
            }
          }
          event "E1": Value Change {
            n1033 = event-data() -> ("NewVal"=w1652:bool)  [unwired: 1 in, 5 out]
            n1034 = property on="移动" class="Bool (strict)"() -> ("Value"=w1655:bool)  [unwired: 2 in, 2 out]
            n1035 = Not(x=w1655) -> (.not. x?=w1654:bool)
            n1036 = And(x=w1654, y=w1652) -> (x .and. y?=w1653:bool)
            n1037 = case shown="True" w1653 {
              frame False {
              }
              frame True {
                n1038 = property on="A1-position-X" class="DigNum (strict)"() -> (error out=w1662:errorcluster, "Value"=w1669:dbl)  [unwired: 2 in, 1 out]
                n1039 = property on="A1-position-Y" class="DigNum (strict)"(error in=w1662) -> (error out=w1661:errorcluster, "Value"=w1658:dbl)  [unwired: 1 in, 1 out]
                n1040 = Subtract(x=w1658, y=18.0) -> (x-y=w1657:dbl)
                n1041 = Subtract(x=w1669, y=0) -> (x-y=w1660:dbl)
                n1042 = vi-ref "goto.vi"() -> (w1667:refnum<vi>)
                n1043 = property class="VI"(reference=w1667, error in=w1661) -> ("Name"=w1666:string)  [unwired: 2 out]
                n1044 = Open VI Reference(type specifier VI Refnum (for type only)=refnum<vi> refnum, vi path=w1666, options=128) -> (vi reference=w1664:refnum<vi>)  [unwired: 3 in, 1 out]
                n1045 = call-by-ref "Start Asynchronous Call"(reference=w1664, "Y(mm)"=w1657, "X(mm)"=w1660) -> ()  [unwired: 10 in, 3 out]
              }
            }
          }
          event "E2": Value Change {
            n1046 = event-data() -> ("NewVal"=w1670:bool)  [unwired: 1 in, 5 out]
            n1047 = property on="移动" class="Bool (strict)"() -> ("Value"=w1673:bool)  [unwired: 2 in, 2 out]
            n1048 = Not(x=w1673) -> (.not. x?=w1672:bool)
            n1049 = And(x=w1672, y=w1670) -> (x .and. y?=w1671:bool)
            n1050 = case shown="True" w1671 {
              frame False {
              }
              frame True {
                n1051 = property on="A1-position-X" class="DigNum (strict)"() -> (error out=w1680:errorcluster, "Value"=w1687:dbl)  [unwired: 2 in, 1 out]
                n1052 = property on="A1-position-Y" class="DigNum (strict)"(error in=w1680) -> (error out=w1679:errorcluster, "Value"=w1676:dbl)  [unwired: 1 in, 1 out]
                n1053 = Subtract(x=w1676, y=18.0) -> (x-y=w1675:dbl)
                n1054 = Subtract(x=w1687, y=4.5) -> (x-y=w1678:dbl)
                n1055 = vi-ref "goto.vi"() -> (w1685:refnum<vi>)
                n1056 = property class="VI"(reference=w1685, error in=w1679) -> ("Name"=w1684:string)  [unwired: 2 out]
                n1057 = Open VI Reference(type specifier VI Refnum (for type only)=refnum<vi> refnum, vi path=w1684, options=128) -> (vi reference=w1682:refnum<vi>)  [unwired: 3 in, 1 out]
                n1058 = call-by-ref "Start Asynchronous Call"(reference=w1682, "Y(mm)"=w1675, "X(mm)"=w1678) -> ()  [unwired: 10 in, 3 out]
              }
            }
          }
          event "E3": Value Change {
            n1059 = event-data() -> ("NewVal"=w1688:bool)  [unwired: 1 in, 5 out]
            n1060 = property on="移动" class="Bool (strict)"() -> ("Value"=w1691:bool)  [unwired: 2 in, 2 out]
            n1061 = Not(x=w1691) -> (.not. x?=w1690:bool)
            n1062 = And(x=w1690, y=w1688) -> (x .and. y?=w1689:bool)
            n1063 = case shown="True" w1689 {
              frame False {
              }
              frame True {
                n1064 = property on="A1-position-X" class="DigNum (strict)"() -> (error out=w1698:errorcluster, "Value"=w1705:dbl)  [unwired: 2 in, 1 out]
                n1065 = property on="A1-position-Y" class="DigNum (strict)"(error in=w1698) -> (error out=w1697:errorcluster, "Value"=w1694:dbl)  [unwired: 1 in, 1 out]
                n1066 = Subtract(x=w1694, y=18.0) -> (x-y=w1693:dbl)
                n1067 = Subtract(x=w1705, y=9) -> (x-y=w1696:dbl)
                n1068 = vi-ref "goto.vi"() -> (w1703:refnum<vi>)
                n1069 = property class="VI"(reference=w1703, error in=w1697) -> ("Name"=w1702:string)  [unwired: 2 out]
                n1070 = Open VI Reference(type specifier VI Refnum (for type only)=refnum<vi> refnum, vi path=w1702, options=128) -> (vi reference=w1700:refnum<vi>)  [unwired: 3 in, 1 out]
                n1071 = call-by-ref "Start Asynchronous Call"(reference=w1700, "Y(mm)"=w1693, "X(mm)"=w1696) -> ()  [unwired: 10 in, 3 out]
              }
            }
          }
          event "E4": Value Change {
            n1072 = event-data() -> ("NewVal"=w1706:bool)  [unwired: 1 in, 5 out]
            n1073 = property on="移动" class="Bool (strict)"() -> ("Value"=w1709:bool)  [unwired: 2 in, 2 out]
            n1074 = Not(x=w1709) -> (.not. x?=w1708:bool)
            n1075 = And(x=w1708, y=w1706) -> (x .and. y?=w1707:bool)
            n1076 = case shown="True" w1707 {
              frame False {
              }
              frame True {
                n1077 = property on="A1-position-X" class="DigNum (strict)"() -> (error out=w1716:errorcluster, "Value"=w1723:dbl)  [unwired: 2 in, 1 out]
                n1078 = property on="A1-position-Y" class="DigNum (strict)"(error in=w1716) -> (error out=w1715:errorcluster, "Value"=w1712:dbl)  [unwired: 1 in, 1 out]
                n1079 = Subtract(x=w1712, y=18.0) -> (x-y=w1711:dbl)
                n1080 = Subtract(x=w1723, y=13.5) -> (x-y=w1714:dbl)
                n1081 = vi-ref "goto.vi"() -> (w1721:refnum<vi>)
                n1082 = property class="VI"(reference=w1721, error in=w1715) -> ("Name"=w1720:string)  [unwired: 2 out]
                n1083 = Open VI Reference(type specifier VI Refnum (for type only)=refnum<vi> refnum, vi path=w1720, options=128) -> (vi reference=w1718:refnum<vi>)  [unwired: 3 in, 1 out]
                n1084 = call-by-ref "Start Asynchronous Call"(reference=w1718, "Y(mm)"=w1711, "X(mm)"=w1714) -> ()  [unwired: 10 in, 3 out]
              }
            }
          }
          event "E5": Value Change {
            n1085 = event-data() -> ("NewVal"=w1724:bool)  [unwired: 1 in, 5 out]
            n1086 = property on="移动" class="Bool (strict)"() -> ("Value"=w1727:bool)  [unwired: 2 in, 2 out]
            n1087 = Not(x=w1727) -> (.not. x?=w1726:bool)
            n1088 = And(x=w1726, y=w1724) -> (x .and. y?=w1725:bool)
            n1089 = case shown="True" w1725 {
              frame False {
              }
              frame True {
                n1090 = property on="A1-position-X" class="DigNum (strict)"() -> (error out=w1734:errorcluster, "Value"=w1741:dbl)  [unwired: 2 in, 1 out]
                n1091 = property on="A1-position-Y" class="DigNum (strict)"(error in=w1734) -> (error out=w1733:errorcluster, "Value"=w1730:dbl)  [unwired: 1 in, 1 out]
                n1092 = Subtract(x=w1730, y=18.0) -> (x-y=w1729:dbl)
                n1093 = Subtract(x=w1741, y=18) -> (x-y=w1732:dbl)
                n1094 = vi-ref "goto.vi"() -> (w1739:refnum<vi>)
                n1095 = property class="VI"(reference=w1739, error in=w1733) -> ("Name"=w1738:string)  [unwired: 2 out]
                n1096 = Open VI Reference(type specifier VI Refnum (for type only)=refnum<vi> refnum, vi path=w1738, options=128) -> (vi reference=w1736:refnum<vi>)  [unwired: 3 in, 1 out]
                n1097 = call-by-ref "Start Asynchronous Call"(reference=w1736, "Y(mm)"=w1729, "X(mm)"=w1732) -> ()  [unwired: 10 in, 3 out]
              }
            }
          }
          event "E6": Value Change {
            n1098 = event-data() -> ("NewVal"=w1742:bool)  [unwired: 1 in, 5 out]
            n1099 = property on="移动" class="Bool (strict)"() -> ("Value"=w1745:bool)  [unwired: 2 in, 2 out]
            n1100 = Not(x=w1745) -> (.not. x?=w1744:bool)
            n1101 = And(x=w1744, y=w1742) -> (x .and. y?=w1743:bool)
            n1102 = case shown="True" w1743 {
              frame False {
              }
              frame True {
                n1103 = property on="A1-position-X" class="DigNum (strict)"() -> (error out=w1752:errorcluster, "Value"=w1759:dbl)  [unwired: 2 in, 1 out]
                n1104 = property on="A1-position-Y" class="DigNum (strict)"(error in=w1752) -> (error out=w1751:errorcluster, "Value"=w1748:dbl)  [unwired: 1 in, 1 out]
                n1105 = Subtract(x=w1748, y=18.0) -> (x-y=w1747:dbl)
                n1106 = Subtract(x=w1759, y=22.5) -> (x-y=w1750:dbl)
                n1107 = vi-ref "goto.vi"() -> (w1757:refnum<vi>)
                n1108 = property class="VI"(reference=w1757, error in=w1751) -> ("Name"=w1756:string)  [unwired: 2 out]
                n1109 = Open VI Reference(type specifier VI Refnum (for type only)=refnum<vi> refnum, vi path=w1756, options=128) -> (vi reference=w1754:refnum<vi>)  [unwired: 3 in, 1 out]
                n1110 = call-by-ref "Start Asynchronous Call"(reference=w1754, "Y(mm)"=w1747, "X(mm)"=w1750) -> ()  [unwired: 10 in, 3 out]
              }
            }
          }
          event "ShutDownSystem": Value Change {
            n1111 = event-data() -> ("NewVal"=w1762:bool)  [unwired: 1 in, 5 out]
            n1112 = case shown="True" w1762 {
              tunnel: w1761 -> [_ w1766]
              frame False {
              }
              frame True {
                n1113 = Unbundle By Name(w1766) -> ("ConfiguredPumpCom"=w1765:refnum<visa-resource-name>, "ConfiguredLaserCom"=w1764:refnum<visa-resource-name>)
                n1114 = VISA Close(VISA resource name=w1765) -> (error out=w1763:errorcluster)  [unwired: 1 in]
                n1115 = VISA Close(VISA resource name=w1764, error in (no error)=w1763) -> ()  [unwired: 1 out]
              }
            }
          }
        }
      }
      n1116 = while {
        tunnel: w91 -> [w97]
        stop <- FALSE stop-if-true
        n1117 = event shown="[2] <motor status>: User Event" {
          selector: w97 -> [_ _ _ _]
          dyn-events: _ -> [_ _ _ _]
          timeout: _ -> [_ _ _ _]
          event Timeout {
            n1118 = event-data() -> ()  [unwired: 1 in, 3 out]
          }
          event User Event {
            n1119 = event-data() -> ("AI"=w99:dbl[], "DI"=w98:bool[])  [unwired: 1 in, 4 out]
            n1120 = Index Array(array=w99, index=0) -> (element=w117:dbl)
            n1121 = Index Array(array=w98, index=0) -> (element=→"X0":bool)
            n1122 = Divide(x=w117, y=10.0) -> (x/y=w119:dbl)
            n1123 = Multiply(x=w119, y=2000.0) -> (x*y=w121:dbl)
            n1124 = property on="MCPHV-Real" class="DigNum (strict)"("Value"=w121) -> (error out=w100:errorcluster)  [unwired: 2 in, 1 out]
            n1125 = Index Array(array=w98, index=4) -> (element=→"Y0":bool)
            n1126 = Index Array(array=w99, index=1) -> (element=w122:dbl)
            n1127 = Divide(x=w122, y=10.0) -> (x/y=w124:dbl)
            n1128 = Multiply(x=w124, y=20000.0) -> (x*y=w126:dbl)
            n1129 = Index Array(array=w98, index=1) -> (element=→"X满":bool)
            n1130 = property on="Tar.HV-Real" class="DigNum (strict)"(error in=w100, "Value"=w126) -> (error out=w101:errorcluster)  [unwired: 1 in, 1 out]
            n1131 = Index Array(array=w99, index=2) -> (element=w127:dbl)
            n1132 = Index Array(array=w98, index=3) -> (element=→"Y标":bool)
            n1133 = Divide(x=w127, y=10.0) -> (x/y=w129:dbl)
            n1134 = Multiply(x=w129, y=2000.0) -> (x*y=w131:dbl)
            n1135 = property on="Pul.HV-Real" class="DigNum (strict)"(error in=w101, "Value"=w131) -> (error out=w102:errorcluster)  [unwired: 1 in, 1 out]
            n1136 = Index Array(array=w99, index=3) -> (element=w132:dbl)
            n1137 = Index Array(array=w98, index=2) -> (element=→"Y满":bool)
            n1138 = Divide(x=w132, y=10.0) -> (x/y=w134:dbl)
            n1139 = Multiply(x=w134, y=10000.0) -> (x*y=w136:dbl)
            n1140 = property on="LensHV-Real" class="DigNum (strict)"(error in=w102, "Value"=w136) -> (error out=w138:errorcluster)  [unwired: 1 in, 1 out]
            n1141 = Index Array(array=w99, index=19) -> (element=w140:dbl)
            n1142 = Subtract(x=w140, y=3.572) -> (x-y=w142:dbl)
            n1143 = Divide(x=w142, y=1.286) -> (x/y=w144:dbl)
            n1144 = Power Of 10(x=w144) -> (10^x=w145:dbl)
            n1145 = Index Array(array=w99, index=18) -> (element=w146:dbl)
            n1146 = Subtract(x=w146, y=8.5) -> (x-y=w148:dbl)
            n1147 = property on="Lvaccum" class="DigNum (strict)"(error in=w138, "Value"=w145) -> (error out=w150:errorcluster)  [unwired: 1 in, 1 out]
            n1148 = Power Of 10(x=w148) -> (10^x=w149:dbl)
            n1149 = property on="Hvaccum" class="DigNum (strict)"(error in=w150, "Value"=w149) -> ()  [unwired: 1 in, 2 out]
          }
          event User Event {
            n1150 = event-data() -> ("status"=w151:string)  [unwired: 1 in, 5 out]
            n1151 = case shown="\"moving\"" w151 {
              frame "stop", Default {
                n1152 = property on="GO" class="Bool (strict)"("DisabledEnum"=T10."Enabled" ("Disabled")) -> (error out=w153:errorcluster)  [unwired: 2 in, 1 out]
                n1153 = property on="移动" class="Bool (strict)"(error in=w153, "Value"=FALSE ("移动")) -> ()  [unwired: 1 in, 2 out]
              }
              frame "moving" {
                n1154 = property on="GO" class="Bool (strict)"("DisabledEnum"=T10."Disabled and Grayed Out" ("Disabled")) -> (error out=w156:errorcluster)  [unwired: 2 in, 1 out]
                n1155 = property on="移动" class="Bool (strict)"(error in=w156, "Value"=TRUE ("移动")) -> ()  [unwired: 1 in, 2 out]
              }
            }
          }
          event User Event {
            n1156 = event-data() -> ("source"=w158:string, "value"=w159:dbl)  [unwired: 1 in, 4 out]
            n1157 = case shown="\"X\"" w158 {
              tunnel: w159 -> [w166 w174]
              tunnel: [w168 w175] -> w165
              frame "Y", Default {
                n1158 = property on="X当前" class="DigNum (strict)"() -> ("Value"=w170:dbl)  [unwired: 2 in, 2 out]
                n1159 = Multiply(x=w166, y=1000.0) -> (x*y=w171:dbl)
                n1160 = Divide(x=w170, y=1000.0) -> (x/y=w167:dbl)
                n1161 = Build Array "Build Array"(w167, w166) -> (w168:dbl[])
                n1162 = property on="Y当前" class="DigNum (strict)"("Value"=w171) -> ()  [unwired: 2 in, 2 out]
              }
              frame "X" {
                n1163 = property on="Y当前" class="DigNum (strict)"() -> ("Value"=w177:dbl)  [unwired: 2 in, 2 out]
                n1164 = Multiply(x=w174, y=1000.0) -> (x*y=w178:dbl)
                n1165 = Divide(x=w177, y=1000.0) -> (x/y=w173:dbl)
                n1166 = property on="X当前" class="DigNum (strict)"("Value"=w178) -> ()  [unwired: 2 in, 2 out]
                n1167 = Build Array(w174, w173) -> (w175:dbl[])
              }
            }
            n1168 = Current VI's Path() -> (path=w162:path)
            n1169 = Strip Path(path=w162) -> (stripped path=w163:path)  [unwired: 1 out]
            n1170 = Build Path(base path=w163, name or relative path="last_position") -> (appended path=w161:path)
            n1171 = call-poly <vilib>:"Write To Spreadsheet File.vi"("format (%.3f)"="%.9f", "1D data"=w165, "file path (dialog if empty)"=w161) -> ()  [unwired: 5 in, 1 out]
          }
        }
      }
    }
  }
  n1172 = Unbundle(w23) -> ("tasks"=w4:T13, "interface"=w3:T12, "error out"=w2:errorcluster)
  n1173 = call "USB6343_Control_v1.6.2.vi"("error in"=w2, "interface"=w3, "tasks"=w4) -> ()  [unwired: 9 in]
  n1174 = call <vilib>:"IMAQdx Enumerate Cameras.vi"() -> ("error out"=w13:errorcluster, "Camera Information Array"=w10:T18)  [unwired: 10 in]
  n1175 = while {
    tunnel: w25 -> [w1788]
    tunnel: w24 -> [w1786]
    stop <- FALSE stop-if-true
    n1176 = Unbundle By Name(w1788) -> ("pump semaphore"=w1787:T3, "laser semaphore"=w1783:T3)
    n1177 = Unbundle By Name(w1786) -> ("ConfiguredPumpCom"=w1785:refnum<visa-resource-name>, "ConfiguredLaserCom"=w1773:refnum<visa-resource-name>)
    n1178 = call <vilib>:"Acquire Semaphore.vi"("semaphore"=w1787) -> ("error out"=w1772:errorcluster, "semaphore out"=w1784:T3)  [unwired: 4 in, 1 out]
    n1179 = call "pumpStatus.vi"("VISA resource name"=w1785, "error in (no error)"=w1772) -> ("PumpKW"=→"PumpKW":dbl, "PumpTemp"=→"PumpTemp":u16, "PumpAmps"=→"PumpAmps":dbl, "PumpVolts"=→"PumpVolts":dbl, "TurboSpeed"=→"TurboSpeed":dbl, "error out"=w1771:errorcluster)  [unwired: 8 in]
    n1180 = call <vilib>:"Release Semaphore.vi"("error in (no error)"=w1771, "semaphore"=w1784) -> ("error out"=w1769:errorcluster)  [unwired: 4 in, 1 out]
    n1181 = call <vilib>:"Acquire Semaphore.vi"("error in (no error)"=w1769, "semaphore"=w1783) -> ("error out"=w1770:errorcluster, "semaphore out"=w1768:T3)  [unwired: 3 in, 1 out]
    n1182 = call "Laser-Get-Shotstatus.vi"("VISA resource name"=w1773, "error in (no error)"=w1770) -> ("cluster"=→"cluster":T7, "error out"=w1767:errorcluster)  [unwired: 1 out]
    n1183 = call <vilib>:"Release Semaphore.vi"("error in (no error)"=w1767, "semaphore"=w1768) -> ("error out"=w1782:errorcluster)  [unwired: 4 in, 1 out]
    n1184 = call "Time Delay2"("error in (no error)"=w1782, "Delay Time (s)"=1.0) -> ()  [unwired: 9 in, 1 out]
  }
  n1185 = Index Array(array=w10, index=0) -> (element=w12:T19)
  n1186 = Unbundle By Name(w12) -> ("InterfaceName"=w20:string)
  n1187 = call <vilib>:"IMAQdx Open Camera.vi"("error in"=w13, "Session In"=w20) -> ("error out"=w7:errorcluster, "Session Out"=w8:T20)  [unwired: 8 in]
  n1188 = property class="IMAQdx" props=["VideoMode", "Width", "Height"](reference=w8, error in=w7, "VideoMode"=u32 13) -> (reference out=w6:T20, error out=w5:errorcluster)  [unwired: 2 out]
  n1189 = call "IMAQ Create"("Image Name"=w20) -> ("New Image"=w15:T2)  [unwired: 4 in, 1 out]
  n1190 = call <vilib>:"IMAQdx Configure Grab.vi"("error in"=w5, "Session In"=w6) -> ("error out"=w19:errorcluster, "Session Out"=w14:T20)  [unwired: 8 in]
  n1191 = while {
    tunnel: w19 -> [w1795]
    tunnel: w14 -> [w1794]
    tunnel: w15 -> [w1793]
    tunnel: [w1792] -> w16
    tunnel: [w1791] -> w17
    tunnel: [w1790] -> w18
    stop <- FALSE stop-if-true
    n1192 = call <vilib>:"IMAQdx Grab.vi"("error in"=w1795, "Image In"=w1793, "Session In"=w1794) -> ("error out"=w1792:errorcluster, "Image Out"=w1790:T2, "Session Out"=w1791:T20)  [unwired: 5 in, 1 out]
    "Image" <- w1790
  }
  n1193 = call "IMAQ Dispose"("Image"=w18) -> ()  [unwired: 5 in, 1 out]
  n1194 = call <vilib>:"IMAQdx Close Camera.vi"("error in"=w16, "Session In"=w17) -> ()  [unwired: 9 in, 1 out]
